vi "SBND_TST_p1_adc_1117.vi"() -> ()   [LabVIEW 2015]
uses:
  E:/P1_ADC_TEST_2017/LabVIEW_1130/LBNE_DLL/LBNE_DLL/bin/Debug/LBNE_DLL.dll
  <vilib>/Analysis/baseanly.llb/Mean (DBL).vi
  LBNE_Global .vi
  <vilib>/express/express analysis/Spectral/Block/exnSpectralBlock spectral measurements power poly.vi
  <vilib>/express/express analysis/Spectral/Block/exnSpectralBlock spectral measurements power DDT.vi
  <vilib>/express/express analysis/Spectral/XNode/ExpressSpectralMeasurementsBlockNode.xnode
  <vilib>/Analysis/NI_AAL_SigProc.lvlib
  <vilib>/Analysis/NI_AALBase.lvlib
panel:
  out "20":u16=100
  out "33":u16=3
  out "32":u16=10
  out "31":u16=90
  out "30":u16=32
  out "29":u16=10
  out "28":u16=10
  out "27":u16=90
  out "26":u16=60
  out "25":u16=40
  out "24":u16=6
  out "23":u16=92
  out "22":u16=12
  out "21":u16
  out "(hi.lo)":u16 format="%x"
  out "array":bool[](array[boolean])=[TRUE, FALSE, FALSE, TRUE, FALSE, FALSE, FALSE, FALSE]
  out "FE RB":u32[](array[numeric])=[4294901760, 4294901760, 4294901760, 4294901760, 4294901760, 4294901760, 4294901760, 4294901760, 4294901760, 4294901760, 4294901760, 4294901760, 4294901760, 4294901760, 4294901760, 4294901760, 4294901760, 4294901760, 4294901760, 4294901760, 4294901760, 4294901760, 4294901760, 4294901760, 4294901760, 4294901760, 4294901760, 4294901760, 4294901760, 4294901760, 4294901760, 4294901760, 4294901760, 4294901760, 4294901760, 4294901760] format="%x"
  out "FE Input":u32[](array[numeric])=[3503345872, 3503345872, 3503345872, 3503345872, 3503345872, 3503345872, 3503345872, 3503345872, 151062785, 3503345872, 3503345872, 3503345872, 3503345872, 3503345872, 3503345872, 3503345872, 3503345872, 151062785, 3503345872, 3503345872, 3503345872, 3503345872, 3503345872, 3503345872, 3503345872, 3503345872, 151062785, 3503345872, 3503345872, 3503345872, 3503345872, 3503345872, 3503345872, 3503345872, 3503345872, 151062785] format="%x"
  out "ADC RB":u32[](array[numeric])=[514, 514, 514, 514, 514, 514, 514, 514, 37120, 0, 0, 0, 0, 0, 0, 0, 0, 37120, 0, 0, 0, 0, 0, 0, 0, 0, 37120, 0, 0, 0, 0, 0, 0, 0, 0, 37120] format="%x"
  out "ADC  Input":u32[](array[numeric])=[0, 0, 0, 0, 0, 0, 0, 0, 1216366720, 0, 0, 0, 0, 0, 0, 0, 0, 1216366720, 0, 0, 0, 0, 0, 0, 0, 0, 1216366720, 257, 257, 257, 257, 257, 257, 257, 257, 1216366720] format="%x"
  in  "Array 4":T1(array[cluster])=[{"EN_GR"=1, "CLKG"=2, "FRQC"=1, "F2"=0, "F1"=0}, {"EN_GR"=1, "CLKG"=2, "FRQC"=1, "F2"=0, "F1"=0}, {"EN_GR"=1, "CLKG"=2, "FRQC"=1, "F2"=0, "F1"=0}, {"EN_GR"=1, "CLKG"=2, "FRQC"=1, "F2"=0, "F1"=0}, {"EN_GR"=0, "CLKG"=2, "FRQC"=1, "F2"=0, "F1"=0}, {"EN_GR"=0, "CLKG"=2, "FRQC"=1, "F2"=0, "F1"=0}, {"EN_GR"=0, "CLKG"=2, "FRQC"=1, "F2"=0, "F1"=0}, {"EN_GR"=1, "CLKG"=2, "FRQC"=1, "F2"=0, "F1"=0}] {"F1" items=["FIFO write clock is the ADC write clock", "FIFO write clock is on pin IdxMp/n.  "]; "F2" items=["FIFO clock generator off", "FIFO clock generator  on."]; "FRQC" items=["1 MHz", "2 MHz "]; "CLKG" items=["ADC clocks from monostable", "External clocks", "ADC clocks from digital generator of FIFO", "ADC clocks from monostable"]; "EN_GR" items=["Disables offset current absorption", "Enables the offset current absorption"]}
  out "size(s) 3":i32=127
  out "Array 5":dbl[](array[numeric])
  out "setting":u16=141
  out "Time has Elapsed":bool
  in  "y":i32=50
  out "ADC_hist":u32[][](array[numeric])
  out "FF_B_SHFT 2":u32=101058054 format="%x"
  out "TP_RES":u32=39341825
  out "Array 2":u32[](array[numeric])=[3503345872, 3503345872, 3503345872, 3503345872, 3503345872, 3503345872, 3503345872, 3503345872, 151062785, 3503345872, 3503345872, 3503345872, 3503345872, 3503345872, 3503345872, 3503345872, 3503345872, 151062785, 3503345872, 3503345872, 3503345872, 3503345872, 3503345872, 3503345872, 3503345872, 3503345872, 151062785, 3503345872, 3503345872, 3503345872, 3503345872, 3503345872, 3503345872, 3503345872, 3503345872, 151062785] format="%x"
  out "Array":u32[](array[numeric])=[0, 0, 0, 0, 0, 0, 0, 0, 1216366720, 0, 0, 0, 0, 0, 0, 0, 0, 1216366720, 0, 0, 0, 0, 0, 0, 0, 0, 1216366720, 257, 257, 257, 257, 257, 257, 257, 257, 1216366720] format="%x"
  out "FF_B_SHFT":u32=101058056 format="%x"
  in  "stop":bool
  in  "Tab Control":T2(tab)
  in  "Mult":dbl=1.0 format="%#_6p"
  in  "Pulse width(ns)":u32 max=1000000 step=20
  in  "Save":bool
  in  "DAC_MEAS":bool
  out "max value":u32=1719
  in  "RESET 6":bool
  in  "samples 3":i32
  in  "CHANNEL":u8(slide)
  in  "Tab Control 3":enum32{"CLOCK PHASE CONTROL"}(tab)
  in  "DATA SHIFT":u8[](array[numeric])=[8, 6, 6, 6, 6, 6, 6, 6] format="%x"
  in  "ADC_TM EN":bool=TRUE
  in  "TEST PAT":u32=279 format="%x"
  in  "TEST EN":u32 format="%x"
  out "result":u32=2165768192
  in  "ADC  CLK \nPHASE":bool[](array[boolean])=[TRUE, FALSE, FALSE, FALSE, TRUE, FALSE, TRUE, TRUE]
  in  "ASIC/CHN READOUT":bool=TRUE
  in  "number_of_samples":u32=10000
  in  "FREQ":u16=600
  in  "DLY":u8=79
  in  "AMPL":u8=1 format="%x"
  in  "CHIP":u8(slide) scale=0.0..7.0
  in  "STOP_DATA":bool
  in  "AUTO SCALE":bool=TRUE
  in  "x":u32=100
  out "ADC_MEAN":dbl=1719.0
  out "ADC_CNT":u32=37
  out "ADC_PEAK":u32=1719
  out "Waveform Graph 4":u32[](graph)
  out "ADC HIST":dynamicdata(graph)
  out "samples 4":u32=285743519
  out "Waveform Graph 5":u32[](graph)=[1719, 1718, 1719, 1717, 1719, 1717, 1718, 1717, 1718, 1719, 1718, 1717, 1718, 1716, 1717, 1718, 1717, 1717, 1717, 1717, 1718, 1719, 1718, 1717, 1719, 1719, 1719, 1717, 1718, 1717, 1716, 1719, 1718, 1717, 1717, 1719, 1717, 1718, 1717, 1719, 1716, 1718, 1717, 1718, 1717, 1718, 1717, 1718, 1717, 1718]
  in  "length":i32=50 min=10 max=65 step=1
  in  "SYNC":bool
  in  "FILE PATH":path=path "D:/debug_data"
  in  "FILE NAME 2":string="adaf2sd"
  in  "SAVE TO \nFILE":bool
  out "Store_Data":bool
  in  "SYNC 3":bool
  in  "recalu":bool
  out "samples":i32=10001
  in  "IntDAC_ON":bool
  out "x+y":u8=1 format="%b"
  in  "SYNC 2":bool
  in  "pulse_en":bool
  out "INV_REG":u16=3
  in  "invert 5":bool caption="INVERT"
  in  "invert 4":bool caption="invert"
  in  "invert 3":bool caption="invert"
  in  "invert 2":bool=TRUE caption="invert"
  in  "invert":bool=TRUE
  in  "LSB_S_OFF":dbl=4.4999999999999993e-07 caption="OFFSET" min=0.0 max=0.000655 step=1e-08 format="%#_6p"
  in  "LSB_S_WID":dbl=5e-08 caption="WIDTH" min=1e-08 max=0.000655 step=1e-08 format="%#_6p"
  in  "LSB_FC_OFF2":dbl=4.5e-07 caption="OFFSET" min=0.0 max=0.000655 step=1e-08 format="%#_6p"
  in  "LSB_FC_WID1":dbl=1.6e-07 caption="WIDTH" min=1e-08 max=0.000655 step=1e-08 format="%#_6p"
  in  "RD/EN_WID":dbl=3e-08 caption="WIDTH" min=1e-08 max=0.000655 step=1e-08 format="%#_6p"
  in  "LSB_FC_OFF1":dbl=5e-08 caption="OFFSET" min=0.0 max=0.000655 step=1e-08 format="%#_6p"
  in  "LSB_FC_WID2":dbl=5e-08 caption="WIDTH" min=1e-08 max=0.000655 step=1e-08 format="%#_6p"
  in  "PERIOD 2":dbl=5e-07 min=1e-08 max=0.000655 step=1e-08 format="%#_6p"
  in  "MSB_WID":dbl=3e-07 caption="WIDTH" min=1e-08 max=0.000655 step=1e-08 format="%#_6p"
  in  "MSB_OFF":dbl=2e-07 caption="OFFSET" min=0.0 max=0.000655 step=1e-08 format="%#_6p"
  in  "ADC_WID":dbl=6e-08 caption="WIDTH" min=1e-08 max=0.000655 step=1e-08 format="%#_6p"
  in  "ADC_OFF":dbl caption="OFFSET" min=0.0 max=0.000655 step=1e-08 format="%#_6p"
  in  "CLOCK":dbl=5e-09 format="%#_6p"
  in  "RD/EN_OFF":dbl=4.6e-07 caption="OFFSET" min=0.0 max=0.000655 step=1e-08 format="%#_6p"
  in  "Setting_ext_clk":bool
  in  "Reset":bool=TRUE
  out "Waveform Graph":dynamicdata(graph)=[{"t0"=timestamp(0 s since 1904-01-01), "dt"=199.98000199980004, "Y"=array[5001 elements], "attributes"=variant("NI_ChannelName"=variant(string "Power Spectrum"))}]
  in  "Boolean":bool=TRUE
  out "Peds Mean":dbl=18.0
  out "Peds_RMS":dbl
  in  "Restart Averaging":bool
  in  "fft save":bool=TRUE
  in  "Start channel":u8
  in  "Start chip":u8
  out "CUR_CHP":u8=8 caption="CHIP"
  out "CUR_CHN":u8 caption="CHANNEL"
  in  "Tab Control 2":enum32{"Page 1", "Page 2", "Page 3"}(tab)=enum."Page 2"
  out "Waveform Graph 6":u32[](graph)=[347, 344, 344, 344, 345, 347, 349, 350, 352, 351, 350, 350, 348, 349, 347, 350, 355, 674, 1968, 3349, 3455, 2112, 1599, 1721, 1728, 2759, 1820, 1126, 725, 547, 534, 612, 755, 755, 767, 750, 720, 699, 682, 677]
  out "ADC_CNT 2":u32=250000
  out "Waveform Graph 7":u32[](graph)
  out "CNT":i32
  in  "number_of_samples 2":u32=10000
  out "peds rms":dbl=13.663892227612275
  out "peds Mean":dbl=966.158
  out "ADC_MEAN 2":dbl=3547.568003950388
  out "ADC_RMS 2":dbl=28.577553542992373
  out "ENC":u32[][](array[numeric])=[[1066, 1158, 1012, 1088, 995, 1035, 1178, 1226, 0, 0, 0, 0, 0, 0, 0, 0], [1189, 1244, 1188, 920, 983, 1182, 1156, 1036, 0, 0, 0, 0, 0, 0, 0, 0], [998, 1190, 1140, 1203, 1082, 1076, 1156, 1019, 0, 0, 0, 0, 0, 0, 0, 0], [1218, 1198, 1231, 1210, 1128, 1046, 1135, 1285, 0, 0, 0, 0, 0, 0, 0, 0], [1111, 1144, 1123, 1107, 1274, 1033, 1249, 1045, 0, 0, 0, 0, 0, 0, 0, 0], [1232, 1074, 1188, 1225, 1224, 1163, 1150, 1045, 0, 0, 0, 0, 0, 0, 0, 0], [1135, 1231, 1161, 1158, 1204, 1187, 1007, 1210, 0, 0, 0, 0, 0, 0, 0, 0], [1167, 1176, 1273, 1200, 1029, 1106, 1193, 1134, 0, 0, 0, 0, 0, 0, 0, 0], [1193, 1078, 1088, 1147, 1057, 1218, 1117, 1152, 0, 0, 0, 0, 0, 0, 0, 0], [1139, 1255, 1171, 1006, 1142, 1231, 1182, 1110, 0, 0, 0, 0, 0, 0, 0, 0], [1022, 1243, 1182, 1152, 1182, 1227, 1034, 1008, 0, 0, 0, 0, 0, 0, 0, 0], [1097, 1118, 1072, 1073, 1076, 1190, 1129, 1021, 0, 0, 0, 0, 0, 0, 0, 0], [1180, 1434, 1174, 1222, 1134, 1076, 983, 961, 0, 0, 0, 0, 0, 0, 0, 0], [1246, 1138, 1204, 1072, 996, 1199, 1170, 1189, 0, 0, 0, 0, 0, 0, 0, 0], [1117, 1221, 1111, 1069, 1076, 1020, 1125, 1307, 0, 0, 0, 0, 0, 0, 0, 0], [1150, 1221, 1017, 1216, 1027, 1131, 1151, 1107, 0, 0, 0, 0, 0, 0, 0, 0]]
  out "RMS":dbl[][](array[numeric])=[[13.158810131795315, 14.299668256349447, 12.492235332772674, 13.434291139405659, 12.283790528144634, 12.773694837415796, 14.542669902822118, 15.129984571856891, 0.0, 0.0, 0.0, 0.0, 0.0, 0.0, 0.0, 0.0], [14.678913424572517, 15.352980350441642, 14.665580703900332, 11.355610563990915, 12.138665292767438, 14.589238842015973, 14.27260740231528, 12.784333020313527, 0.0, 0.0, 0.0, 0.0, 0.0, 0.0, 0.0, 0.0], [12.316104634769772, 14.686169938243747, 14.071507513514494, 14.850335266956211, 13.356531107153144, 13.286305287729014, 14.272524762853365, 12.585939548041432, 0.0, 0.0, 0.0, 0.0, 0.0, 0.0, 0.0, 0.0], [15.031876090654704, 14.78741307663375, 15.197331681388519, 14.942137963142448, 13.92969604991704, 12.916776312026833, 14.017775625421985, 15.861789423517077, 0.0, 0.0, 0.0, 0.0, 0.0, 0.0, 0.0, 0.0], [13.711007977448755, 14.124903893964802, 13.86214292900519, 13.669041429899488, 15.730185376637957, 12.757548988490175, 15.416399526623406, 12.90285640589203, 0.0, 0.0, 0.0, 0.0, 0.0, 0.0, 0.0, 0.0], [15.209968953932732, 13.253351507556122, 14.67011636123585, 15.11890588873142, 15.112163287188801, 14.361479615439631, 14.198048906716979, 12.907182040902331, 0.0, 0.0, 0.0, 0.0, 0.0, 0.0, 0.0, 0.0], [14.00645905304824, 15.192981506088497, 14.334865664637054, 14.29655500081451, 14.863929546227123, 14.648189450000741, 12.433031371901722, 14.93841649736285, 0.0, 0.0, 0.0, 0.0, 0.0, 0.0, 0.0, 0.0], [14.406934492960996, 14.521369254626054, 15.713725148777902, 14.816638937130847, 12.698558733540393, 13.65630718677371, 14.730008604397979, 14.000887735770736, 0.0, 0.0, 0.0, 0.0, 0.0, 0.0, 0.0, 0.0], [14.726953471809923, 13.307153473504258, 13.425939022614743, 14.159111250573732, 13.047276940761495, 15.032795841962947, 13.788303828391248, 14.216588987149647, 0.0, 0.0, 0.0, 0.0, 0.0, 0.0, 0.0, 0.0], [14.060310114619874, 15.497566502140451, 14.45258949361071, 12.414504608398772, 14.093800711961055, 15.193383167000526, 14.591254627573019, 13.700501782581963, 0.0, 0.0, 0.0, 0.0, 0.0, 0.0, 0.0, 0.0], [12.620986613202522, 15.34119284681887, 14.596673335246262, 14.228085214724398, 14.588330975790932, 15.14637178214725, 12.759404023095692, 12.44636167027054, 0.0, 0.0, 0.0, 0.0, 0.0, 0.0, 0.0, 0.0], [13.542240957742603, 13.796521505221467, 13.235895747990849, 13.24595461130884, 13.288907173806308, 14.693371316457617, 13.942789791470513, 12.605823223037053, 0.0, 0.0, 0.0, 0.0, 0.0, 0.0, 0.0, 0.0], [14.567227096150493, 17.700518696569162, 14.499408433524646, 15.089488052632309, 13.99466814342557, 13.28550840471075, 12.138577668930898, 11.868199777665112, 0.0, 0.0, 0.0, 0.0, 0.0, 0.0, 0.0, 0.0], [15.383401089361877, 14.0437627128782, 14.865354796421366, 13.236273748711483, 12.302313129985306, 14.80603646506271, 14.449664788619662, 14.684171701673126, 0.0, 0.0, 0.0, 0.0, 0.0, 0.0, 0.0, 0.0], [13.788793478982793, 15.074520898020795, 13.714749170015086, 13.194651442199076, 13.287129102811642, 12.589358859141534, 13.891878034502772, 16.13217079683144, 0.0, 0.0, 0.0, 0.0, 0.0, 0.0, 0.0, 0.0], [14.194393496869207, 14.58553882593015, 12.561266269833073, 15.01194166987972, 12.684919097973044, 13.95782081566281, 14.211606275556221, 13.663892227612275, 0.0, 0.0, 0.0, 0.0, 0.0, 0.0, 0.0, 0.0]] format="%#_6p"
  out "MEAN":dbl[][](array[numeric])=[[951.324636, 1011.55798, 971.46512, 1001.66468, 968.556052, 972.350264, 982.554388, 977.525348, 0.0, 0.0, 0.0, 0.0, 0.0, 0.0, 0.0, 0.0], [968.791648, 997.257824, 952.538196, 967.293388, 974.391288, 923.371776, 967.966284, 965.50768, 0.0, 0.0, 0.0, 0.0, 0.0, 0.0, 0.0, 0.0], [966.960944, 1017.868124, 981.59792, 999.453604, 946.836188, 936.086336, 945.20444, 959.828888, 0.0, 0.0, 0.0, 0.0, 0.0, 0.0, 0.0, 0.0], [978.26338, 1043.011188, 949.993868, 964.42902, 957.316784, 950.378752, 979.645384, 934.216884, 0.0, 0.0, 0.0, 0.0, 0.0, 0.0, 0.0, 0.0], [929.989036, 1032.178852, 966.136316, 986.937408, 946.225756, 967.610864, 953.010968, 978.696088, 0.0, 0.0, 0.0, 0.0, 0.0, 0.0, 0.0, 0.0], [929.028032, 1024.033592, 975.532416, 969.967212, 946.246792, 962.814236, 963.491192, 925.32462, 0.0, 0.0, 0.0, 0.0, 0.0, 0.0, 0.0, 0.0], [900.810692, 1016.34432, 957.256952, 971.032568, 951.10148, 974.453052, 971.472628, 976.797908, 0.0, 0.0, 0.0, 0.0, 0.0, 0.0, 0.0, 0.0], [904.885524, 1025.378384, 979.768964, 963.671816, 921.32862, 935.616876, 951.336824, 954.797924, 0.0, 0.0, 0.0, 0.0, 0.0, 0.0, 0.0, 0.0], [946.570576, 978.304044, 982.728128, 961.54466, 934.350396, 941.809608, 934.119708, 956.873992, 0.0, 0.0, 0.0, 0.0, 0.0, 0.0, 0.0, 0.0], [944.1745, 1004.2861, 977.463388, 964.074912, 934.10018, 936.20658, 957.856724, 945.618092, 0.0, 0.0, 0.0, 0.0, 0.0, 0.0, 0.0, 0.0], [973.670476, 982.029248, 954.42366, 975.224724, 923.454628, 929.649464, 976.710324, 968.553636, 0.0, 0.0, 0.0, 0.0, 0.0, 0.0, 0.0, 0.0], [965.06046, 898.844772, 965.280992, 974.93758, 917.347224, 921.535312, 966.193304, 960.837284, 0.0, 0.0, 0.0, 0.0, 0.0, 0.0, 0.0, 0.0], [950.01384, 992.454184, 956.749904, 943.244992, 952.055344, 933.469464, 965.61666, 962.037436, 0.0, 0.0, 0.0, 0.0, 0.0, 0.0, 0.0, 0.0], [930.076456, 1022.444884, 969.01946, 944.750212, 957.989368, 920.209564, 958.431424, 951.790124, 0.0, 0.0, 0.0, 0.0, 0.0, 0.0, 0.0, 0.0], [927.998292, 992.330316, 944.414212, 937.281776, 943.311696, 914.253672, 936.52954, 980.55764, 0.0, 0.0, 0.0, 0.0, 0.0, 0.0, 0.0, 0.0], [937.546208, 992.701584, 949.3722, 922.113264, 923.434524, 924.734336, 914.765328, 966.158, 0.0, 0.0, 0.0, 0.0, 0.0, 0.0, 0.0, 0.0]] format="%#_6p"
  out "samples received":i32=260051
  out "Average of all CHNS":dbl=1135.9057710689235
  out "gain electrons":u16=148
  out "FFT Analysis":dynamicdata(graph)=[{"t0"=timestamp(0 s since 1904-01-01), "dt"=400.0, "Y"=array[2500 elements], "attributes"=variant("NI_ChannelName"=variant(string "Power Spectrum"))}]
  in  "START":bool
  in  "FILE PATH 2":path=path "D:/ProtoDUNE_AM3/data0831/RMS"
  in  "FILE NAME 3":string="v6_" caption="FILE NAME 2"
  in  "SAVE TO \nFILE 2":bool
  in  "stop 2":bool
  out "samples 5":u32=261950 caption="SAMPLES"
  out "TP enable":bool
  out "AMPL 2":u8 format="%x"
  out "Store_Data 2":bool
  in  "com":u32=30
  in  "FREQ 2":u16=300
  in  "Caculation":u32=200
  in  "FILE NAME 4":string="FFT_" caption="FFTFILE NAME 2"
  out "loop cnt":i32=18865
  in  "AMPL2 END":i32 format="%x"
  in  "ADC write":bool=TRUE
  in  "DAC  0x00-0x3f":u16 format="%x"
  in  "DAC SW":u16(ring) items=["DISABLE TEST PULSE", "INTERNAL DAC", "EXTERNAL DAC", "DAC OUTPUT"]
  in  "DAC":u16[](array[numeric])=[16, 16, 16, 16, 16, 16, 16, 16] format="%x"
  in  "SW":u16[](array[ring])=[1, 1, 1, 1, 1, 1, 1, 1] items=["DISABLE TEST PULSE", "INTERNAL DAC", "EXTERNAL DAC", "DAC OUTPUT"]
  in  "FE ASIC(DAC)":bool=TRUE
  in  "ALL SET":bool
  in  "s 11":bool=TRUE
  in  "write_string":bool
  out "SDI 2":u16=16 format="%x"
  out "rst":u16=2
  out "cs":u16=4
  out "ck":u16=8
  out "SDI":u16=1
  in  "OK Button 2":bool
  in  "Slide":u8(slide)=3 scale=0.0..7.0
  in  "channel":T3={"sts"=TRUE, "snc"=TRUE, "SG"=2, "ST"=0, "SDC"=FALSE, "SDF"=FALSE} {"ST" items=["1us", "0.5us", "3us", "2us"]; "SG" items=["4.7 mV/fC", "7.8 mV/fC", "14 mV/fC", "25 mV/fC"]}
  in  "CHANNEL 4":T4={"D_offset"=0, "PDSR"=FALSE, "PCSR"=FALSE, "slp"=FALSE, "tst"=TRUE} {"D_offset" items=["0", "1", "2", "3", "4", "5", "6", "7", "8", "9", "10", "11", "12", "13", "14", "15"]}
  in  "QUICK SET":bool
  in  "s 10":bool=TRUE
  in  "s 9":bool=TRUE
  in  "s 8":bool=TRUE
  in  "s 7":bool=TRUE
  in  "s 6":bool=TRUE
  in  "s 5":bool=TRUE
  in  "s 4":bool=TRUE
  in  "s 3":bool=TRUE
  in  "s 2":bool=TRUE
  in  "s":bool=TRUE
  in  "CHANNEL 3":T5(array[cluster])=[[{"D_offset"=0, "PDSR"=FALSE, "PCSR"=FALSE, "slp"=FALSE, "tst"=FALSE}, {"D_offset"=0, "PDSR"=FALSE, "PCSR"=FALSE, "slp"=FALSE, "tst"=FALSE}, {"D_offset"=0, "PDSR"=FALSE, "PCSR"=FALSE, "slp"=FALSE, "tst"=FALSE}, {"D_offset"=0, "PDSR"=FALSE, "PCSR"=FALSE, "slp"=FALSE, "tst"=TRUE}, {"D_offset"=0, "PDSR"=FALSE, "PCSR"=FALSE, "slp"=FALSE, "tst"=FALSE}, {"D_offset"=0, "PDSR"=FALSE, "PCSR"=FALSE, "slp"=FALSE, "tst"=FALSE}, {"D_offset"=0, "PDSR"=FALSE, "PCSR"=FALSE, "slp"=FALSE, "tst"=FALSE}, {"D_offset"=0, "PDSR"=FALSE, "PCSR"=FALSE, "slp"=FALSE, "tst"=FALSE}], [{"D_offset"=0, "PDSR"=FALSE, "PCSR"=FALSE, "slp"=FALSE, "tst"=FALSE}, {"D_offset"=0, "PDSR"=FALSE, "PCSR"=FALSE, "slp"=FALSE, "tst"=FALSE}, {"D_offset"=0, "PDSR"=FALSE, "PCSR"=FALSE, "slp"=FALSE, "tst"=FALSE}, {"D_offset"=0, "PDSR"=FALSE, "PCSR"=FALSE, "slp"=FALSE, "tst"=TRUE}, {"D_offset"=0, "PDSR"=FALSE, "PCSR"=FALSE, "slp"=FALSE, "tst"=FALSE}, {"D_offset"=0, "PDSR"=FALSE, "PCSR"=FALSE, "slp"=FALSE, "tst"=FALSE}, {"D_offset"=0, "PDSR"=FALSE, "PCSR"=FALSE, "slp"=FALSE, "tst"=FALSE}, {"D_offset"=0, "PDSR"=FALSE, "PCSR"=FALSE, "slp"=FALSE, "tst"=FALSE}], [{"D_offset"=0, "PDSR"=FALSE, "PCSR"=FALSE, "slp"=FALSE, "tst"=FALSE}, {"D_offset"=0, "PDSR"=FALSE, "PCSR"=FALSE, "slp"=FALSE, "tst"=FALSE}, {"D_offset"=0, "PDSR"=FALSE, "PCSR"=FALSE, "slp"=FALSE, "tst"=FALSE}, {"D_offset"=0, "PDSR"=FALSE, "PCSR"=FALSE, "slp"=FALSE, "tst"=TRUE}, {"D_offset"=0, "PDSR"=FALSE, "PCSR"=FALSE, "slp"=FALSE, "tst"=FALSE}, {"D_offset"=0, "PDSR"=FALSE, "PCSR"=FALSE, "slp"=FALSE, "tst"=FALSE}, {"D_offset"=0, "PDSR"=FALSE, "PCSR"=FALSE, "slp"=FALSE, "tst"=FALSE}, {"D_offset"=0, "PDSR"=FALSE, "PCSR"=FALSE, "slp"=FALSE, "tst"=FALSE}], [{"D_offset"=0, "PDSR"=FALSE, "PCSR"=FALSE, "slp"=FALSE, "tst"=FALSE}, {"D_offset"=0, "PDSR"=FALSE, "PCSR"=FALSE, "slp"=FALSE, "tst"=FALSE}, {"D_offset"=0, "PDSR"=FALSE, "PCSR"=FALSE, "slp"=FALSE, "tst"=FALSE}, {"D_offset"=0, "PDSR"=FALSE, "PCSR"=FALSE, "slp"=FALSE, "tst"=TRUE}, {"D_offset"=0, "PDSR"=FALSE, "PCSR"=FALSE, "slp"=FALSE, "tst"=FALSE}, {"D_offset"=0, "PDSR"=FALSE, "PCSR"=FALSE, "slp"=FALSE, "tst"=FALSE}, {"D_offset"=0, "PDSR"=FALSE, "PCSR"=FALSE, "slp"=FALSE, "tst"=FALSE}, {"D_offset"=0, "PDSR"=FALSE, "PCSR"=FALSE, "slp"=FALSE, "tst"=FALSE}], [{"D_offset"=0, "PDSR"=FALSE, "PCSR"=FALSE, "slp"=FALSE, "tst"=FALSE}, {"D_offset"=0, "PDSR"=FALSE, "PCSR"=FALSE, "slp"=FALSE, "tst"=FALSE}, {"D_offset"=0, "PDSR"=FALSE, "PCSR"=FALSE, "slp"=FALSE, "tst"=FALSE}, {"D_offset"=0, "PDSR"=FALSE, "PCSR"=FALSE, "slp"=FALSE, "tst"=TRUE}, {"D_offset"=0, "PDSR"=FALSE, "PCSR"=FALSE, "slp"=FALSE, "tst"=FALSE}, {"D_offset"=0, "PDSR"=FALSE, "PCSR"=FALSE, "slp"=FALSE, "tst"=FALSE}, {"D_offset"=0, "PDSR"=FALSE, "PCSR"=FALSE, "slp"=FALSE, "tst"=FALSE}, {"D_offset"=0, "PDSR"=FALSE, "PCSR"=FALSE, "slp"=FALSE, "tst"=FALSE}], [{"D_offset"=0, "PDSR"=FALSE, "PCSR"=FALSE, "slp"=FALSE, "tst"=FALSE}, {"D_offset"=0, "PDSR"=FALSE, "PCSR"=FALSE, "slp"=FALSE, "tst"=FALSE}, {"D_offset"=0, "PDSR"=FALSE, "PCSR"=FALSE, "slp"=FALSE, "tst"=FALSE}, {"D_offset"=0, "PDSR"=FALSE, "PCSR"=FALSE, "slp"=FALSE, "tst"=TRUE}, {"D_offset"=0, "PDSR"=FALSE, "PCSR"=FALSE, "slp"=FALSE, "tst"=FALSE}, {"D_offset"=0, "PDSR"=FALSE, "PCSR"=FALSE, "slp"=FALSE, "tst"=FALSE}, {"D_offset"=0, "PDSR"=FALSE, "PCSR"=FALSE, "slp"=FALSE, "tst"=FALSE}, {"D_offset"=0, "PDSR"=FALSE, "PCSR"=FALSE, "slp"=FALSE, "tst"=FALSE}], [{"D_offset"=0, "PDSR"=FALSE, "PCSR"=FALSE, "slp"=FALSE, "tst"=FALSE}, {"D_offset"=0, "PDSR"=FALSE, "PCSR"=FALSE, "slp"=FALSE, "tst"=FALSE}, {"D_offset"=0, "PDSR"=FALSE, "PCSR"=FALSE, "slp"=FALSE, "tst"=FALSE}, {"D_offset"=0, "PDSR"=FALSE, "PCSR"=FALSE, "slp"=FALSE, "tst"=TRUE}, {"D_offset"=0, "PDSR"=FALSE, "PCSR"=FALSE, "slp"=FALSE, "tst"=FALSE}, {"D_offset"=0, "PDSR"=FALSE, "PCSR"=FALSE, "slp"=FALSE, "tst"=FALSE}, {"D_offset"=0, "PDSR"=FALSE, "PCSR"=FALSE, "slp"=FALSE, "tst"=FALSE}, {"D_offset"=0, "PDSR"=FALSE, "PCSR"=FALSE, "slp"=FALSE, "tst"=FALSE}], [{"D_offset"=0, "PDSR"=FALSE, "PCSR"=FALSE, "slp"=FALSE, "tst"=FALSE}, {"D_offset"=0, "PDSR"=FALSE, "PCSR"=FALSE, "slp"=FALSE, "tst"=FALSE}, {"D_offset"=0, "PDSR"=FALSE, "PCSR"=FALSE, "slp"=FALSE, "tst"=FALSE}, {"D_offset"=0, "PDSR"=FALSE, "PCSR"=FALSE, "slp"=FALSE, "tst"=TRUE}, {"D_offset"=0, "PDSR"=FALSE, "PCSR"=FALSE, "slp"=FALSE, "tst"=FALSE}, {"D_offset"=0, "PDSR"=FALSE, "PCSR"=FALSE, "slp"=FALSE, "tst"=FALSE}, {"D_offset"=0, "PDSR"=FALSE, "PCSR"=FALSE, "slp"=FALSE, "tst"=FALSE}, {"D_offset"=0, "PDSR"=FALSE, "PCSR"=FALSE, "slp"=FALSE, "tst"=FALSE}], [{"D_offset"=0, "PDSR"=FALSE, "PCSR"=FALSE, "slp"=FALSE, "tst"=FALSE}, {"D_offset"=0, "PDSR"=FALSE, "PCSR"=FALSE, "slp"=FALSE, "tst"=FALSE}, {"D_offset"=0, "PDSR"=FALSE, "PCSR"=FALSE, "slp"=FALSE, "tst"=FALSE}, {"D_offset"=0, "PDSR"=FALSE, "PCSR"=FALSE, "slp"=FALSE, "tst"=TRUE}, {"D_offset"=0, "PDSR"=FALSE, "PCSR"=FALSE, "slp"=FALSE, "tst"=FALSE}, {"D_offset"=0, "PDSR"=FALSE, "PCSR"=FALSE, "slp"=FALSE, "tst"=FALSE}, {"D_offset"=0, "PDSR"=FALSE, "PCSR"=FALSE, "slp"=FALSE, "tst"=FALSE}, {"D_offset"=0, "PDSR"=FALSE, "PCSR"=FALSE, "slp"=FALSE, "tst"=FALSE}], [{"D_offset"=0, "PDSR"=FALSE, "PCSR"=FALSE, "slp"=FALSE, "tst"=FALSE}, {"D_offset"=0, "PDSR"=FALSE, "PCSR"=FALSE, "slp"=FALSE, "tst"=FALSE}, {"D_offset"=0, "PDSR"=FALSE, "PCSR"=FALSE, "slp"=FALSE, "tst"=FALSE}, {"D_offset"=0, "PDSR"=FALSE, "PCSR"=FALSE, "slp"=FALSE, "tst"=TRUE}, {"D_offset"=0, "PDSR"=FALSE, "PCSR"=FALSE, "slp"=FALSE, "tst"=FALSE}, {"D_offset"=0, "PDSR"=FALSE, "PCSR"=FALSE, "slp"=FALSE, "tst"=FALSE}, {"D_offset"=0, "PDSR"=FALSE, "PCSR"=FALSE, "slp"=FALSE, "tst"=FALSE}, {"D_offset"=0, "PDSR"=FALSE, "PCSR"=FALSE, "slp"=FALSE, "tst"=FALSE}], [{"D_offset"=0, "PDSR"=FALSE, "PCSR"=FALSE, "slp"=FALSE, "tst"=FALSE}, {"D_offset"=0, "PDSR"=FALSE, "PCSR"=FALSE, "slp"=FALSE, "tst"=FALSE}, {"D_offset"=0, "PDSR"=FALSE, "PCSR"=FALSE, "slp"=FALSE, "tst"=FALSE}, {"D_offset"=0, "PDSR"=FALSE, "PCSR"=FALSE, "slp"=FALSE, "tst"=TRUE}, {"D_offset"=0, "PDSR"=FALSE, "PCSR"=FALSE, "slp"=FALSE, "tst"=FALSE}, {"D_offset"=0, "PDSR"=FALSE, "PCSR"=FALSE, "slp"=FALSE, "tst"=FALSE}, {"D_offset"=0, "PDSR"=FALSE, "PCSR"=FALSE, "slp"=FALSE, "tst"=FALSE}, {"D_offset"=0, "PDSR"=FALSE, "PCSR"=FALSE, "slp"=FALSE, "tst"=FALSE}], [{"D_offset"=0, "PDSR"=FALSE, "PCSR"=FALSE, "slp"=FALSE, "tst"=FALSE}, {"D_offset"=0, "PDSR"=FALSE, "PCSR"=FALSE, "slp"=FALSE, "tst"=FALSE}, {"D_offset"=0, "PDSR"=FALSE, "PCSR"=FALSE, "slp"=FALSE, "tst"=FALSE}, {"D_offset"=0, "PDSR"=FALSE, "PCSR"=FALSE, "slp"=FALSE, "tst"=TRUE}, {"D_offset"=0, "PDSR"=FALSE, "PCSR"=FALSE, "slp"=FALSE, "tst"=FALSE}, {"D_offset"=0, "PDSR"=FALSE, "PCSR"=FALSE, "slp"=FALSE, "tst"=FALSE}, {"D_offset"=0, "PDSR"=FALSE, "PCSR"=FALSE, "slp"=FALSE, "tst"=FALSE}, {"D_offset"=0, "PDSR"=FALSE, "PCSR"=FALSE, "slp"=FALSE, "tst"=FALSE}], [{"D_offset"=0, "PDSR"=FALSE, "PCSR"=FALSE, "slp"=FALSE, "tst"=FALSE}, {"D_offset"=0, "PDSR"=FALSE, "PCSR"=FALSE, "slp"=FALSE, "tst"=FALSE}, {"D_offset"=0, "PDSR"=FALSE, "PCSR"=FALSE, "slp"=FALSE, "tst"=FALSE}, {"D_offset"=0, "PDSR"=FALSE, "PCSR"=FALSE, "slp"=FALSE, "tst"=TRUE}, {"D_offset"=0, "PDSR"=FALSE, "PCSR"=FALSE, "slp"=FALSE, "tst"=FALSE}, {"D_offset"=0, "PDSR"=FALSE, "PCSR"=FALSE, "slp"=FALSE, "tst"=FALSE}, {"D_offset"=0, "PDSR"=FALSE, "PCSR"=FALSE, "slp"=FALSE, "tst"=FALSE}, {"D_offset"=0, "PDSR"=FALSE, "PCSR"=FALSE, "slp"=FALSE, "tst"=FALSE}], [{"D_offset"=0, "PDSR"=FALSE, "PCSR"=FALSE, "slp"=FALSE, "tst"=FALSE}, {"D_offset"=0, "PDSR"=FALSE, "PCSR"=FALSE, "slp"=FALSE, "tst"=FALSE}, {"D_offset"=0, "PDSR"=FALSE, "PCSR"=FALSE, "slp"=FALSE, "tst"=FALSE}, {"D_offset"=0, "PDSR"=FALSE, "PCSR"=FALSE, "slp"=FALSE, "tst"=TRUE}, {"D_offset"=0, "PDSR"=FALSE, "PCSR"=FALSE, "slp"=FALSE, "tst"=FALSE}, {"D_offset"=0, "PDSR"=FALSE, "PCSR"=FALSE, "slp"=FALSE, "tst"=FALSE}, {"D_offset"=0, "PDSR"=FALSE, "PCSR"=FALSE, "slp"=FALSE, "tst"=FALSE}, {"D_offset"=0, "PDSR"=FALSE, "PCSR"=FALSE, "slp"=FALSE, "tst"=FALSE}], [{"D_offset"=0, "PDSR"=FALSE, "PCSR"=FALSE, "slp"=FALSE, "tst"=FALSE}, {"D_offset"=0, "PDSR"=FALSE, "PCSR"=FALSE, "slp"=FALSE, "tst"=FALSE}, {"D_offset"=0, "PDSR"=FALSE, "PCSR"=FALSE, "slp"=FALSE, "tst"=FALSE}, {"D_offset"=0, "PDSR"=FALSE, "PCSR"=FALSE, "slp"=FALSE, "tst"=TRUE}, {"D_offset"=0, "PDSR"=FALSE, "PCSR"=FALSE, "slp"=FALSE, "tst"=FALSE}, {"D_offset"=0, "PDSR"=FALSE, "PCSR"=FALSE, "slp"=FALSE, "tst"=FALSE}, {"D_offset"=0, "PDSR"=FALSE, "PCSR"=FALSE, "slp"=FALSE, "tst"=FALSE}, {"D_offset"=0, "PDSR"=FALSE, "PCSR"=FALSE, "slp"=FALSE, "tst"=FALSE}], [{"D_offset"=0, "PDSR"=FALSE, "PCSR"=FALSE, "slp"=FALSE, "tst"=FALSE}, {"D_offset"=0, "PDSR"=FALSE, "PCSR"=FALSE, "slp"=FALSE, "tst"=FALSE}, {"D_offset"=0, "PDSR"=FALSE, "PCSR"=FALSE, "slp"=FALSE, "tst"=FALSE}, {"D_offset"=0, "PDSR"=FALSE, "PCSR"=FALSE, "slp"=FALSE, "tst"=TRUE}, {"D_offset"=0, "PDSR"=FALSE, "PCSR"=FALSE, "slp"=FALSE, "tst"=FALSE}, {"D_offset"=0, "PDSR"=FALSE, "PCSR"=FALSE, "slp"=FALSE, "tst"=FALSE}, {"D_offset"=0, "PDSR"=FALSE, "PCSR"=FALSE, "slp"=FALSE, "tst"=FALSE}, {"D_offset"=0, "PDSR"=FALSE, "PCSR"=FALSE, "slp"=FALSE, "tst"=FALSE}]] {"D_offset" items=["0", "1", "2", "3", "4", "5", "6", "7", "8", "9", "10", "11", "12", "13", "14", "15"]}
  out "ADC ARRAY":bool[](array[boolean])=[FALSE, FALSE, FALSE, FALSE, FALSE, FALSE, FALSE, FALSE, FALSE, FALSE, FALSE, FALSE, FALSE, FALSE, FALSE, FALSE, FALSE, FALSE, FALSE, FALSE, FALSE, FALSE, FALSE, FALSE, FALSE, FALSE, FALSE, FALSE, FALSE, FALSE, FALSE, FALSE, FALSE, FALSE, FALSE, FALSE, FALSE, FALSE, FALSE, FALSE, FALSE, FALSE, FALSE, FALSE, FALSE, FALSE, FALSE, FALSE, FALSE, FALSE, FALSE, FALSE, FALSE, FALSE, FALSE, FALSE, FALSE, FALSE, FALSE, FALSE, FALSE, FALSE, FALSE, FALSE, FALSE, FALSE, FALSE, FALSE, FALSE, FALSE, FALSE, FALSE, FALSE, FALSE, FALSE, FALSE, FALSE, FALSE, FALSE, FALSE, FALSE, FALSE, FALSE, FALSE, FALSE, FALSE, FALSE, FALSE, FALSE, FALSE, FALSE, FALSE, FALSE, FALSE, FALSE, FALSE, FALSE, FALSE, FALSE, FALSE, FALSE, FALSE, FALSE, FALSE, FALSE, FALSE, FALSE, FALSE, FALSE, FALSE, FALSE, FALSE, FALSE, FALSE, FALSE, FALSE, FALSE, FALSE, FALSE, FALSE, FALSE, FALSE, FALSE, FALSE, FALSE, FALSE, FALSE, FALSE, FALSE, FALSE, FALSE, FALSE, FALSE, FALSE, FALSE, TRUE, FALSE, FALSE, FALSE, TRUE, FALSE, FALSE, TRUE, FALSE, FALSE, FALSE, FALSE, FALSE, FALSE, FALSE, FALSE, FALSE, FALSE, FALSE, FALSE, FALSE, FALSE, FALSE, FALSE, FALSE, FALSE, FALSE, FALSE, FALSE, FALSE, FALSE, FALSE, FALSE, FALSE, FALSE, FALSE, FALSE, FALSE, FALSE, FALSE, FALSE, FALSE, FALSE, FALSE, FALSE, FALSE, FALSE, FALSE, FALSE, FALSE, FALSE, FALSE, FALSE, FALSE, FALSE, FALSE, FALSE, FALSE, FALSE, FALSE, FALSE, FALSE, FALSE, FALSE, FALSE, FALSE, FALSE, FALSE, FALSE, FALSE, FALSE, FALSE, FALSE, FALSE, FALSE, FALSE, FALSE, FALSE, FALSE, FALSE, FALSE, FALSE, FALSE, FALSE, FALSE, FALSE, FALSE, FALSE, FALSE, FALSE, FALSE, FALSE, FALSE, FALSE, FALSE, FALSE, FALSE, FALSE, FALSE, FALSE, FALSE, FALSE, FALSE, FALSE, FALSE, FALSE, FALSE, FALSE, FALSE, FALSE, FALSE, FALSE, FALSE, FALSE, FALSE, FALSE, FALSE, FALSE, FALSE, FALSE, FALSE, FALSE, FALSE, FALSE, FALSE, FALSE, FALSE, FALSE, FALSE, FALSE, FALSE, FALSE, FALSE, FALSE, FALSE, FALSE, FALSE, FALSE, FALSE, FALSE, FALSE, FALSE, FALSE, FALSE, TRUE, FALSE, FALSE, FALSE, TRUE, FALSE, FALSE, TRUE, FALSE, FALSE, FALSE, FALSE, FALSE, FALSE, FALSE, FALSE, FALSE, FALSE, FALSE, FALSE, FALSE, FALSE, FALSE, FALSE, FALSE, FALSE, FALSE, FALSE, FALSE, FALSE, FALSE, FALSE, FALSE, FALSE, FALSE, FALSE, FALSE, FALSE, FALSE, FALSE, FALSE, FALSE, FALSE, FALSE, FALSE, FALSE, FALSE, FALSE, FALSE, FALSE, FALSE, FALSE, FALSE, FALSE, FALSE, FALSE, FALSE, FALSE, FALSE, FALSE, FALSE, FALSE, FALSE, FALSE, FALSE, FALSE, FALSE, FALSE, FALSE, FALSE, FALSE, FALSE, FALSE, FALSE, FALSE, FALSE, FALSE, FALSE, FALSE, FALSE, FALSE, FALSE, FALSE, FALSE, FALSE, FALSE, FALSE, FALSE, FALSE, FALSE, FALSE, FALSE, FALSE, FALSE, FALSE, FALSE, FALSE, FALSE, FALSE, FALSE, FALSE, FALSE, FALSE, FALSE, FALSE, FALSE, FALSE, FALSE, FALSE, FALSE, FALSE, FALSE, FALSE, FALSE, FALSE, FALSE, FALSE, FALSE, FALSE, FALSE, FALSE, FALSE, FALSE, FALSE, FALSE, FALSE, FALSE, FALSE, FALSE, FALSE, FALSE, FALSE, FALSE, FALSE, FALSE, FALSE, FALSE, FALSE, FALSE, FALSE, FALSE, FALSE, FALSE, FALSE, TRUE, FALSE, FALSE, FALSE, TRUE, FALSE, FALSE, TRUE, FALSE, TRUE, FALSE, FALSE, FALSE, FALSE, FALSE, FALSE, FALSE, TRUE, FALSE, FALSE, FALSE, FALSE, FALSE, FALSE, FALSE, TRUE, FALSE, FALSE, FALSE, FALSE, FALSE, FALSE, FALSE, TRUE, FALSE, FALSE, FALSE, FALSE, FALSE, FALSE, FALSE, TRUE, FALSE, FALSE, FALSE, FALSE, FALSE, FALSE, FALSE, TRUE, FALSE, FALSE, FALSE, FALSE, FALSE, FALSE, FALSE, TRUE, FALSE, FALSE, FALSE, FALSE, FALSE, FALSE, FALSE, TRUE, FALSE, FALSE, FALSE, FALSE, FALSE, FALSE, FALSE, TRUE, FALSE, FALSE, FALSE, FALSE, FALSE, FALSE, FALSE, TRUE, FALSE, FALSE, FALSE, FALSE, FALSE, FALSE, FALSE, TRUE, FALSE, FALSE, FALSE, FALSE, FALSE, FALSE, FALSE, TRUE, FALSE, FALSE, FALSE, FALSE, FALSE, FALSE, FALSE, TRUE, FALSE, FALSE, FALSE, FALSE, FALSE, FALSE, FALSE, TRUE, FALSE, FALSE, FALSE, FALSE, FALSE, FALSE, FALSE, TRUE, FALSE, FALSE, FALSE, FALSE, FALSE, FALSE, FALSE, TRUE, FALSE, FALSE, FALSE, FALSE, FALSE, FALSE, FALSE, FALSE, FALSE, FALSE, FALSE, FALSE, FALSE, FALSE, TRUE, FALSE, FALSE, FALSE, TRUE, FALSE, FALSE, TRUE, FALSE, FALSE, FALSE, FALSE, FALSE, FALSE, FALSE, FALSE, FALSE, FALSE, FALSE, FALSE, FALSE, FALSE, FALSE, FALSE, FALSE, FALSE, FALSE, FALSE, FALSE, FALSE, FALSE, FALSE, FALSE, FALSE, FALSE, FALSE, FALSE, FALSE, FALSE, FALSE, FALSE, FALSE, FALSE, FALSE, FALSE, FALSE, FALSE, FALSE, FALSE, FALSE, FALSE, FALSE, FALSE, FALSE, FALSE, FALSE, FALSE, FALSE, FALSE, FALSE, FALSE, FALSE, FALSE, FALSE, FALSE, FALSE, FALSE, FALSE, FALSE, FALSE, FALSE, FALSE, FALSE, FALSE, FALSE, FALSE, FALSE, FALSE, FALSE, FALSE, FALSE, FALSE, FALSE, FALSE, FALSE, FALSE, FALSE, FALSE, FALSE, FALSE, FALSE, FALSE, FALSE, FALSE, FALSE, FALSE, FALSE, FALSE, FALSE, FALSE, FALSE, FALSE, FALSE, FALSE, FALSE, FALSE, FALSE, FALSE, FALSE, FALSE, FALSE, FALSE, FALSE, FALSE, FALSE, FALSE, FALSE, FALSE, FALSE, FALSE, FALSE, FALSE, FALSE, FALSE, FALSE, FALSE, FALSE, FALSE, FALSE, FALSE, FALSE, FALSE, FALSE, FALSE, FALSE, FALSE, FALSE, FALSE, FALSE, FALSE, FALSE, FALSE, FALSE, FALSE, TRUE, FALSE, FALSE, FALSE, TRUE, FALSE, FALSE, TRUE, FALSE, FALSE, FALSE, FALSE, FALSE, FALSE, FALSE, FALSE, FALSE, FALSE, FALSE, FALSE, FALSE, FALSE, FALSE, FALSE, FALSE, FALSE, FALSE, FALSE, FALSE, FALSE, FALSE, FALSE, FALSE, FALSE, FALSE, FALSE, FALSE, FALSE, FALSE, FALSE, FALSE, FALSE, FALSE, FALSE, FALSE, FALSE, FALSE, FALSE, FALSE, FALSE, FALSE, FALSE, FALSE, FALSE, FALSE, FALSE, FALSE, FALSE, FALSE, FALSE, FALSE, FALSE, FALSE, FALSE, FALSE, FALSE, FALSE, FALSE, FALSE, FALSE, FALSE, FALSE, FALSE, FALSE, FALSE, FALSE, FALSE, FALSE, FALSE, FALSE, FALSE, FALSE, FALSE, FALSE, FALSE, FALSE, FALSE, FALSE, FALSE, FALSE, FALSE, FALSE, FALSE, FALSE, FALSE, FALSE, FALSE, FALSE, FALSE, FALSE, FALSE, FALSE, FALSE, FALSE, FALSE, FALSE, FALSE, FALSE, FALSE, FALSE, FALSE, FALSE, FALSE, FALSE, FALSE, FALSE, FALSE, FALSE, FALSE, FALSE, FALSE, FALSE, FALSE, FALSE, FALSE, FALSE, FALSE, FALSE, FALSE, FALSE, FALSE, FALSE, FALSE, FALSE, FALSE, FALSE, FALSE, FALSE, FALSE, FALSE, FALSE, FALSE, FALSE, FALSE, TRUE, FALSE, FALSE, FALSE, TRUE, FALSE, FALSE, TRUE, FALSE, FALSE, FALSE, FALSE, FALSE, FALSE, FALSE, FALSE, FALSE, FALSE, FALSE, FALSE, FALSE, FALSE, FALSE, FALSE, FALSE, FALSE, FALSE, FALSE, FALSE, FALSE, FALSE, FALSE, FALSE, FALSE, FALSE, FALSE, FALSE, FALSE, FALSE, FALSE, FALSE, FALSE, FALSE, FALSE, FALSE, FALSE, FALSE, FALSE, FALSE, FALSE, FALSE, FALSE, FALSE, FALSE, FALSE, FALSE, FALSE, FALSE, FALSE, FALSE, FALSE, FALSE, FALSE, FALSE, FALSE, FALSE, FALSE, FALSE, FALSE, FALSE, FALSE, FALSE, FALSE, FALSE, FALSE, FALSE, FALSE, FALSE, FALSE, FALSE, FALSE, FALSE, FALSE, FALSE, FALSE, FALSE, FALSE, FALSE, FALSE, FALSE, FALSE, FALSE, FALSE, FALSE, FALSE, FALSE, FALSE, FALSE, FALSE, FALSE, FALSE, FALSE, FALSE, FALSE, FALSE, FALSE, FALSE, FALSE, FALSE, FALSE, FALSE, FALSE, FALSE, FALSE, FALSE, FALSE, FALSE, FALSE, FALSE, FALSE, FALSE, FALSE, FALSE, FALSE, FALSE, FALSE, FALSE, FALSE, FALSE, FALSE, FALSE, FALSE, FALSE, FALSE, FALSE, FALSE, FALSE, FALSE, FALSE, FALSE, FALSE, FALSE, FALSE, FALSE, TRUE, FALSE, FALSE, FALSE, TRUE, FALSE, FALSE, TRUE, FALSE, FALSE, FALSE, FALSE, FALSE, FALSE, FALSE, FALSE, FALSE, FALSE, FALSE, FALSE, FALSE, FALSE, FALSE, FALSE, FALSE, FALSE, FALSE, FALSE, FALSE, FALSE, FALSE, FALSE, FALSE, FALSE, FALSE, FALSE, FALSE, FALSE, FALSE, FALSE, FALSE, FALSE, FALSE, FALSE, FALSE, FALSE, FALSE, FALSE, FALSE, FALSE, FALSE, FALSE, FALSE, FALSE, FALSE, FALSE, FALSE, FALSE, FALSE, FALSE, FALSE, FALSE, FALSE, FALSE, FALSE, FALSE, FALSE, FALSE, FALSE, FALSE, FALSE, FALSE, FALSE, FALSE, FALSE, FALSE, FALSE, FALSE, FALSE, FALSE, FALSE, FALSE, FALSE, FALSE, FALSE, FALSE, FALSE, FALSE, FALSE, FALSE, FALSE, FALSE, FALSE, FALSE, FALSE, FALSE, FALSE, FALSE, FALSE, FALSE, FALSE, FALSE, FALSE, FALSE, FALSE, FALSE, FALSE, FALSE, FALSE, FALSE, FALSE, FALSE, FALSE, FALSE, FALSE, FALSE, FALSE, FALSE, FALSE, FALSE, FALSE, FALSE, FALSE, FALSE, FALSE, FALSE, FALSE, FALSE, FALSE, FALSE, FALSE, FALSE, FALSE, FALSE, FALSE, FALSE, FALSE, FALSE, FALSE, FALSE, FALSE, FALSE, FALSE, FALSE, TRUE, FALSE, FALSE, FALSE, TRUE, FALSE, FALSE, TRUE, FALSE]
  out "FE ARRAY":bool[](array[boolean])=[FALSE, FALSE, FALSE, FALSE, TRUE, FALSE, TRUE, TRUE, FALSE, FALSE, FALSE, FALSE, TRUE, FALSE, TRUE, TRUE, FALSE, FALSE, FALSE, FALSE, TRUE, FALSE, TRUE, TRUE, FALSE, FALSE, FALSE, FALSE, TRUE, FALSE, TRUE, TRUE, FALSE, FALSE, FALSE, FALSE, TRUE, FALSE, TRUE, TRUE, FALSE, FALSE, FALSE, FALSE, TRUE, FALSE, TRUE, TRUE, FALSE, FALSE, FALSE, FALSE, TRUE, FALSE, TRUE, TRUE, FALSE, FALSE, FALSE, FALSE, TRUE, FALSE, TRUE, TRUE, FALSE, FALSE, FALSE, FALSE, TRUE, FALSE, TRUE, TRUE, FALSE, FALSE, FALSE, FALSE, TRUE, FALSE, TRUE, TRUE, FALSE, FALSE, FALSE, FALSE, TRUE, FALSE, TRUE, TRUE, FALSE, FALSE, FALSE, FALSE, TRUE, FALSE, TRUE, TRUE, FALSE, FALSE, FALSE, FALSE, TRUE, FALSE, TRUE, TRUE, FALSE, FALSE, FALSE, FALSE, TRUE, FALSE, TRUE, TRUE, FALSE, FALSE, FALSE, FALSE, TRUE, FALSE, TRUE, TRUE, FALSE, FALSE, FALSE, FALSE, TRUE, FALSE, TRUE, TRUE, TRUE, FALSE, FALSE, FALSE, FALSE, FALSE, FALSE, FALSE, TRUE, FALSE, FALSE, TRUE, FALSE, FALSE, FALSE, FALSE, FALSE, FALSE, FALSE, FALSE, TRUE, FALSE, TRUE, TRUE, FALSE, FALSE, FALSE, FALSE, TRUE, FALSE, TRUE, TRUE, FALSE, FALSE, FALSE, FALSE, TRUE, FALSE, TRUE, TRUE, FALSE, FALSE, FALSE, FALSE, TRUE, FALSE, TRUE, TRUE, FALSE, FALSE, FALSE, FALSE, TRUE, FALSE, TRUE, TRUE, FALSE, FALSE, FALSE, FALSE, TRUE, FALSE, TRUE, TRUE, FALSE, FALSE, FALSE, FALSE, TRUE, FALSE, TRUE, TRUE, FALSE, FALSE, FALSE, FALSE, TRUE, FALSE, TRUE, TRUE, FALSE, FALSE, FALSE, FALSE, TRUE, FALSE, TRUE, TRUE, FALSE, FALSE, FALSE, FALSE, TRUE, FALSE, TRUE, TRUE, FALSE, FALSE, FALSE, FALSE, TRUE, FALSE, TRUE, TRUE, FALSE, FALSE, FALSE, FALSE, TRUE, FALSE, TRUE, TRUE, FALSE, FALSE, FALSE, FALSE, TRUE, FALSE, TRUE, TRUE, FALSE, FALSE, FALSE, FALSE, TRUE, FALSE, TRUE, TRUE, FALSE, FALSE, FALSE, FALSE, TRUE, FALSE, TRUE, TRUE, FALSE, FALSE, FALSE, FALSE, TRUE, FALSE, TRUE, TRUE, TRUE, FALSE, FALSE, FALSE, FALSE, FALSE, FALSE, FALSE, TRUE, FALSE, FALSE, TRUE, FALSE, FALSE, FALSE, FALSE, FALSE, FALSE, FALSE, FALSE, TRUE, FALSE, TRUE, TRUE, FALSE, FALSE, FALSE, FALSE, TRUE, FALSE, TRUE, TRUE, FALSE, FALSE, FALSE, FALSE, TRUE, FALSE, TRUE, TRUE, FALSE, FALSE, FALSE, FALSE, TRUE, FALSE, TRUE, TRUE, FALSE, FALSE, FALSE, FALSE, TRUE, FALSE, TRUE, TRUE, FALSE, FALSE, FALSE, FALSE, TRUE, FALSE, TRUE, TRUE, FALSE, FALSE, FALSE, FALSE, TRUE, FALSE, TRUE, TRUE, FALSE, FALSE, FALSE, FALSE, TRUE, FALSE, TRUE, TRUE, FALSE, FALSE, FALSE, FALSE, TRUE, FALSE, TRUE, TRUE, FALSE, FALSE, FALSE, FALSE, TRUE, FALSE, TRUE, TRUE, FALSE, FALSE, FALSE, FALSE, TRUE, FALSE, TRUE, TRUE, FALSE, FALSE, FALSE, FALSE, TRUE, FALSE, TRUE, TRUE, FALSE, FALSE, FALSE, FALSE, TRUE, FALSE, TRUE, TRUE, FALSE, FALSE, FALSE, FALSE, TRUE, FALSE, TRUE, TRUE, FALSE, FALSE, FALSE, FALSE, TRUE, FALSE, TRUE, TRUE, FALSE, FALSE, FALSE, FALSE, TRUE, FALSE, TRUE, TRUE, TRUE, FALSE, FALSE, FALSE, FALSE, FALSE, FALSE, FALSE, TRUE, FALSE, FALSE, TRUE, FALSE, FALSE, FALSE, FALSE, FALSE, FALSE, FALSE, FALSE, TRUE, FALSE, TRUE, TRUE, FALSE, FALSE, FALSE, FALSE, TRUE, FALSE, TRUE, TRUE, FALSE, FALSE, FALSE, FALSE, TRUE, FALSE, TRUE, TRUE, FALSE, FALSE, FALSE, FALSE, TRUE, FALSE, TRUE, TRUE, FALSE, FALSE, FALSE, FALSE, TRUE, FALSE, TRUE, TRUE, FALSE, FALSE, FALSE, FALSE, TRUE, FALSE, TRUE, TRUE, FALSE, FALSE, FALSE, FALSE, TRUE, FALSE, TRUE, TRUE, FALSE, FALSE, FALSE, FALSE, TRUE, FALSE, TRUE, TRUE, FALSE, FALSE, FALSE, FALSE, TRUE, FALSE, TRUE, TRUE, FALSE, FALSE, FALSE, FALSE, TRUE, FALSE, TRUE, TRUE, FALSE, FALSE, FALSE, FALSE, TRUE, FALSE, TRUE, TRUE, FALSE, FALSE, FALSE, FALSE, TRUE, FALSE, TRUE, TRUE, FALSE, FALSE, FALSE, FALSE, TRUE, FALSE, TRUE, TRUE, FALSE, FALSE, FALSE, FALSE, TRUE, FALSE, TRUE, TRUE, FALSE, FALSE, FALSE, FALSE, TRUE, FALSE, TRUE, TRUE, FALSE, FALSE, FALSE, FALSE, TRUE, FALSE, TRUE, TRUE, TRUE, FALSE, FALSE, FALSE, FALSE, FALSE, FALSE, FALSE, TRUE, FALSE, FALSE, TRUE, FALSE, FALSE, FALSE, FALSE, FALSE, FALSE, FALSE, FALSE, TRUE, FALSE, TRUE, TRUE, FALSE, FALSE, FALSE, FALSE, TRUE, FALSE, TRUE, TRUE, FALSE, FALSE, FALSE, FALSE, TRUE, FALSE, TRUE, TRUE, FALSE, FALSE, FALSE, FALSE, TRUE, FALSE, TRUE, TRUE, FALSE, FALSE, FALSE, FALSE, TRUE, FALSE, TRUE, TRUE, FALSE, FALSE, FALSE, FALSE, TRUE, FALSE, TRUE, TRUE, FALSE, FALSE, FALSE, FALSE, TRUE, FALSE, TRUE, TRUE, FALSE, FALSE, FALSE, FALSE, TRUE, FALSE, TRUE, TRUE, FALSE, FALSE, FALSE, FALSE, TRUE, FALSE, TRUE, TRUE, FALSE, FALSE, FALSE, FALSE, TRUE, FALSE, TRUE, TRUE, FALSE, FALSE, FALSE, FALSE, TRUE, FALSE, TRUE, TRUE, FALSE, FALSE, FALSE, FALSE, TRUE, FALSE, TRUE, TRUE, FALSE, FALSE, FALSE, FALSE, TRUE, FALSE, TRUE, TRUE, FALSE, FALSE, FALSE, FALSE, TRUE, FALSE, TRUE, TRUE, FALSE, FALSE, FALSE, FALSE, TRUE, FALSE, TRUE, TRUE, FALSE, FALSE, FALSE, FALSE, TRUE, FALSE, TRUE, TRUE, TRUE, FALSE, FALSE, FALSE, FALSE, FALSE, FALSE, FALSE, TRUE, FALSE, FALSE, TRUE, FALSE, FALSE, FALSE, FALSE, FALSE, FALSE, FALSE, FALSE, TRUE, FALSE, TRUE, TRUE, FALSE, FALSE, FALSE, FALSE, TRUE, FALSE, TRUE, TRUE, FALSE, FALSE, FALSE, FALSE, TRUE, FALSE, TRUE, TRUE, FALSE, FALSE, FALSE, FALSE, TRUE, FALSE, TRUE, TRUE, FALSE, FALSE, FALSE, FALSE, TRUE, FALSE, TRUE, TRUE, FALSE, FALSE, FALSE, FALSE, TRUE, FALSE, TRUE, TRUE, FALSE, FALSE, FALSE, FALSE, TRUE, FALSE, TRUE, TRUE, FALSE, FALSE, FALSE, FALSE, TRUE, FALSE, TRUE, TRUE, FALSE, FALSE, FALSE, FALSE, TRUE, FALSE, TRUE, TRUE, FALSE, FALSE, FALSE, FALSE, TRUE, FALSE, TRUE, TRUE, FALSE, FALSE, FALSE, FALSE, TRUE, FALSE, TRUE, TRUE, FALSE, FALSE, FALSE, FALSE, TRUE, FALSE, TRUE, TRUE, FALSE, FALSE, FALSE, FALSE, TRUE, FALSE, TRUE, TRUE, FALSE, FALSE, FALSE, FALSE, TRUE, FALSE, TRUE, TRUE, FALSE, FALSE, FALSE, FALSE, TRUE, FALSE, TRUE, TRUE, FALSE, FALSE, FALSE, FALSE, TRUE, FALSE, TRUE, TRUE, TRUE, FALSE, FALSE, FALSE, FALSE, FALSE, FALSE, FALSE, TRUE, FALSE, FALSE, TRUE, FALSE, FALSE, FALSE, FALSE, FALSE, FALSE, FALSE, FALSE, TRUE, FALSE, TRUE, TRUE, FALSE, FALSE, FALSE, FALSE, TRUE, FALSE, TRUE, TRUE, FALSE, FALSE, FALSE, FALSE, TRUE, FALSE, TRUE, TRUE, FALSE, FALSE, FALSE, FALSE, TRUE, FALSE, TRUE, TRUE, FALSE, FALSE, FALSE, FALSE, TRUE, FALSE, TRUE, TRUE, FALSE, FALSE, FALSE, FALSE, TRUE, FALSE, TRUE, TRUE, FALSE, FALSE, FALSE, FALSE, TRUE, FALSE, TRUE, TRUE, FALSE, FALSE, FALSE, FALSE, TRUE, FALSE, TRUE, TRUE, FALSE, FALSE, FALSE, FALSE, TRUE, FALSE, TRUE, TRUE, FALSE, FALSE, FALSE, FALSE, TRUE, FALSE, TRUE, TRUE, FALSE, FALSE, FALSE, FALSE, TRUE, FALSE, TRUE, TRUE, FALSE, FALSE, FALSE, FALSE, TRUE, FALSE, TRUE, TRUE, FALSE, FALSE, FALSE, FALSE, TRUE, FALSE, TRUE, TRUE, FALSE, FALSE, FALSE, FALSE, TRUE, FALSE, TRUE, TRUE, FALSE, FALSE, FALSE, FALSE, TRUE, FALSE, TRUE, TRUE, FALSE, FALSE, FALSE, FALSE, TRUE, FALSE, TRUE, TRUE, TRUE, FALSE, FALSE, FALSE, FALSE, FALSE, FALSE, FALSE, TRUE, FALSE, FALSE, TRUE, FALSE, FALSE, FALSE, FALSE, FALSE, FALSE, FALSE, FALSE, TRUE, FALSE, TRUE, TRUE, FALSE, FALSE, FALSE, FALSE, TRUE, FALSE, TRUE, TRUE, FALSE, FALSE, FALSE, FALSE, TRUE, FALSE, TRUE, TRUE, FALSE, FALSE, FALSE, FALSE, TRUE, FALSE, TRUE, TRUE, FALSE, FALSE, FALSE, FALSE, TRUE, FALSE, TRUE, TRUE, FALSE, FALSE, FALSE, FALSE, TRUE, FALSE, TRUE, TRUE, FALSE, FALSE, FALSE, FALSE, TRUE, FALSE, TRUE, TRUE, FALSE, FALSE, FALSE, FALSE, TRUE, FALSE, TRUE, TRUE, FALSE, FALSE, FALSE, FALSE, TRUE, FALSE, TRUE, TRUE, FALSE, FALSE, FALSE, FALSE, TRUE, FALSE, TRUE, TRUE, FALSE, FALSE, FALSE, FALSE, TRUE, FALSE, TRUE, TRUE, FALSE, FALSE, FALSE, FALSE, TRUE, FALSE, TRUE, TRUE, FALSE, FALSE, FALSE, FALSE, TRUE, FALSE, TRUE, TRUE, FALSE, FALSE, FALSE, FALSE, TRUE, FALSE, TRUE, TRUE, FALSE, FALSE, FALSE, FALSE, TRUE, FALSE, TRUE, TRUE, FALSE, FALSE, FALSE, FALSE, TRUE, FALSE, TRUE, TRUE, TRUE, FALSE, FALSE, FALSE, FALSE, FALSE, FALSE, FALSE, TRUE, FALSE, FALSE, TRUE, FALSE, FALSE, FALSE, FALSE]
  in  "SLK":bool=TRUE
  in  "STB":u16(ring) items=["Monitor Analog"=0, "Monitor Temp"=1, "Monitor Bandgap"=3]
  in  "Array 3":T6(array[cluster])=[[{"sts"=TRUE, "snc"=TRUE, "SG"=2, "ST"=0, "SDC"=FALSE, "SDF"=FALSE}, {"sts"=TRUE, "snc"=TRUE, "SG"=2, "ST"=0, "SDC"=FALSE, "SDF"=FALSE}, {"sts"=TRUE, "snc"=TRUE, "SG"=2, "ST"=0, "SDC"=FALSE, "SDF"=FALSE}, {"sts"=TRUE, "snc"=TRUE, "SG"=2, "ST"=0, "SDC"=FALSE, "SDF"=FALSE}, {"sts"=TRUE, "snc"=TRUE, "SG"=2, "ST"=0, "SDC"=FALSE, "SDF"=FALSE}, {"sts"=TRUE, "snc"=TRUE, "SG"=2, "ST"=0, "SDC"=FALSE, "SDF"=FALSE}, {"sts"=TRUE, "snc"=TRUE, "SG"=2, "ST"=0, "SDC"=FALSE, "SDF"=FALSE}, {"sts"=TRUE, "snc"=TRUE, "SG"=2, "ST"=0, "SDC"=FALSE, "SDF"=FALSE}], [{"sts"=TRUE, "snc"=TRUE, "SG"=2, "ST"=0, "SDC"=FALSE, "SDF"=FALSE}, {"sts"=TRUE, "snc"=TRUE, "SG"=2, "ST"=0, "SDC"=FALSE, "SDF"=FALSE}, {"sts"=TRUE, "snc"=TRUE, "SG"=2, "ST"=0, "SDC"=FALSE, "SDF"=FALSE}, {"sts"=TRUE, "snc"=TRUE, "SG"=2, "ST"=0, "SDC"=FALSE, "SDF"=FALSE}, {"sts"=TRUE, "snc"=TRUE, "SG"=2, "ST"=0, "SDC"=FALSE, "SDF"=FALSE}, {"sts"=TRUE, "snc"=TRUE, "SG"=2, "ST"=0, "SDC"=FALSE, "SDF"=FALSE}, {"sts"=TRUE, "snc"=TRUE, "SG"=2, "ST"=0, "SDC"=FALSE, "SDF"=FALSE}, {"sts"=TRUE, "snc"=TRUE, "SG"=2, "ST"=0, "SDC"=FALSE, "SDF"=FALSE}], [{"sts"=TRUE, "snc"=TRUE, "SG"=2, "ST"=0, "SDC"=FALSE, "SDF"=FALSE}, {"sts"=TRUE, "snc"=TRUE, "SG"=2, "ST"=0, "SDC"=FALSE, "SDF"=FALSE}, {"sts"=TRUE, "snc"=TRUE, "SG"=2, "ST"=0, "SDC"=FALSE, "SDF"=FALSE}, {"sts"=TRUE, "snc"=TRUE, "SG"=2, "ST"=0, "SDC"=FALSE, "SDF"=FALSE}, {"sts"=TRUE, "snc"=TRUE, "SG"=2, "ST"=0, "SDC"=FALSE, "SDF"=FALSE}, {"sts"=TRUE, "snc"=TRUE, "SG"=2, "ST"=0, "SDC"=FALSE, "SDF"=FALSE}, {"sts"=TRUE, "snc"=TRUE, "SG"=2, "ST"=0, "SDC"=FALSE, "SDF"=FALSE}, {"sts"=TRUE, "snc"=TRUE, "SG"=2, "ST"=0, "SDC"=FALSE, "SDF"=FALSE}], [{"sts"=TRUE, "snc"=TRUE, "SG"=2, "ST"=0, "SDC"=FALSE, "SDF"=FALSE}, {"sts"=TRUE, "snc"=TRUE, "SG"=2, "ST"=0, "SDC"=FALSE, "SDF"=FALSE}, {"sts"=TRUE, "snc"=TRUE, "SG"=2, "ST"=0, "SDC"=FALSE, "SDF"=FALSE}, {"sts"=TRUE, "snc"=TRUE, "SG"=2, "ST"=0, "SDC"=FALSE, "SDF"=FALSE}, {"sts"=TRUE, "snc"=TRUE, "SG"=2, "ST"=0, "SDC"=FALSE, "SDF"=FALSE}, {"sts"=TRUE, "snc"=TRUE, "SG"=2, "ST"=0, "SDC"=FALSE, "SDF"=FALSE}, {"sts"=TRUE, "snc"=TRUE, "SG"=2, "ST"=0, "SDC"=FALSE, "SDF"=FALSE}, {"sts"=TRUE, "snc"=TRUE, "SG"=2, "ST"=0, "SDC"=FALSE, "SDF"=FALSE}], [{"sts"=TRUE, "snc"=TRUE, "SG"=2, "ST"=0, "SDC"=FALSE, "SDF"=FALSE}, {"sts"=TRUE, "snc"=TRUE, "SG"=2, "ST"=0, "SDC"=FALSE, "SDF"=FALSE}, {"sts"=TRUE, "snc"=TRUE, "SG"=2, "ST"=0, "SDC"=FALSE, "SDF"=FALSE}, {"sts"=TRUE, "snc"=TRUE, "SG"=2, "ST"=0, "SDC"=FALSE, "SDF"=FALSE}, {"sts"=TRUE, "snc"=TRUE, "SG"=2, "ST"=0, "SDC"=FALSE, "SDF"=FALSE}, {"sts"=TRUE, "snc"=TRUE, "SG"=2, "ST"=0, "SDC"=FALSE, "SDF"=FALSE}, {"sts"=TRUE, "snc"=TRUE, "SG"=2, "ST"=0, "SDC"=FALSE, "SDF"=FALSE}, {"sts"=TRUE, "snc"=TRUE, "SG"=2, "ST"=0, "SDC"=FALSE, "SDF"=FALSE}], [{"sts"=TRUE, "snc"=TRUE, "SG"=2, "ST"=0, "SDC"=FALSE, "SDF"=FALSE}, {"sts"=TRUE, "snc"=TRUE, "SG"=2, "ST"=0, "SDC"=FALSE, "SDF"=FALSE}, {"sts"=TRUE, "snc"=TRUE, "SG"=2, "ST"=0, "SDC"=FALSE, "SDF"=FALSE}, {"sts"=TRUE, "snc"=TRUE, "SG"=2, "ST"=0, "SDC"=FALSE, "SDF"=FALSE}, {"sts"=TRUE, "snc"=TRUE, "SG"=2, "ST"=0, "SDC"=FALSE, "SDF"=FALSE}, {"sts"=TRUE, "snc"=TRUE, "SG"=2, "ST"=0, "SDC"=FALSE, "SDF"=FALSE}, {"sts"=TRUE, "snc"=TRUE, "SG"=2, "ST"=0, "SDC"=FALSE, "SDF"=FALSE}, {"sts"=TRUE, "snc"=TRUE, "SG"=2, "ST"=0, "SDC"=FALSE, "SDF"=FALSE}], [{"sts"=TRUE, "snc"=TRUE, "SG"=2, "ST"=0, "SDC"=FALSE, "SDF"=FALSE}, {"sts"=TRUE, "snc"=TRUE, "SG"=2, "ST"=0, "SDC"=FALSE, "SDF"=FALSE}, {"sts"=TRUE, "snc"=TRUE, "SG"=2, "ST"=0, "SDC"=FALSE, "SDF"=FALSE}, {"sts"=TRUE, "snc"=TRUE, "SG"=2, "ST"=0, "SDC"=FALSE, "SDF"=FALSE}, {"sts"=TRUE, "snc"=TRUE, "SG"=2, "ST"=0, "SDC"=FALSE, "SDF"=FALSE}, {"sts"=TRUE, "snc"=TRUE, "SG"=2, "ST"=0, "SDC"=FALSE, "SDF"=FALSE}, {"sts"=TRUE, "snc"=TRUE, "SG"=2, "ST"=0, "SDC"=FALSE, "SDF"=FALSE}, {"sts"=TRUE, "snc"=TRUE, "SG"=2, "ST"=0, "SDC"=FALSE, "SDF"=FALSE}], [{"sts"=TRUE, "snc"=TRUE, "SG"=2, "ST"=0, "SDC"=FALSE, "SDF"=FALSE}, {"sts"=TRUE, "snc"=TRUE, "SG"=2, "ST"=0, "SDC"=FALSE, "SDF"=FALSE}, {"sts"=TRUE, "snc"=TRUE, "SG"=2, "ST"=0, "SDC"=FALSE, "SDF"=FALSE}, {"sts"=TRUE, "snc"=TRUE, "SG"=2, "ST"=0, "SDC"=FALSE, "SDF"=FALSE}, {"sts"=TRUE, "snc"=TRUE, "SG"=2, "ST"=0, "SDC"=FALSE, "SDF"=FALSE}, {"sts"=TRUE, "snc"=TRUE, "SG"=2, "ST"=0, "SDC"=FALSE, "SDF"=FALSE}, {"sts"=TRUE, "snc"=TRUE, "SG"=2, "ST"=0, "SDC"=FALSE, "SDF"=FALSE}, {"sts"=TRUE, "snc"=TRUE, "SG"=2, "ST"=0, "SDC"=FALSE, "SDF"=FALSE}], [{"sts"=TRUE, "snc"=TRUE, "SG"=2, "ST"=0, "SDC"=FALSE, "SDF"=FALSE}, {"sts"=TRUE, "snc"=TRUE, "SG"=2, "ST"=0, "SDC"=FALSE, "SDF"=FALSE}, {"sts"=TRUE, "snc"=TRUE, "SG"=2, "ST"=0, "SDC"=FALSE, "SDF"=FALSE}, {"sts"=TRUE, "snc"=TRUE, "SG"=2, "ST"=0, "SDC"=FALSE, "SDF"=FALSE}, {"sts"=TRUE, "snc"=TRUE, "SG"=2, "ST"=0, "SDC"=FALSE, "SDF"=FALSE}, {"sts"=TRUE, "snc"=TRUE, "SG"=2, "ST"=0, "SDC"=FALSE, "SDF"=FALSE}, {"sts"=TRUE, "snc"=TRUE, "SG"=2, "ST"=0, "SDC"=FALSE, "SDF"=FALSE}, {"sts"=TRUE, "snc"=TRUE, "SG"=2, "ST"=0, "SDC"=FALSE, "SDF"=FALSE}], [{"sts"=TRUE, "snc"=TRUE, "SG"=2, "ST"=0, "SDC"=FALSE, "SDF"=FALSE}, {"sts"=TRUE, "snc"=TRUE, "SG"=2, "ST"=0, "SDC"=FALSE, "SDF"=FALSE}, {"sts"=TRUE, "snc"=TRUE, "SG"=2, "ST"=0, "SDC"=FALSE, "SDF"=FALSE}, {"sts"=TRUE, "snc"=TRUE, "SG"=2, "ST"=0, "SDC"=FALSE, "SDF"=FALSE}, {"sts"=TRUE, "snc"=TRUE, "SG"=2, "ST"=0, "SDC"=FALSE, "SDF"=FALSE}, {"sts"=TRUE, "snc"=TRUE, "SG"=2, "ST"=0, "SDC"=FALSE, "SDF"=FALSE}, {"sts"=TRUE, "snc"=TRUE, "SG"=2, "ST"=0, "SDC"=FALSE, "SDF"=FALSE}, {"sts"=TRUE, "snc"=TRUE, "SG"=2, "ST"=0, "SDC"=FALSE, "SDF"=FALSE}], [{"sts"=TRUE, "snc"=TRUE, "SG"=2, "ST"=0, "SDC"=FALSE, "SDF"=FALSE}, {"sts"=TRUE, "snc"=TRUE, "SG"=2, "ST"=0, "SDC"=FALSE, "SDF"=FALSE}, {"sts"=TRUE, "snc"=TRUE, "SG"=2, "ST"=0, "SDC"=FALSE, "SDF"=FALSE}, {"sts"=TRUE, "snc"=TRUE, "SG"=2, "ST"=0, "SDC"=FALSE, "SDF"=FALSE}, {"sts"=TRUE, "snc"=TRUE, "SG"=2, "ST"=0, "SDC"=FALSE, "SDF"=FALSE}, {"sts"=TRUE, "snc"=TRUE, "SG"=2, "ST"=0, "SDC"=FALSE, "SDF"=FALSE}, {"sts"=TRUE, "snc"=TRUE, "SG"=2, "ST"=0, "SDC"=FALSE, "SDF"=FALSE}, {"sts"=TRUE, "snc"=TRUE, "SG"=2, "ST"=0, "SDC"=FALSE, "SDF"=FALSE}], [{"sts"=TRUE, "snc"=TRUE, "SG"=2, "ST"=0, "SDC"=FALSE, "SDF"=FALSE}, {"sts"=TRUE, "snc"=TRUE, "SG"=2, "ST"=0, "SDC"=FALSE, "SDF"=FALSE}, {"sts"=TRUE, "snc"=TRUE, "SG"=2, "ST"=0, "SDC"=FALSE, "SDF"=FALSE}, {"sts"=TRUE, "snc"=TRUE, "SG"=2, "ST"=0, "SDC"=FALSE, "SDF"=FALSE}, {"sts"=TRUE, "snc"=TRUE, "SG"=2, "ST"=0, "SDC"=FALSE, "SDF"=FALSE}, {"sts"=TRUE, "snc"=TRUE, "SG"=2, "ST"=0, "SDC"=FALSE, "SDF"=FALSE}, {"sts"=TRUE, "snc"=TRUE, "SG"=2, "ST"=0, "SDC"=FALSE, "SDF"=FALSE}, {"sts"=TRUE, "snc"=TRUE, "SG"=2, "ST"=0, "SDC"=FALSE, "SDF"=FALSE}], [{"sts"=TRUE, "snc"=TRUE, "SG"=2, "ST"=0, "SDC"=FALSE, "SDF"=FALSE}, {"sts"=TRUE, "snc"=TRUE, "SG"=2, "ST"=0, "SDC"=FALSE, "SDF"=FALSE}, {"sts"=TRUE, "snc"=TRUE, "SG"=2, "ST"=0, "SDC"=FALSE, "SDF"=FALSE}, {"sts"=TRUE, "snc"=TRUE, "SG"=2, "ST"=0, "SDC"=FALSE, "SDF"=FALSE}, {"sts"=TRUE, "snc"=TRUE, "SG"=2, "ST"=0, "SDC"=FALSE, "SDF"=FALSE}, {"sts"=TRUE, "snc"=TRUE, "SG"=2, "ST"=0, "SDC"=FALSE, "SDF"=FALSE}, {"sts"=TRUE, "snc"=TRUE, "SG"=2, "ST"=0, "SDC"=FALSE, "SDF"=FALSE}, {"sts"=TRUE, "snc"=TRUE, "SG"=2, "ST"=0, "SDC"=FALSE, "SDF"=FALSE}], [{"sts"=TRUE, "snc"=TRUE, "SG"=2, "ST"=0, "SDC"=FALSE, "SDF"=FALSE}, {"sts"=TRUE, "snc"=TRUE, "SG"=2, "ST"=0, "SDC"=FALSE, "SDF"=FALSE}, {"sts"=TRUE, "snc"=TRUE, "SG"=2, "ST"=0, "SDC"=FALSE, "SDF"=FALSE}, {"sts"=TRUE, "snc"=TRUE, "SG"=2, "ST"=0, "SDC"=FALSE, "SDF"=FALSE}, {"sts"=TRUE, "snc"=TRUE, "SG"=2, "ST"=0, "SDC"=FALSE, "SDF"=FALSE}, {"sts"=TRUE, "snc"=TRUE, "SG"=2, "ST"=0, "SDC"=FALSE, "SDF"=FALSE}, {"sts"=TRUE, "snc"=TRUE, "SG"=2, "ST"=0, "SDC"=FALSE, "SDF"=FALSE}, {"sts"=TRUE, "snc"=TRUE, "SG"=2, "ST"=0, "SDC"=FALSE, "SDF"=FALSE}], [{"sts"=TRUE, "snc"=TRUE, "SG"=2, "ST"=0, "SDC"=FALSE, "SDF"=FALSE}, {"sts"=TRUE, "snc"=TRUE, "SG"=2, "ST"=0, "SDC"=FALSE, "SDF"=FALSE}, {"sts"=TRUE, "snc"=TRUE, "SG"=2, "ST"=0, "SDC"=FALSE, "SDF"=FALSE}, {"sts"=TRUE, "snc"=TRUE, "SG"=2, "ST"=0, "SDC"=FALSE, "SDF"=FALSE}, {"sts"=TRUE, "snc"=TRUE, "SG"=2, "ST"=0, "SDC"=FALSE, "SDF"=FALSE}, {"sts"=TRUE, "snc"=TRUE, "SG"=2, "ST"=0, "SDC"=FALSE, "SDF"=FALSE}, {"sts"=TRUE, "snc"=TRUE, "SG"=2, "ST"=0, "SDC"=FALSE, "SDF"=FALSE}, {"sts"=TRUE, "snc"=TRUE, "SG"=2, "ST"=0, "SDC"=FALSE, "SDF"=FALSE}], [{"sts"=TRUE, "snc"=TRUE, "SG"=2, "ST"=0, "SDC"=FALSE, "SDF"=FALSE}, {"sts"=TRUE, "snc"=TRUE, "SG"=2, "ST"=0, "SDC"=FALSE, "SDF"=FALSE}, {"sts"=TRUE, "snc"=TRUE, "SG"=2, "ST"=0, "SDC"=FALSE, "SDF"=FALSE}, {"sts"=TRUE, "snc"=TRUE, "SG"=2, "ST"=0, "SDC"=FALSE, "SDF"=FALSE}, {"sts"=TRUE, "snc"=TRUE, "SG"=2, "ST"=0, "SDC"=FALSE, "SDF"=FALSE}, {"sts"=TRUE, "snc"=TRUE, "SG"=2, "ST"=0, "SDC"=FALSE, "SDF"=FALSE}, {"sts"=TRUE, "snc"=TRUE, "SG"=2, "ST"=0, "SDC"=FALSE, "SDF"=FALSE}, {"sts"=TRUE, "snc"=TRUE, "SG"=2, "ST"=0, "SDC"=FALSE, "SDF"=FALSE}]] {"ST" items=["1us", "0.5us", "3us", "2us"]; "SG" items=["4.7 mV/fC", "7.8 mV/fC", "14 mV/fC", "25 mV/fC"]}
  out "size(s)":i32=1152
  out "size(s) 2":i32=1152
  out "ADC SPI OK":bool
  out "FE SPI OK":bool
  out "ADC FIFO SYNC":u16=65535 format="%016b"
  out "DAC  0x00-0x3f":u16=16 format="%x"
  in  "SLK 2":bool
  in  "DAC QUICK SET":bool
  in  "Global0":T7={"CLKG"=2, "FRQC"=0, "EN_GR"=0, "F0"=1, "F1"=0, "F2"=0, "F3"=0} {"F3" items=["0: IDL falling edge is delayed of 5-10ns after IDXM rising edge", "1: delay of 1 clock cycle on LVDS pin CLK"]; "F2" items=["0: the signal  generator on", "1: the signal  generator off"]; "F1" items=["0: a rising edge on LVDS pin ADC_CONV starts the sampling and readout", "1:the readout is compatible to V* version"]; "F0" items=["0: the ADC write clock is generated internally", "1: the ADC write clock is on LVDS pin IDXM"]; "FRQC" items=["0: 1 MHz", "1: 2 MHz "]; "CLKG" items=["0: ADC clocks from internal FIFO controller", "1: External clocks", "2: ADC clocks from internal monostable", "3: ADC clocks from internal FIFO controller"]; "EN_GR" items=["0: Disables offset current absorption", "1: Enables the offset current absorption"]}
  in  "Global1":T8={"F4"=1, "F5"=0, "sLSB"=0, "RES4-0(binary)"=0} {"RES4-0(binary)" items=["0", "1", "2", "3", "4", "5", "6", "7", "8", "9", "10", "11", "12", "13", "14", "15"]; "sLSB" items=["0: Full", "1: partial"]; "F5" items=["0: ADC data is selected and pipelined", "1: test data is selected and pipelined"]; "F4" items=["0: eanble F5", "1: CMOS pins CS and CLK controls the pipeline"]}
  in  "Sync_cnt":bool=TRUE
  in  "Cluster":T9={"EXT_RST"=TRUE, "EXT_READ"=TRUE, "EXT_MSB"=TRUE, "EXT_LSB"=TRUE, "EXT_LSBc"=TRUE, "ADC_CLK_200M"=TRUE, "ADC_CONV"=TRUE, "ADC_SPI_CS"=TRUE, "ADC_PD"=TRUE, "ADC_SPI_SCK"=TRUE, "ADC_SPI_SDO"=TRUE}
  in  "UDP READ":bool
  in  "UDP WRITE":bool
  out "DATA 3":u32=571627079 format="%x"
  in  "ADDRESS 3":u16=7 format="%x"
  in  "DATA":u32=571627079 format="%x"
  in  "ADDRESS":u16=7 format="%x"
  in  "Remote Host":string="192.168.121.1"
  out "start_udp_IO":string="OK"
  out "UDP_CLEANUP":string="ok"
  in  "ADDRESS 4":u16=16 format="%x"
  out "DATA 4":u32=267 format="%x"
  in  "DATA 2":u32=288 format="%x"
  in  "ADDRESS 2":u16=16 format="%x"
  in  "SBND I2C WRITE":bool
  in  "SBND I2C READ":bool
  in  "UDP/I2C":bool=TRUE
  in  "LBNE READ BLK":bool
  in  "BLK ADDRESS":u16=8
  out "BLK RD DATA":u32[](array[numeric]) format="%x"
  out "LBNE_DLL_VERSION":u32=102
  in  "enable":bool
  in  "Tab Control 4":T10(tab)
  in  "program \nFLASH":bool
  in  "Numeric":i32
  out "Meter":dbl(knob) scale=0.0..100.0
  out "PAGE 3":i32=15217
  out "READ ARRAY 2":u32[](array[numeric])=[0, 0, 0, 0, 0, 0, 0, 0, 0, 0, 17, 0, 268501009, 268500992, 4352, 268500992, 0, 0, 0, 1114112, 0, 0, 0, 0, 0, 0, 0, 4097, 0, 0, 0, 0, 0, 0, 0, 0, 0, 0, 0, 0, 0, 0, 0, 0, 0, 0, 0, 0, 49346, 3752002095, 1846345728, 0, 2961253394, 1410483634, 2170847556, 2219156004, 304223960, 313009179, 1210598437, 1361318696, 1363678808, 608862849, 1652632961, 1108584484] format="%x"
  out "WRITE ARRAY":u32[](array[numeric])=[2236879429, 310464840, 374875202, 715203606, 3625093268, 2169131592, 626074644, 709969942, 411345938, 1247969573, 2705857704, 612701202, 1410476625, 1209419940, 1210753316, 304159560, 763447890, 1210336293, 2702344466, 2243199396, 306872897, 2994852882, 672421924, 2236879402, 1099452744, 457712194, 709960731, 1210941768, 2219135560, 622944897, 709969947, 1210599466, 1361318744, 311059585, 1163020321, 672573458, 2234810698, 2722638417, 605102474, 1686193490, 1210337890, 2167017881, 2166039579, 1209733701, 1376855178, 1686192513, 1168253974, 2819757512, 2166039579, 1209209428, 323334785, 1686193284, 1168253970, 571922450, 2820938568, 675554641, 605235281, 1209423908, 1250066786, 2167243074, 330842450, 1211453732, 428364104, 374875202] format="%x"
  out "x = y?":bool
  out "pages 2":dbl=15292.25390625
  in  "LOAD RPD":bool
  out "DATA 5":u32 format="%x"
  in  "READ STATUS":bool
  in  "erase flash":bool
  in  "START FROM":i32=15217
  in  "STOP WRITE":bool
  out "DATA 6":u32 format="%x"
  out "NUM ATTEMP":i32=15217
  out "ONE_MORE":i32=15217
  out "x = y? 3":bool
  in  "verify\nFLASH":bool
  out "Meter 2":dbl(knob) scale=0.0..100.0
  out "PAGE 2":i32=15217
  out "READ ARRAY 3":u32[](array[numeric])=[0, 0, 0, 0, 0, 0, 0, 0, 0, 0, 17, 0, 268501009, 268500992, 4352, 268500992, 0, 0, 0, 1114112, 0, 0, 0, 0, 0, 0, 0, 4097, 0, 0, 0, 0, 0, 0, 0, 0, 0, 0, 0, 0, 0, 0, 0, 0, 0, 0, 0, 0, 49346, 3752002095, 1846345728, 0, 2961253394, 1410483634, 2170847556, 2219156004, 304223960, 313009179, 1210598437, 1361318696, 1363678808, 608862849, 1652632961, 1108584484] format="%x"
  out "WRITE ARRAY 2":u32[](array[numeric])=[2236879429, 310464840, 374875202, 715203606, 3625093268, 2169131592, 626074644, 709969942, 411345938, 1247969573, 2705857704, 612701202, 1410476625, 1209419940, 1210753316, 304159560, 763447890, 1210336293, 2702344466, 2243199396, 306872897, 2994852882, 672421924, 2236879402, 1099452744, 457712194, 709960731, 1210941768, 2219135560, 622944897, 709969947, 1210599466, 1361318744, 311059585, 1163020321, 672573458, 2234810698, 2722638417, 605102474, 1686193490, 1210337890, 2167017881, 2166039579, 1209733701, 1376855178, 1686192513, 1168253974, 2819757512, 2166039579, 1209209428, 323334785, 1686193284, 1168253970, 571922450, 2820938568, 675554641, 605235281, 1209423908, 1250066786, 2167243074, 330842450, 1211453732, 428364104, 374875202] format="%x"
  out "x = y? 2":bool
  in  "STOP VERIFY":bool
  in  "blank check":bool
  in  "start from":i32=15217
  in  "read flash":bool
  in  "P OFFSET":i32=15210
  in  "PAGES":i32=10
  out "PAGE":i32=104
  out "READ FROM FLASH":u32[][](array[numeric]) format="%x"
  out "FROM FILE":u32[][](array[numeric]) format="%x"
  in  "SAVE FLASH DATA":bool
  out "error out 2":errorcluster
  # "SW1   SW0   DAC5  DAC4  DAC3 DAC2 DAC1 DAC0"
  # "RAW BIN FILE"
  # "1"
  # "1"
  # "2"
  # "2"
  # "3"
  # "3"
  # "4"
  # "4"
  # "5"
  # "5"
  # "6"
  # "6"
  # "7"
  # "7"
  # "8"
  # "8"
  # "STATUS"
  # "0"
  # "1"
  # "2"
  # "3"
  # "4"
  # "5"
  # "6"
  # "7"
  # "8"
  # "9"
  # "10"
  # "11"
  # "12"
  # "13"
  # "14"
  # "15"
  # "STEP 1"
  # "STEP 2"
  # "STEP 3"
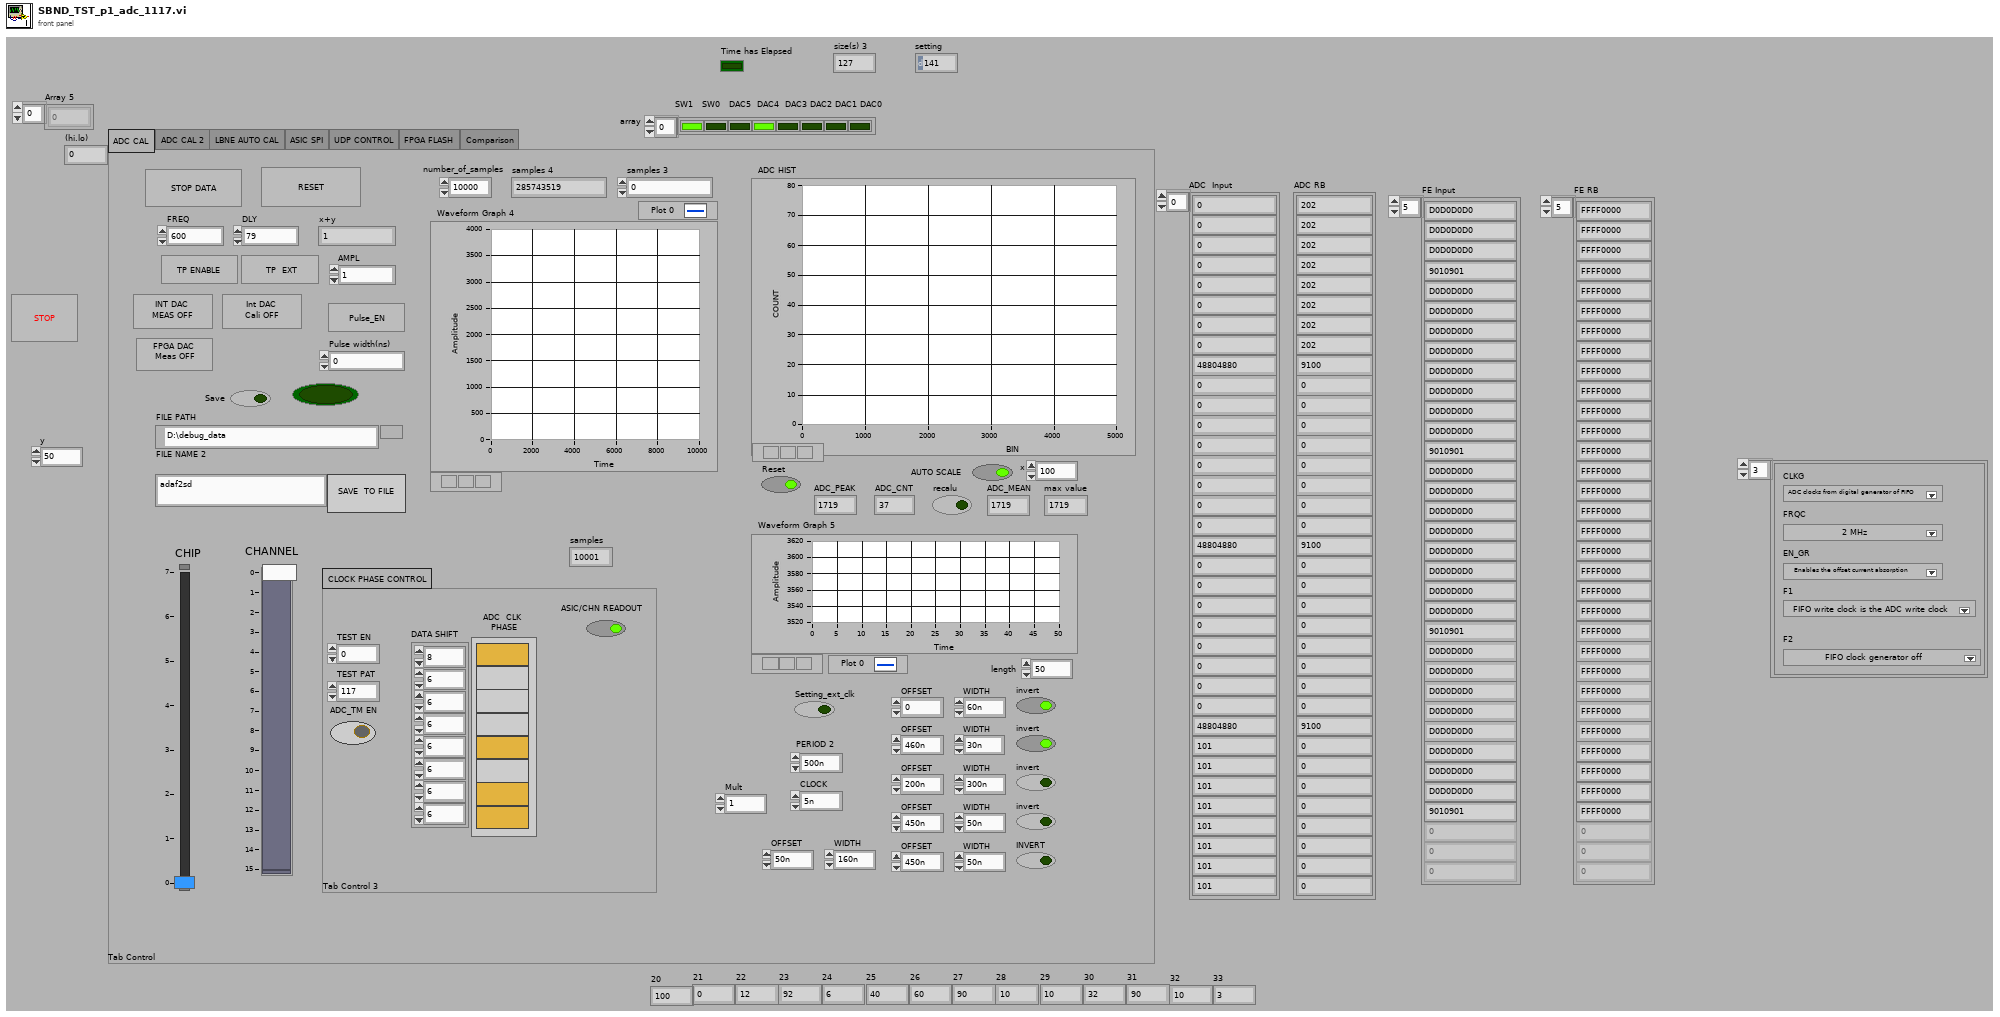
[diagram p1: front panel]
types:
  T1 = cluster{"EN_GR":u16, "CLKG":u16, "FRQC":u16, "F2":u16, "F1":u16}[]
  T2 = enum32{"ADC CAL", "ADC CAL 2", "LBNE AUTO CAL", "ASIC SPI", "UDP CONTROL", "FPGA FLASH", "Comparison"}
  T3 = cluster{"sts":bool, "snc":bool, "SG":u16, "ST":u16, "SDC":bool, "SDF":bool}
  T4 = cluster{"D_offset":u16, "PDSR":bool, "PCSR":bool, "slp":bool, "tst":bool}
  T5 = cluster{"D_offset":u16, "PDSR":bool, "PCSR":bool, "slp":bool, "tst":bool}[][]
  T6 = cluster{"sts":bool, "snc":bool, "SG":u16, "ST":u16, "SDC":bool, "SDF":bool}[][]
  T7 = cluster{"CLKG":u16, "FRQC":u16, "EN_GR":u16, "F0":u16, "F1":u16, "F2":u16, "F3":u16}
  T8 = cluster{"F4":u16, "F5":u16, "sLSB":u16, "RES4-0(binary)":u16}
  T9 = cluster{"EXT_RST":bool, "EXT_READ":bool, "EXT_MSB":bool, "EXT_LSB":bool, "EXT_LSBc":bool, "ADC_CLK_200M":bool, "ADC_CONV":bool, "ADC_SPI_CS":bool, "ADC_PD":bool, "ADC_SPI_SCK":bool, "ADC_SPI_SDO":bool}
  T10 = enum32{"PROGRAM FPGA", "VERIFY FPGA", "READ BACK AND SAVE"}
  T11 = cluster{"averaging mode":u16, "weighting mode":u16, "number of averages":u32}
  T12 = cluster{"dB On (F)":bool, "unwrap phase (F)":bool, "convert to degree (F)":bool}
  T13 = enum16{"open", "replace", "create", "open or create", "replace or create", "replace or create with confirmation"}
  T14 = enum16{"deny read/write", "deny write-only", "deny none"}
  T15 = cluster{"D_offset":u16, "PDSR":bool, "PCSR":bool, "slp":bool, "tst":bool}[]
  T16 = cluster{"sts":bool, "snc":bool, "SG":u16, "ST":u16, "SDC":bool, "SDF":bool}[]
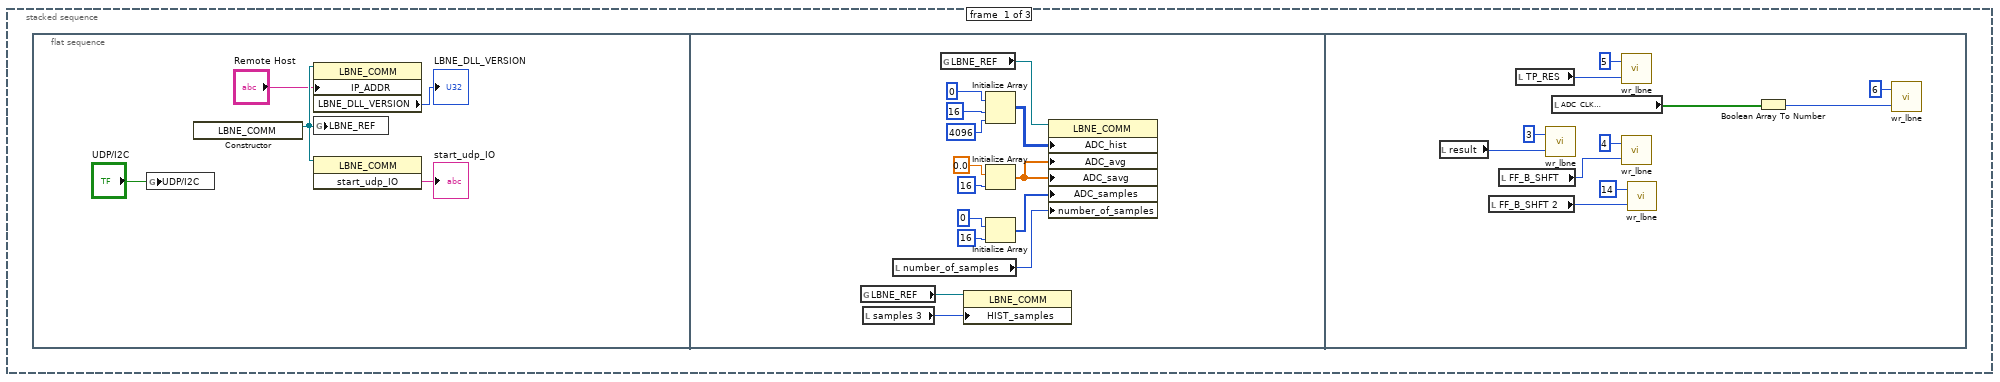
[diagram p2: hidden frame]
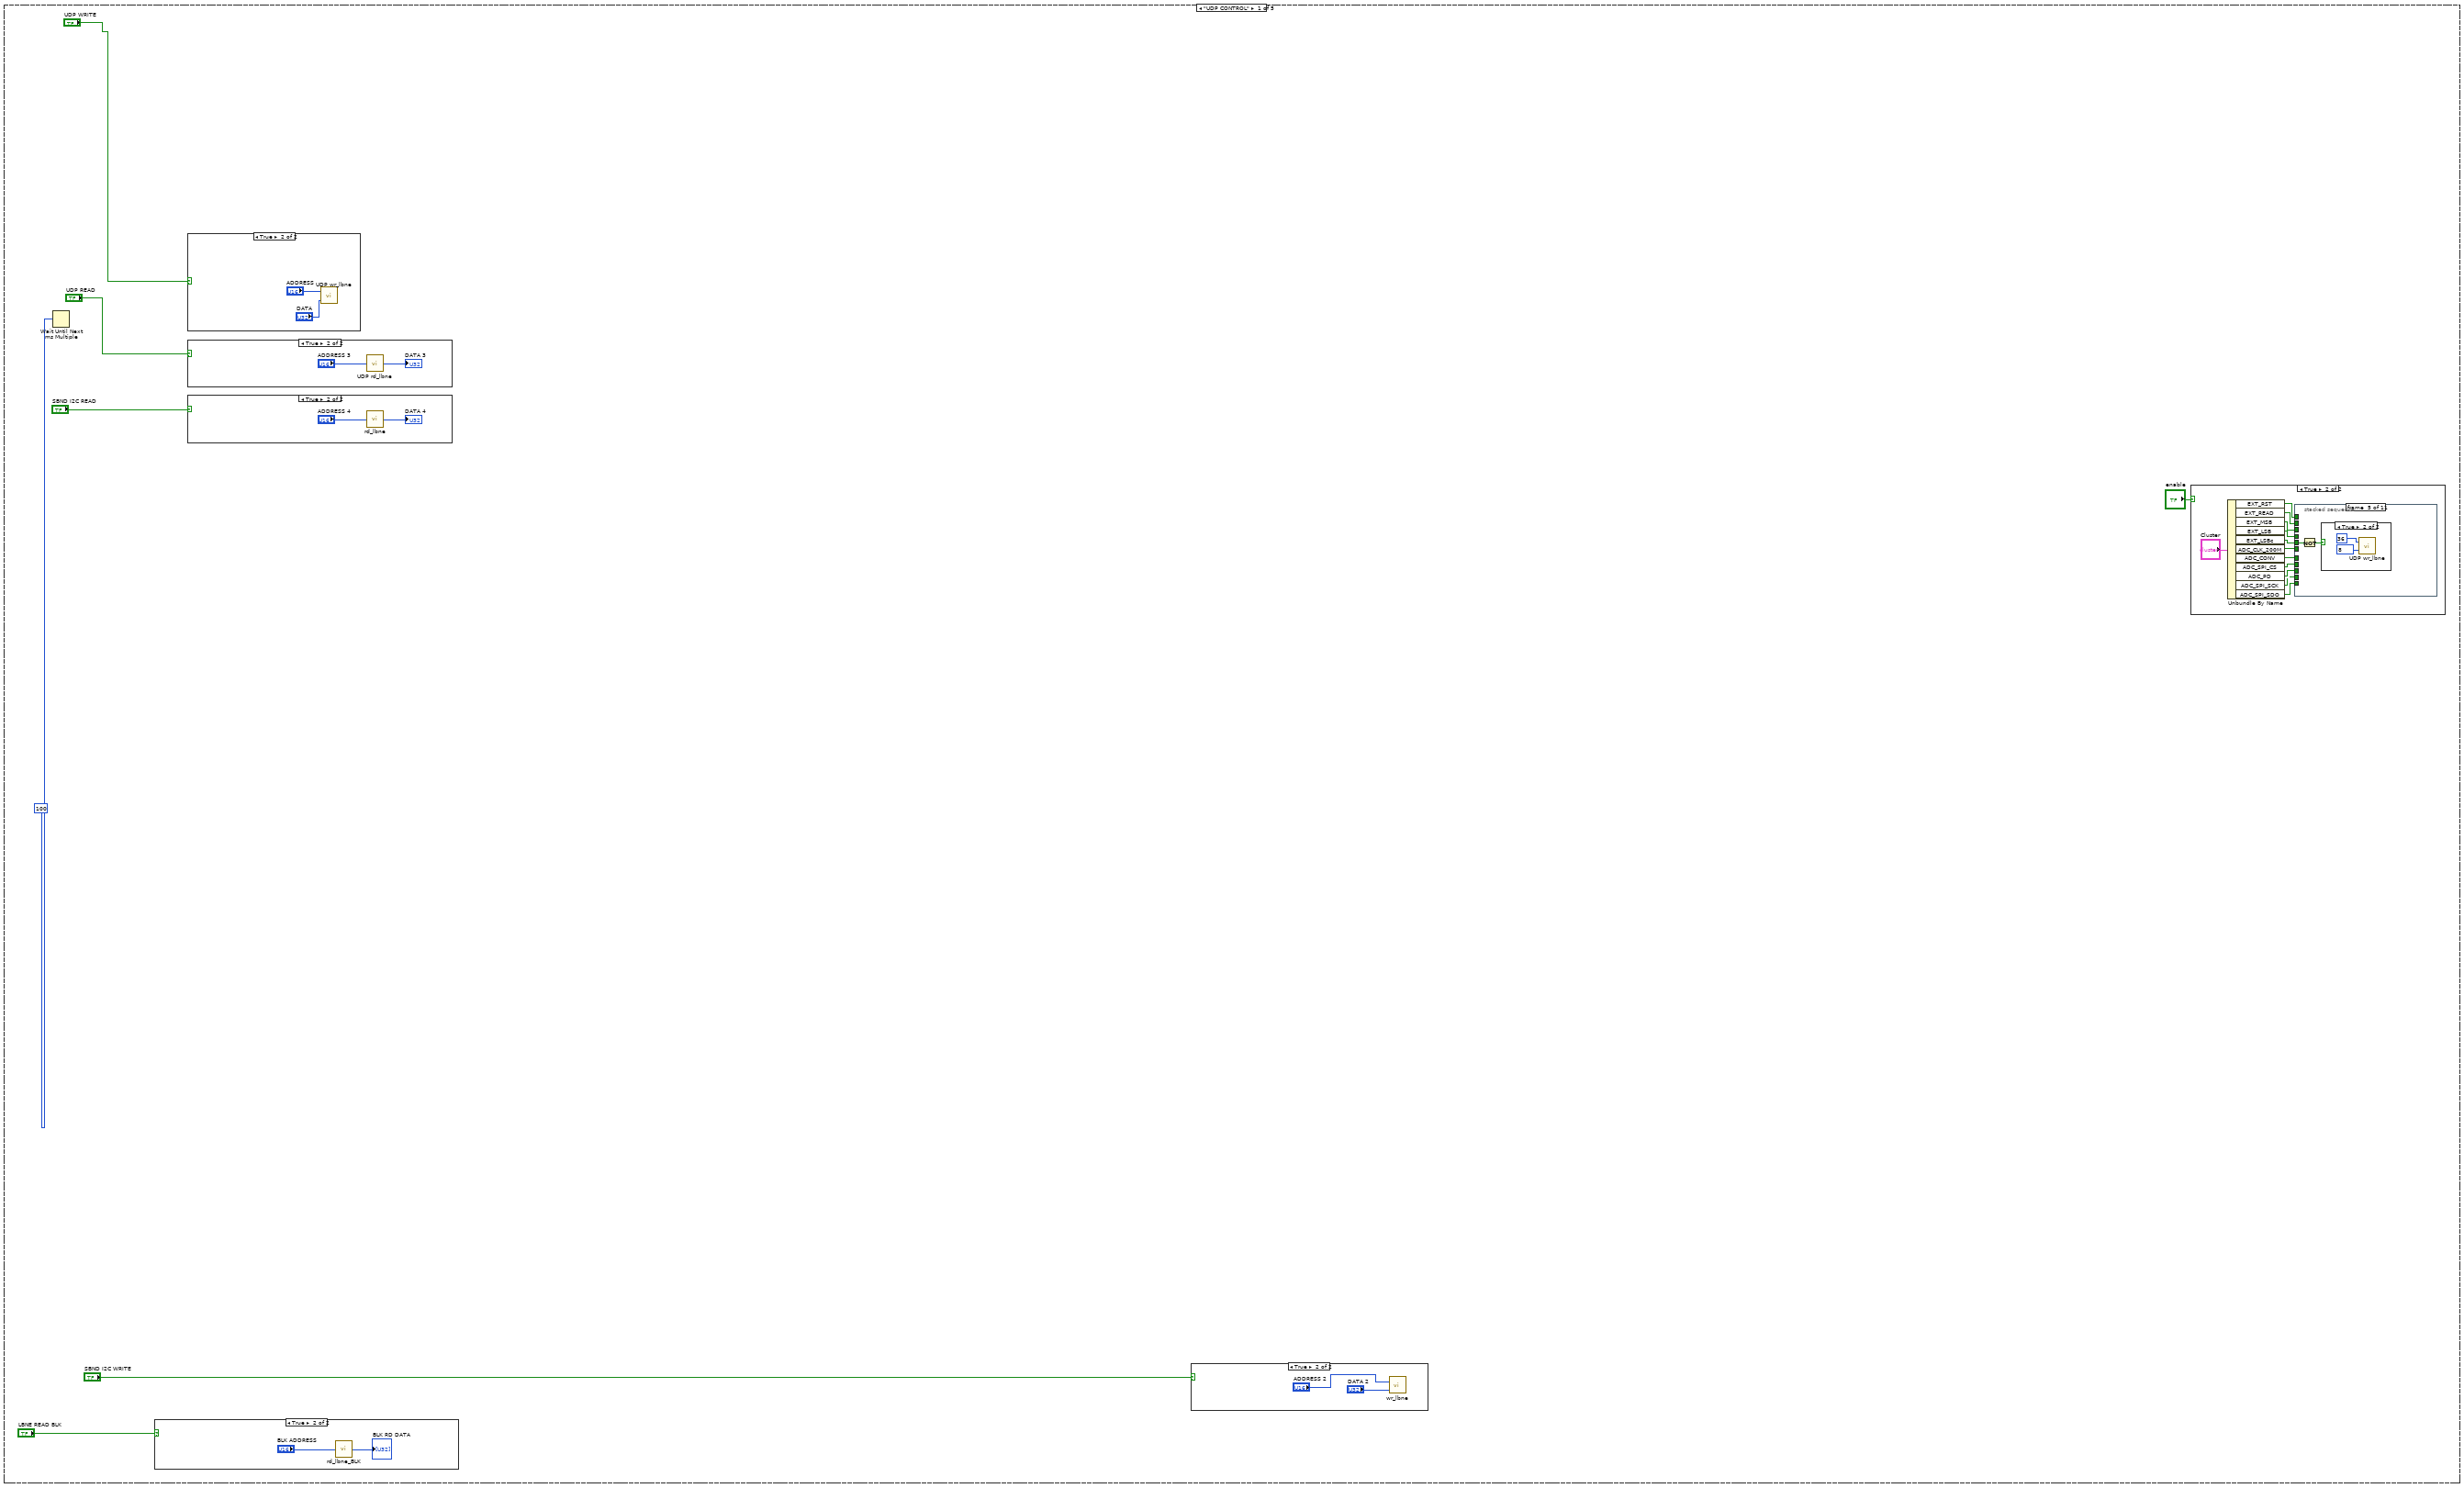
[diagram p3: hidden frame]
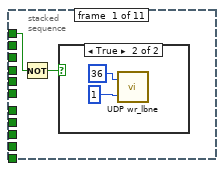
[diagram p5: hidden frame]
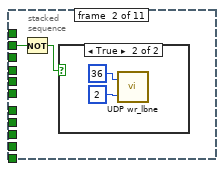
[diagram p7: hidden frame]
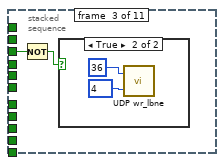
[diagram p9: hidden frame]
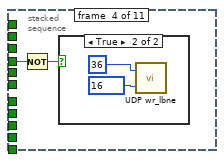
[diagram p11: hidden frame]
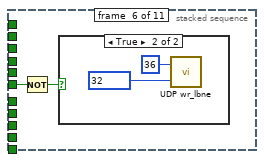
[diagram p14: hidden frame]
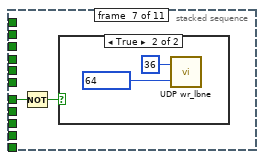
[diagram p16: hidden frame]
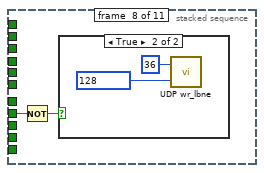
[diagram p18: hidden frame]
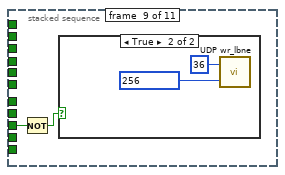
[diagram p20: hidden frame]
diagram:
  n1 = stacked-sequence {
    frame #0 {
      n2 = flat-sequence {
        frame #0 {
          n3 = global write "LBNE_Global .vi" "UDP/I2C"("UDP/I2C") -> ()
          n4 = constructor class="LBNE_COMM"() -> (reference out=w5:refnum<k24>)  [unwired: 3 in, 2 out]
          n5 = property class="LBNE_COMM"(reference=w5, "IP_ADDR"="Remote Host") -> ("LBNE_DLL_VERSION"=→"LBNE_DLL_VERSION":u32)  [unwired: 1 in, 2 out]
          n6 = global write "LBNE_Global .vi" "LBNE_REF"(w5) -> ()
          n7 = invoke class="LBNE_COMM" method="start_udp_IO"(reference=w5) -> ("start_udp_IO"=→"start_udp_IO":string)  [unwired: 2 in, 2 out]
        }
        frame #1 {
          n8 = global read "LBNE_Global .vi" "LBNE_REF"() -> (w18:refnum<k24>)
          n9 = local read "samples 3"() -> (w19:i32)
          n10 = local read "number_of_samples"() -> (w17:u32)
          n11 = global read "LBNE_Global .vi" "LBNE_REF"() -> (w6:refnum<k24>)
          n12 = property class="LBNE_COMM"(reference=w18, "HIST_samples"=w19) -> ()  [unwired: 1 in, 2 out]
          n13 = Initialize Array(u32 0 ("element"), 16 ("dimension size"), 4096 ("dimension size")) -> (w10:u32[][])
          n14 = Initialize Array(0.0 ("element"), 16 ("dimension size")) -> (w13:dbl[])
          n15 = Initialize Array(u32 0 ("element"), 16 ("dimension size")) -> (w15:u32[])
          n16 = property class="LBNE_COMM"(reference=w6, "ADC_hist"=w10, "ADC_avg"=w13, "ADC_savg"=w13, "ADC_samples"=w15, "number_of_samples"=w17) -> ()  [unwired: 1 in, 2 out]
        }
        frame #2 {
          n17 = local read "result"() -> (w27:u32)
          n18 = local read "FF_B_SHFT 2"() -> (w21:u32)
          n19 = local read "FF_B_SHFT"() -> (w30:u32)
          n20 = local read "TP_RES"() -> (w22:u32)
          n21 = call "wr_lbne.vi"("DATA"=w27, "ADDRESS"=u16 3) -> ()  [unwired: 1 out]
          n22 = local read "ADC  CLK \nPHASE"() -> (w24:bool[])
          n23 = call "wr_lbne.vi"("DATA"=w22, "ADDRESS"=u16 5) -> ()  [unwired: 1 out]
          n24 = call "wr_lbne.vi"("DATA"=w30, "ADDRESS"=u16 4) -> ()  [unwired: 1 out]
          n25 = call "wr_lbne.vi"("DATA"=w21, "ADDRESS"=u16 14) -> ()  [unwired: 1 out]
          n26 = Boolean Array To Number(Boolean array=w24) -> (number=w26:u32)
          n27 = call "wr_lbne.vi"("DATA"=w26, "ADDRESS"=u16 6 ("address")) -> ()  [unwired: 1 out]
        }
      }
    }
    frame #1 {
      n28 = while {
        shift-right: [w32] -> _
        shift-left: u32[] [] ("appended array") -> [w33]
        stop <- "stop" stop-if-true
        n29 = case shown="\"ASIC SPI\"" "Tab Control" {
          tunnel: w33 -> [_ w110 _ _ _]
          tunnel: [_ w109 _ _ _] -> w32
          frame "UDP CONTROL" {
            n30 = Wait Until Next ms Multiple(millisecond multiple=u32 100) -> ()  [unwired: 1 out]
            n31 = case shown="True" "LBNE READ BLK" {
              frame False {
              }
              frame True {
                n32 = call "rd_lbne_BLK.vi"("ADDRESS 2"="BLK ADDRESS") -> ("Array"=→"BLK RD DATA":u32[])
              }
            }
            n33 = case shown="True" "UDP WRITE" {
              frame False {
              }
              frame True {
                n34 = call "UDP wr_lbne.vi"("DATA"="DATA", "ADDRESS"="ADDRESS") -> ()  [unwired: 1 out]
              }
            }
            n35 = case shown="True" "UDP READ" {
              frame False {
              }
              frame True {
                n36 = call "UDP rd_lbne.vi"("ADDRESS 2"="ADDRESS 3") -> ("DATA 2"=→"DATA 3":u32)
              }
            }
            n37 = case shown="True" "SBND I2C READ" {
              frame False {
              }
              frame True {
                n38 = call "rd_lbne.vi"("ADDRESS 2"="ADDRESS 4") -> ("DATA 2"=→"DATA 4":u32)
              }
            }
            n39 = case shown="True" "SBND I2C WRITE" {
              frame False {
              }
              frame True {
                n40 = call "wr_lbne.vi"("DATA"="DATA 2", "ADDRESS"="ADDRESS 2") -> ()  [unwired: 1 out]
              }
            }
            n41 = case shown="True" "enable" {
              frame False {
              }
              frame True {
                n42 = Unbundle By Name("Cluster") -> ("EXT_RST"=w53:bool, "EXT_READ"=w52:bool, "EXT_MSB"=w51:bool, "EXT_LSB"=w50:bool, "EXT_LSBc"=w49:bool, "ADC_CLK_200M"=w48:bool, "ADC_CONV"=w47:bool, "ADC_SPI_CS"=w46:bool, "ADC_PD"=w45:bool, "ADC_SPI_SCK"=w44:bool, "ADC_SPI_SDO"=w43:bool)
                n43 = stacked-sequence {
                  tunnel: w53 -> [w56 _ _ _ _ _ _ _ _ _ _]
                  tunnel: w52 -> [_ w60 _ _ _ _ _ _ _ _ _]
                  tunnel: w51 -> [_ _ w63 _ _ _ _ _ _ _ _]
                  tunnel: w50 -> [_ _ _ w67 _ _ _ _ _ _ _]
                  tunnel: w49 -> [_ _ _ _ w71 _ _ _ _ _ _]
                  tunnel: w48 -> [_ _ _ _ _ w75 _ _ _ _ _]
                  tunnel: w47 -> [_ _ _ _ _ _ w79 _ _ _ _]
                  tunnel: w46 -> [_ _ _ _ _ _ _ w83 _ _ _]
                  tunnel: w45 -> [_ _ _ _ _ _ _ _ w87 _ _]
                  tunnel: w44 -> [_ _ _ _ _ _ _ _ _ w91 _]
                  tunnel: w43 -> [_ _ _ _ _ _ _ _ _ _ w95]
                  frame #0 {
                    n44 = Not(x=w56) -> (.not. x?=w55:bool)
                    n45 = case shown="True" w55 {
                      frame False {
                      }
                      frame True {
                        n46 = call "UDP wr_lbne.vi"("DATA"=u16 1 ("ADDRESS"), "ADDRESS"=u16 36) -> ()  [unwired: 1 out]
                      }
                    }
                  }
                  frame #1 {
                    n47 = Not(x=w60) -> (.not. x?=w59:bool)
                    n48 = case shown="True" w59 {
                      frame False {
                      }
                      frame True {
                        n49 = call "UDP wr_lbne.vi"("DATA"=u16 2 ("ADDRESS"), "ADDRESS"=u16 36) -> ()  [unwired: 1 out]
                      }
                    }
                  }
                  frame #2 {
                    n50 = Not(x=w63) -> (.not. x?=w64:bool)
                    n51 = case shown="True" w64 {
                      frame False {
                      }
                      frame True {
                        n52 = call "UDP wr_lbne.vi"("DATA"=u16 4 ("ADDRESS"), "ADDRESS"=u16 36) -> ()  [unwired: 1 out]
                      }
                    }
                  }
                  frame #3 {
                    n53 = Not(x=w67) -> (.not. x?=w68:bool)
                    n54 = case shown="True" w68 {
                      frame False {
                      }
                      frame True {
                        n55 = call "UDP wr_lbne.vi"("DATA"=u16 16 ("ADDRESS"), "ADDRESS"=u16 36) -> ()  [unwired: 1 out]
                      }
                    }
                  }
                  frame #4 {
                    n56 = Not(x=w71) -> (.not. x?=w72:bool)
                    n57 = case shown="True" w72 {
                      frame False {
                      }
                      frame True {
                        n58 = call "UDP wr_lbne.vi"("DATA"=u16 8 ("ADDRESS"), "ADDRESS"=u16 36) -> ()  [unwired: 1 out]
                      }
                    }
                  }
                  frame #5 {
                    n59 = Not(x=w75) -> (.not. x?=w76:bool)
                    n60 = case shown="True" w76 {
                      frame False {
                      }
                      frame True {
                        n61 = call "UDP wr_lbne.vi"("DATA"=u16 32 ("ADDRESS"), "ADDRESS"=u16 36) -> ()  [unwired: 1 out]
                      }
                    }
                  }
                  frame #6 {
                    n62 = Not(x=w79) -> (.not. x?=w80:bool)
                    n63 = case shown="True" w80 {
                      frame False {
                      }
                      frame True {
                        n64 = call "UDP wr_lbne.vi"("DATA"=u16 64 ("ADDRESS"), "ADDRESS"=u16 36) -> ()  [unwired: 1 out]
                      }
                    }
                  }
                  frame #7 {
                    n65 = Not(x=w83) -> (.not. x?=w84:bool)
                    n66 = case shown="True" w84 {
                      frame False {
                      }
                      frame True {
                        n67 = call "UDP wr_lbne.vi"("DATA"=u16 128 ("ADDRESS"), "ADDRESS"=u16 36) -> ()  [unwired: 1 out]
                      }
                    }
                  }
                  frame #8 {
                    n68 = Not(x=w87) -> (.not. x?=w88:bool)
                    n69 = case shown="True" w88 {
                      frame False {
                      }
                      frame True {
                        n70 = call "UDP wr_lbne.vi"("DATA"=u16 256 ("ADDRESS"), "ADDRESS"=u16 36) -> ()  [unwired: 1 out]
                      }
                    }
                  }
                  frame #9 {
                    n71 = Not(x=w91) -> (.not. x?=w92:bool)
                    n72 = case shown="True" w92 {
                      frame False {
                      }
                      frame True {
                        n73 = call "UDP wr_lbne.vi"("DATA"=u16 512 ("ADDRESS"), "ADDRESS"=u16 36) -> ()  [unwired: 1 out]
                      }
                    }
                  }
                  frame #10 {
                    n74 = Not(x=w95) -> (.not. x?=w96:bool)
                    n75 = case shown="True" w96 {
                      frame False {
                      }
                      frame True {
                        n76 = call "UDP wr_lbne.vi"("DATA"=u16 1024 ("ADDRESS"), "ADDRESS"=u16 36) -> ()  [unwired: 1 out]
                      }
                    }
                  }
                }
              }
            }
          }
          frame "ADC CAL", Default {
            n77 = Wait Until Next ms Multiple(millisecond multiple=u32 10) -> ()  [unwired: 1 out]
            n78 = global read "LBNE_Global .vi" "LBNE_REF"() -> (w113:refnum<k24>)
            n79 = property class="LBNE_COMM"(reference=w113) -> ("Store_Data"=→"Store_Data":bool)  [unwired: 1 in, 2 out]
            n80 = case shown="True" "RESET 6" {
              frame False {
              }
              frame True {
                n81 = flat-sequence {
                  tunnel: "number_of_samples" -> [w384]
                  frame #0 {
                    n82 = global read "LBNE_Global .vi" "LBNE_REF"() -> (w385:refnum<k24>)
                    n83 = global read "LBNE_Global .vi" "LBNE_REF"() -> (w387:refnum<k24>)
                    n84 = Initialize Array(u32 0 ("element"), 16 ("dimension size"), 4096 ("dimension size")) -> (w391:u32[][])
                    n85 = Initialize Array(0.0 ("element"), 16 ("dimension size")) -> (w394:dbl[])
                    n86 = Initialize Array(u32 0 ("element"), 16 ("dimension size")) -> (w396:u32[])
                    n87 = property class="LBNE_COMM"(reference=w387, "ADC_hist"=w391, "ADC_avg"=w394, "ADC_savg"=w394, "ADC_samples"=w396, "number_of_samples"=w384) -> ()  [unwired: 1 in, 2 out]
                    n88 = property class="LBNE_COMM"(reference=w385, "LV_READY"=FALSE) -> ()  [unwired: 1 in, 2 out]
                  }
                }
              }
            }
            n89 = event shown="[4] \"SYNC\", \"IntDAC_ON\", \"DAC_MEAS\", \"SYNC 3\", \"SYNC 2\", \"Pulse width(ns)\", \"pulse_en\": Value Change" {
              selector: _ -> [_ _ _ _ _ _ _ _]
              dyn-events: _ -> [_ _ _ _ _ _ _ _]
              timeout: 100 -> [_ _ _ _ _ _ _ _]
              event Timeout {
                n90 = event-data() -> ()  [unwired: 1 in, 2 out]
              }
              event "ADC_TM EN", "TEST PAT", "TEST EN", "ADC  CLK \nPHASE", "DATA SHIFT": Value Change {
                n91 = event-data() -> ()  [unwired: 1 in, 6 out]
                n92 = Boolean Array To Number(Boolean array="ADC  CLK \nPHASE") -> (number=w237:u32)
                n93 = Boolean To (0,1)(Boolean="ADC_TM EN") -> (0, 1=w242:i16)
                n94 = call "wr_lbne.vi"("DATA"=w237, "ADDRESS"=u16 6 ("address")) -> ()  [unwired: 1 out]
                n95 = for {
                  tunnel: "DATA SHIFT" -> [w259] mode=indexing
                  shift-right: [w254] -> _
                  shift-left: bool[] [] -> [w256]
                  tunnel: [w255] -> w233
                  tunnel: [w252] -> w231
                  w253 = 32 ("length")
                  n96 = Number To Boolean Array(number=w259) -> (Boolean array=w258:bool[])
                  n97 = Array Subset(array=w258, length=8) -> (w257:bool[])  [unwired: 1 in]
                  n98 = Build Array (concatenate)(w256, w257) -> (w254:bool[])
                  n99 = Array Subset(array=w254, index=w253, length=w253) -> (w252:bool[])
                  n100 = Array Subset(array=w254, length=w253) -> (w255:bool[])  [unwired: 1 in]
                }
                n101 = To Unsigned Long Integer(number=w242) -> (unsigned 32bit integer=w243:u32)
                n102 = Logical Shift(y=i16 16, x="TEST PAT") -> (x << y=w246:u32)
                n103 = Logical Shift(y=i16 31, x=w243) -> (x << y=w245:u32)
                n104 = Compound Arithmetic op=OR("TEST EN", w246, w245) -> (w240:u32)
                "result" <- w240
                n105 = call "wr_lbne.vi"("DATA"=w240, "ADDRESS"=u16 3 ("address")) -> ()  [unwired: 1 out]
                n106 = Boolean Array To Number(Boolean array=w231) -> (number=w230:u32)
                "FF_B_SHFT 2" <- w230
                n107 = Boolean Array To Number(Boolean array=w233) -> (number=w234:u32)
                "FF_B_SHFT" <- w234
                n108 = call "wr_lbne.vi"("DATA"=w234, "ADDRESS"=u16 4 ("address")) -> ()  [unwired: 1 out]
                n109 = call "wr_lbne.vi"("DATA"=w230, "ADDRESS"=u16 14 ("address")) -> ()  [unwired: 1 out]
              }
              event "STOP_DATA": Value Change {
                n110 = event-data() -> ()  [unwired: 1 in, 6 out]
                n111 = Select(t=2.0, s="STOP_DATA", f=0.0) -> (s? t:f=w264:dbl)
                n112 = call "wr_lbne.vi"("DATA"=w264, "ADDRESS"=u16 30 ("address")) -> ()  [unwired: 1 out]
              }
              event "FREQ", "DLY", "AMPL": Value Change {
                n113 = event-data() -> ()  [unwired: 1 in, 6 out]
                n114 = Quotient & Remainder(x="AMPL", y=u8 64) -> (x-y*floor(x/y)=w266:u8)  [unwired: 1 out]
                "x+y" <- w266
                n115 = Join Numbers(hi="DLY", lo=w266) -> ((hi.lo)=w271:u16)
                n116 = Join Numbers(hi="FREQ", lo=w271) -> ((hi.lo)=w269:u32)
                "TP_RES" <- w269
                n117 = call "wr_lbne.vi"("DATA"=w269, "ADDRESS"=u16 5) -> ()  [unwired: 1 out]
              }
              event "SYNC", "IntDAC_ON", "DAC_MEAS", "SYNC 3", "SYNC 2", "Pulse width(ns)", "pulse_en": Value Change {
                n118 = event-data() -> ()  [unwired: 1 in, 6 out]
                n119 = flat-sequence {
                  frame #0 {
                    n120 = Boolean To (0,1)(Boolean="SYNC") -> (0, 1=w289:i16)
                    n121 = Select(t=u8 10, s="IntDAC_ON", f=u8 0) -> (s? t:f=w282:u8)
                    n122 = Boolean To (0,1)(Boolean="SYNC 3") -> (0, 1=w288:i16)
                    n123 = To Unsigned Byte Integer(number=w289) -> (unsigned 8bit integer=w280:u8)
                    n124 = Select(t=u8 6, s="DAC_MEAS", f=w282) -> (s? t:f=w279:u8)
                    n125 = Or(x=w280, y=w279) -> (x .or. y?=w277:u8)
                    n126 = To Unsigned Byte Integer(number=w288) -> (unsigned 8bit integer=w287:u8)
                    n127 = Join Numbers(hi=w287, lo=w277) -> ((hi.lo)=w275:u16)
                    n128 = Select(t=u16 384, s="SYNC 2", f=w275) -> (s? t:f=w274:u16)
                    "(hi.lo)" <- w274
                    n129 = call "wr_lbne.vi"("DATA"=w274, "ADDRESS"=u16 16) -> ()  [unwired: 1 out]
                  }
                  frame #1 {
                    n130 = local read "TP_RES"() -> (w295:u32)
                    n131 = Or(x=w295, y=u32 1) -> (x .or. y?=w293:u32)
                    n132 = call "wr_lbne.vi"("DATA"=w293, "ADDRESS"=u16 5) -> ()  [unwired: 1 out]
                  }
                  frame #2 {
                    n133 = Divide(x="Pulse width(ns)", y=u16 20) -> (x/y=w304:dbl)
                    n134 = To Unsigned Word Integer(number=w304) -> (unsigned 16bit integer=w303:u16)
                    n135 = Decrement(x=w303) -> (x-1=w298:u16)
                    n136 = Select(t=u16 32768, s="pulse_en", f=u16 0 ("t")) -> (s? t:f=w299:u16)
                    n137 = Join Numbers(hi=w299, lo=w298) -> ((hi.lo)=w297:u32)
                    n138 = call "wr_lbne.vi"("DATA"=w297, "ADDRESS"=u16 20) -> ()  [unwired: 1 out]
                  }
                }
              }
              event "Setting_ext_clk": Value Change {
                n139 = event-data() -> ()  [unwired: 1 in, 6 out]
                n140 = case shown="True" "Setting_ext_clk" {
                  frame False {
                  }
                  frame True {
                    n141 = Divide(x="CLOCK", y="Mult") -> (x/y=w323:dbl)
                    n142 = Build Array("invert", "invert 2", "invert 3", "invert 4", "invert 5") -> (w340:bool[])
                    n143 = Boolean Array To Number(Boolean array=w340) -> (number=w341:u32)
                    n144 = Divide(x="LSB_S_WID", y=w323) -> (x/y=w370:dbl)
                    n145 = Divide(x="LSB_FC_OFF2", y=w323) -> (x/y=w361:dbl)
                    n146 = Divide(x="LSB_FC_WID1", y=w323) -> (x/y=w363:dbl)
                    n147 = Divide(x="RD/EN_WID", y=w323) -> (x/y=w367:dbl)
                    n148 = Divide(x="LSB_FC_OFF1", y=w323) -> (x/y=w362:dbl)
                    n149 = Divide(x="LSB_FC_WID2", y=w323) -> (x/y=w360:dbl)
                    n150 = Divide(x="PERIOD 2", y=w323) -> (x/y=w371:dbl)
                    n151 = Divide(x="MSB_WID", y=w323) -> (x/y=w368:dbl)
                    n152 = Divide(x="MSB_OFF", y=w323) -> (x/y=w372:dbl)
                    n153 = Divide(x="ADC_WID", y=w323) -> (x/y=w365:dbl)
                    n154 = Divide(x="ADC_OFF", y=w323) -> (x/y=w364:dbl)
                    n155 = Divide(x="LSB_S_OFF", y=w323) -> (x/y=w369:dbl)
                    n156 = Divide(x="RD/EN_OFF", y=w323) -> (x/y=w366:dbl)
                    n157 = To Unsigned Word Integer(number=w341) -> (unsigned 16bit integer=w309:u16)
                    "INV_REG" <- w309
                    "33" <- w309
                    n158 = To Unsigned Word Integer(number=w370) -> (unsigned 16bit integer=w315:u16)
                    "28" <- w315
                    n159 = To Unsigned Word Integer(number=w361) -> (unsigned 16bit integer=w312:u16)
                    "31" <- w312
                    n160 = To Unsigned Word Integer(number=w363) -> (unsigned 16bit integer=w313:u16)
                    "30" <- w313
                    n161 = To Unsigned Word Integer(number=w367) -> (unsigned 16bit integer=w319:u16)
                    "24" <- w319
                    n162 = To Unsigned Word Integer(number=w362) -> (unsigned 16bit integer=w314:u16)
                    "29" <- w314
                    n163 = To Unsigned Word Integer(number=w360) -> (unsigned 16bit integer=w311:u16)
                    "32" <- w311
                    n164 = To Unsigned Word Integer(number=w371) -> (unsigned 16bit integer=w334:u16)
                    "20" <- w334
                    n165 = To Unsigned Word Integer(number=w368) -> (unsigned 16bit integer=w317:u16)
                    "26" <- w317
                    n166 = To Unsigned Word Integer(number=w372) -> (unsigned 16bit integer=w318:u16)
                    "25" <- w318
                    n167 = To Unsigned Word Integer(number=w365) -> (unsigned 16bit integer=w321:u16)
                    "22" <- w321
                    n168 = To Unsigned Word Integer(number=w364) -> (unsigned 16bit integer=w322:u16)
                    "21" <- w322
                    n169 = To Unsigned Word Integer(number=w369) -> (unsigned 16bit integer=w316:u16)
                    "27" <- w316
                    n170 = To Unsigned Word Integer(number=w366) -> (unsigned 16bit integer=w320:u16)
                    "23" <- w320
                    n171 = call "wr_lbne.vi"("DATA"=w309, "ADDRESS"=u16 33 ("ADDRESS 2")) -> ()  [unwired: 1 out]
                    n172 = call "wr_lbne.vi"("DATA"=w315, "ADDRESS"=u16 28 ("ADDRESS 2")) -> ()  [unwired: 1 out]
                    n173 = call "wr_lbne.vi"("DATA"=w312, "ADDRESS"=u16 31 ("ADDRESS 2")) -> ()  [unwired: 1 out]
                    n174 = call "wr_lbne.vi"("DATA"=w313, "ADDRESS"=u16 30 ("ADDRESS 2")) -> ()  [unwired: 1 out]
                    n175 = call "wr_lbne.vi"("DATA"=w319, "ADDRESS"=u16 24 ("ADDRESS 2")) -> ()  [unwired: 1 out]
                    n176 = call "wr_lbne.vi"("DATA"=w314, "ADDRESS"=u16 29 ("ADDRESS 2")) -> ()  [unwired: 1 out]
                    n177 = call "wr_lbne.vi"("DATA"=w311, "ADDRESS"=u16 32 ("ADDRESS 2")) -> ()  [unwired: 1 out]
                    n178 = call "wr_lbne.vi"("DATA"=w334, "ADDRESS"=u16 20 ("ADDRESS 2")) -> ()  [unwired: 1 out]
                    n179 = call "wr_lbne.vi"("DATA"=w317, "ADDRESS"=u16 26 ("ADDRESS 2")) -> ()  [unwired: 1 out]
                    n180 = call "wr_lbne.vi"("DATA"=w318, "ADDRESS"=u16 25 ("ADDRESS 2")) -> ()  [unwired: 1 out]
                    n181 = call "wr_lbne.vi"("DATA"=w321, "ADDRESS"=u16 22 ("ADDRESS 2")) -> ()  [unwired: 1 out]
                    n182 = call "wr_lbne.vi"("DATA"=w322, "ADDRESS"=u16 21 ("ADDRESS 2")) -> ()  [unwired: 1 out]
                    n183 = call "wr_lbne.vi"("DATA"=w316, "ADDRESS"=u16 27 ("ADDRESS 2")) -> ()  [unwired: 1 out]
                    n184 = call "wr_lbne.vi"("DATA"=w320, "ADDRESS"=u16 23 ("ADDRESS 2")) -> ()  [unwired: 1 out]
                  }
                }
              }
              event "samples 3": Value Change {
                n185 = event-data() -> ()  [unwired: 1 in, 6 out]
                n186 = global read "LBNE_Global .vi" "LBNE_REF"() -> (w374:refnum<k24>)
                n187 = property class="LBNE_COMM"(reference=w374, "HIST_samples"="samples 3") -> ()  [unwired: 1 in, 2 out]
              }
              event "CHANNEL", "CHIP", "ASIC/CHN READOUT": Value Change {
                n188 = event-data() -> ()  [unwired: 1 in, 6 out]
                n189 = global read "LBNE_Global .vi" "LBNE_REF"() -> (w379:refnum<k24>)
                n190 = property class="LBNE_COMM"(reference=w379, "CHN_SEL"="CHANNEL") -> ()  [unwired: 1 in, 2 out]
                n191 = Join Numbers(hi="CHANNEL", lo="CHIP") -> ((hi.lo)=w381:u16)
                n192 = Boolean To (0,1)(Boolean="ASIC/CHN READOUT") -> (0, 1=w376:i16)
                n193 = call "wr_lbne.vi"("DATA"=w381, "ADDRESS"=u16 7 ("address")) -> ()  [unwired: 1 out]
                n194 = call "wr_lbne.vi"("DATA"=w376, "ADDRESS"=u16 17 ("address")) -> ()  [unwired: 1 out]
              }
            }
            n195 = stacked-sequence {
              tunnel: w110 -> [w118 _]
              tunnel: [w117 _] -> w109
              frame #0 {
                n196 = local read "STOP_DATA"() -> (w127:bool)
                n197 = global read "LBNE_Global .vi" "LBNE_REF"() -> (w122:refnum<k24>)
                n198 = property class="LBNE_COMM"(reference=w122) -> ("LV_READY"=w120:bool)  [unwired: 1 in, 2 out]
                n199 = Not(x=w127) -> (.not. x?=w121:bool)
                n200 = And(x=w121, y=w120) -> (x .and. y?=w119:bool)
                n201 = case shown="True" w119 {
                  tunnel: [w129 w132] -> w123
                  tunnel: w118 -> [w128 w131]
                  tunnel: [w128 w130] -> w117
                  frame False {
                    n202 = local read "ADC_hist"() -> (w129:u32[][])
                  }
                  frame True {
                    n203 = stacked-sequence {
                      tunnel: [w147 _] -> w132
                      tunnel: w131 -> [w144 _]
                      tunnel: [w145 _] -> w130
                      frame #0 {
                        n204 = global read "LBNE_Global .vi" "LBNE_REF"() -> (w159:refnum<k24>)
                        n205 = case shown="False" "recalu" {
                          tunnel: [w174 u32[] [] ("appended array")] -> w142
                          tunnel: w144 -> [w174 _]
                          frame False {
                          }
                          frame True {
                          }
                        }
                        n206 = case shown="False" "AUTO SCALE" {
                          frame False {
                          }
                          frame True {
                            n207 = local read "ADC_PEAK"() -> (w207:u32)
                            n208 = Add(x="x", y=w207) -> (x+y=w206:u32)
                            n209 = Subtract(x=w207, y="x") -> (x-y=w205:u32)
                            n210 = property on="ADC HIST" class="WFGraph (strict)"("XScale.Maximum"=w206, "XScale.Minimum"=w205) -> ()  [unwired: 2 in, 2 out]
                          }
                        }
                        n211 = property class="LBNE_COMM" props=["receive_word_array", "ADC_hist", "ADC_samples", "receive_byte_array"](reference=w159) -> ("receive_word_array"=w136:u32[], "ADC_hist"=w147:u32[][], "ADC_samples"=w155:u32[])  [unwired: 1 in, 3 out]
                        "Waveform Graph 4" <- w136
                        "ADC_hist" <- w147
                        n212 = local read "CHANNEL"() -> (w154:u8)
                        n213 = case shown="True" "Boolean" {
                          tunnel: w136 -> [_ w179]
                          frame False {
                          }
                          frame True {
                            n214 = Bundle By Name("Y"=w179, "dt"=5e-07) -> (w178:waveform(u32))  [unwired: 1 in]
                            n215 = xnode "Spectral Measurements"("Signals"=w178, "Restart Averaging"="Restart Averaging") -> ("Power Spectrum"=→"Waveform Graph":dynamicdata)  [unwired: 1 in, 2 out]
                          }
                        }
                        n216 = case shown="True" "Save" {
                          tunnel: w136 -> [_ w173]
                          frame False {
                          }
                          frame True {
                            n217 = call "Convert to Dynamic Data8"("Array"=w173) -> ("Dynamic Data Type"=w170:dynamicdata)  [unwired: 3 in]
                            n218 = local read "setting"() -> (w166:u16)
                            n219 = local read "FILE PATH 2"() -> (w167:path)
                            n220 = Number To Decimal String(number=w166, width (-)=i16 3) -> (decimal integer string=w168:string)
                            n221 = Build Path(base path=w167, name or relative path=w168) -> (appended path=w165:path)
                            n222 = Build Path(base path=w165, name or relative path="raw_data") -> (appended path=w171:path)
                            n223 = call "Write To Measurement File4"("Signals"=w170, "Filename"=w171) -> ()  [unwired: 15 in, 3 out]
                          }
                        }
                        n224 = Index Array(array=w155, index=w154) -> (element=→"samples 4":u32)
                        n225 = Array Size(array=w136) -> (size(s)=→"samples":i32)
                        n226 = Array Max & Min(array=w136) -> (max value=w160:u32)  [unwired: 3 out]
                        n227 = call "Convert to Dynamic Data"("Array"=w142) -> ("Dynamic Data Type"=w157:dynamicdata)  [unwired: 3 in]
                        n228 = call "Convert to Dynamic Data7"("Array"=w136) -> ("Dynamic Data Type"=w141:dynamicdata)  [unwired: 3 in]
                        n229 = call "Statistics4"("Signals"=w141) -> ("Standard Dev"=→"Peds_RMS":dynamicdata, "Arithmetic Mean"=→"Peds Mean":dynamicdata)  [unwired: 23 in, 2 out]
                        n230 = call "Statistics"("Signals"=w157) -> ("Total Samples"=→"ADC_CNT":dynamicdata, "Arithmetic Mean"=→"ADC_MEAN":dynamicdata)  [unwired: 23 in, 2 out]
                        n231 = Subtract(x=w160, y="y") -> (x-y=w161:u32)
                        n232 = call "Convert to Dynamic Data9"("Array"=w136) -> ("Dynamic Data Type"=w135:dynamicdata)  [unwired: 3 in]
                        n233 = call "Create Histogram"("Reset"="Reset", "Signal"=w135) -> ("Histogram"=→"ADC HIST":dynamicdata)  [unwired: 8 in, 1 out]
                        n234 = call <vilib>:"Peak Detector.vi"("peaks/valleys"=enum32{"Peaks", "Valleys"}."Peaks", "width"=3, "threshold"=w161, "X"=w136) -> ("Locations"=w152:dbl[], "# found"=w150:i32)  [unwired: 3 in, 3 out]
                        n235 = Greater Or Equal?(x=w150, y=3 ("x")) -> (x >= y?=w153:bool)
                        n236 = case shown="True" w153 {
                          tunnel: w152 -> [_ w203]
                          tunnel: w136 -> [_ w200]
                          tunnel: w142 -> [w191 w194]
                          tunnel: [w191 w193] -> w145
                          frame False {
                          }
                          frame True {
                            n237 = Index Array(array=w203, index=1) -> (element=w201:dbl)
                            n238 = Divide(x="length", y=2) -> (x/y=w198:dbl)
                            n239 = Subtract(x=w201, y=w198) -> (x-y=w199:dbl)
                            n240 = Array Subset(array=w200, index=w199, length="length") -> (w195:u32[])
                            "Waveform Graph 5" <- w195
                            n241 = Array Max & Min(array=w195) -> (max value=w192:u32)  [unwired: 3 out]
                            "max value" <- w192
                            "ADC_PEAK" <- w192
                            n242 = Build Array (concatenate)(w194, w192) -> (w193:u32[])
                          }
                        }
                      }
                      frame #1 {
                        n243 = global read "LBNE_Global .vi" "LBNE_REF"() -> (w208:refnum<k24>)
                        n244 = property class="LBNE_COMM"(reference=w208, "LV_READY"=FALSE) -> ()  [unwired: 1 in, 2 out]
                      }
                    }
                  }
                }
                n245 = local read "CHANNEL"() -> (w125:u8)
                n246 = Index Array(array=w123, index (row)=w125) -> (element=w126:u32[])  [unwired: 1 in]
                n247 = Array Max & Min(array=w126) -> ()  [unwired: 4 out]
                n248 = Array Subset(array=w126, length=4096) -> ()  [unwired: 1 in, 1 out]
              }
              frame #1 {
              }
            }
            n249 = case shown="True" "SAVE TO \nFILE" {
              frame False {
              }
              frame True {
                n250 = local read "Store_Data"() -> (w210:bool)
                n251 = case shown="False" w210 {
                  frame False {
                    n252 = stacked-sequence {
                      seq-local: [w212 _] -> [_ w224]
                      seq-local: [w211 _] -> [_ w223]
                      frame #0 {
                        n253 = Concatenate Strings("FILE NAME 2", ".txt" ("string")) -> (w214:string)
                        n254 = Build Path(base path="FILE PATH", name or relative path=w214) -> (appended path=w212:path)
                        n255 = call <vilib>:"Check if File or Folder Exists.vi"("path"=w212) -> ("file or folder exists?"=w215:bool)  [unwired: 8 in, 2 out]
                        n256 = case shown="False" w215 {
                          tunnel: [TRUE ("T button?") w221] -> w211
                          frame False {
                          }
                          frame True {
                            n257 = Two Button Dialog(message="FILE EXISTS DO YOU \nWANT TO OVERWRITE", 1:"NO" ("F button name (\"Cancel\")"), 2:"YES" ("T button name (\"OK\")")) -> (T button?=w221:bool)
                          }
                        }
                      }
                      frame #1 {
                        n258 = Path To String(path=w224) -> (string=w225:string)
                        n259 = case shown="True" w223 {
                          tunnel: w225 -> [_ w227]
                          frame False {
                          }
                          frame True {
                            n260 = global read "LBNE_Global .vi" "LBNE_REF"() -> (w226:refnum<k24>)
                            n261 = invoke class="LBNE_COMM" method="open_file"(reference=w226, "File_name"=w227) -> ()  [unwired: 2 in, 4 out]
                          }
                        }
                      }
                    }
                  }
                  frame True {
                    n262 = global read "LBNE_Global .vi" "LBNE_REF"() -> (w228:refnum<k24>)
                    n263 = invoke class="LBNE_COMM" method="open_file"(reference=w228, "File_name"="") -> ()  [unwired: 2 in, 4 out]
                  }
                }
              }
            }
          }
          frame "LBNE AUTO CAL" {
            n264 = flat-sequence {
              tunnel: "START" -> [w405]
              tunnel: [w404] -> w400
              tunnel: [w402] -> w399
              tunnel: [w407] -> w398
              frame #0 {
                n265 = case shown="True" w405 {
                  tunnel: [FALSE ("YES") w415] -> w404
                  frame False {
                  }
                  frame True {
                    n266 = call "Display Message to User2"() -> ("YES"=w415:bool)  [unwired: 10 in, 1 out]
                  }
                }
                n267 = local write "Array 5"(dbl[] [] ("output array")) -> ()
                n268 = local read "setting"() -> (w411:u16)
                n269 = Number To Decimal String(number=w411, width (-)=i16 3) -> (decimal integer string=w409:string)
                n270 = Build Path(base path="FILE PATH 2", name or relative path=w409) -> (appended path=w408:path)
                n271 = call <vilib>:"Check if File or Folder Exists.vi"("path"=w408) -> ("file or folder exists?"=w413:bool)  [unwired: 8 in, 2 out]
                n272 = case shown="False" w413 {
                  tunnel: w408 -> [w417 w418]
                  tunnel: [w416 w418] -> w407
                  frame False {
                    n273 = Create Folder(path (use dialog)=w417) -> (created path=w416:path)  [unwired: 2 in, 2 out]
                  }
                  frame True {
                  }
                }
                n274 = local read "DLY"() -> (w403:u8)
                n275 = Number To Decimal String(number=w403) -> (decimal integer string=w402:string)  [unwired: 1 in]
              }
            }
            n276 = case shown="True" w400 {
              tunnel: w399 -> [_ w424]
              tunnel: w398 -> [_ w423]
              frame False {
                n277 = global read "LBNE_Global .vi" "LBNE_REF"() -> (w420:refnum<k24>)
                n278 = property class="LBNE_COMM"(reference=w420) -> ("Store_Data"=w419:bool)  [unwired: 1 in, 2 out]
                n279 = case shown="True" w419 {
                  frame False {
                  }
                  frame True {
                    n280 = global read "LBNE_Global .vi" "LBNE_REF"() -> (w422:refnum<k24>)
                    n281 = invoke class="LBNE_COMM" method="open_file"(reference=w422, "File_name"="") -> ()  [unwired: 2 in, 4 out]
                  }
                }
                n282 = local write "Store_Data 2"(w419) -> ()
              }
              frame True {
                n283 = while {
                  tunnel: w424 -> [w429]
                  tunnel: w423 -> [w428]
                  i -> [w431]
                  stop <- w426 stop-if-true
                  n284 = Not Equal?(x=0, y=w431) -> (x != y?=w432:bool)
                  n285 = stacked-sequence {
                    tunnel: w432 -> [w452 _ _ _]
                    tunnel: w431 -> [w450 _ _ _]
                    tunnel: [_ _ w516 _] -> w430
                    tunnel: w429 -> [_ _ _ w777]
                    tunnel: w428 -> [_ _ w515 w774]
                    frame #0 {
                      n286 = case shown="False" w452 {
                        tunnel: [FALSE ("Boolean") TRUE ("Boolean")] -> w451
                        tunnel: w450 -> [_ w470]
                        tunnel: [u8 0 ("AMPL 2") w469] -> w449
                        frame False {
                        }
                        frame True {
                          n287 = case shown="0, Default" w470 {
                            tunnel: [u8 0 ("AMPL 2") u8 1 ("AMPL 2") u8 2 ("AMPL 2") u8 3 ("AMPL 2") u8 4 ("AMPL 2") u8 5 ("AMPL 2") u8 6 ("AMPL 2") u8 7 ("AMPL 2") u8 8 ("AMPL 2") u8 9 ("AMPL 2") u8 10 ("AMPL 2") u8 11 ("AMPL 2") u8 12 ("AMPL 2") u8 13 ("AMPL 2") u8 14 ("AMPL 2") u8 15 ("AMPL 2") u8 16 ("AMPL 2") u8 17 ("AMPL 2") u8 18 ("AMPL 2") u8 19 ("AMPL 2") u8 20 ("AMPL 2") u8 21 ("AMPL 2") u8 22 ("AMPL 2") u8 23 ("AMPL 2") u8 24 ("AMPL 2") u8 25 ("AMPL 2") u8 26 ("AMPL 2") u8 27 ("AMPL 2") u8 28 ("AMPL 2") u8 29 ("AMPL 2") u8 30 ("AMPL 2") u8 31 ("AMPL 2")] -> w469
                            frame 0, Default {
                              n288 = call "Display Message to User"() -> ()  [unwired: 10 in, 2 out]
                            }
                            frame 1 {
                            }
                            frame 2 {
                            }
                            frame 3 {
                            }
                            frame 4 {
                            }
                            frame 5 {
                            }
                            frame 6 {
                            }
                            frame 7 {
                            }
                            frame 8 {
                            }
                            frame 9 {
                            }
                            frame 10 {
                            }
                            frame 11 {
                            }
                            frame 12 {
                            }
                            frame 13 {
                            }
                            frame 14 {
                            }
                            frame 15 {
                            }
                            frame 16 {
                            }
                            frame 17 {
                            }
                            frame 18 {
                            }
                            frame 19 {
                            }
                            frame 20 {
                            }
                            frame 21 {
                            }
                            frame 22 {
                            }
                            frame 23 {
                            }
                            frame 24 {
                            }
                            frame 25 {
                            }
                            frame 26 {
                            }
                            frame 27 {
                            }
                            frame 28 {
                            }
                            frame 29 {
                            }
                            frame 30 {
                            }
                            frame 31 {
                            }
                          }
                        }
                      }
                      n289 = flat-sequence {
                        tunnel: w449 -> [w453]
                        tunnel: w451 -> [w459]
                        frame #0 {
                          n290 = local read "DLY"() -> (w455:u8)
                          n291 = Join Numbers(hi=w455, lo=w453) -> ((hi.lo)=w457:u16)
                          n292 = local read "FREQ 2"() -> (w454:u16)
                          n293 = Join Numbers(hi=w454, lo=w457) -> ((hi.lo)=w456:u32)
                          n294 = call "wr_lbne.vi"("DATA"=w456, "ADDRESS"=u16 5) -> ()  [unwired: 1 out]
                          "AMPL 2" <- w453
                        }
                        frame #1 {
                          n295 = Boolean To (0,1)(Boolean=w459) -> (0, 1=w463:i16)
                          n296 = Boolean To (0,1)(Boolean=TRUE) -> (0, 1=w465:i16)
                          n297 = To Unsigned Byte Integer(number=w465) -> (unsigned 8bit integer=w466:u8)
                          n298 = To Unsigned Byte Integer(number=w463) -> (unsigned 8bit integer=w464:u8)
                          n299 = Join Numbers(hi=w466, lo=w464) -> ((hi.lo)=w462:u16)
                          n300 = call "wr_lbne.vi"("DATA"=w462, "ADDRESS"=u16 16) -> ()  [unwired: 1 out]
                          "TP enable" <- w459
                        }
                      }
                    }
                    frame #1 {
                      w505 = 16 ("dimension size")
                      n301 = global read "LBNE_Global .vi" "LBNE_REF"() -> (w510:refnum<k24>)
                      n302 = global read "LBNE_Global .vi" "LBNE_REF"() -> (w509:refnum<k24>)
                      n303 = Initialize Array(0.0 ("element"), w505, w505) -> (w506:dbl[][])
                      n304 = local write "MEAN"(w506) -> ()
                      n305 = local write "RMS"(w506) -> ()
                      n306 = property class="LBNE_COMM"(reference=w509) -> ("Store_Data"=w508:bool)  [unwired: 1 in, 2 out]
                      "Store_Data 2" <- w508
                      n307 = property class="LBNE_COMM"(reference=w510, "HIST_samples"=u32 0) -> ()  [unwired: 1 in, 2 out]
                      n308 = case shown="True" w508 {
                        frame False {
                        }
                        frame True {
                          n309 = global read "LBNE_Global .vi" "LBNE_REF"() -> (w514:refnum<k24>)
                          n310 = invoke class="LBNE_COMM" method="open_file"(reference=w514, "File_name"="") -> ()  [unwired: 2 in, 4 out]
                        }
                      }
                      "CUR_CHN" <- "Start channel"
                      "CUR_CHP" <- "Start chip"
                    }
                    frame #2 {
                      n311 = while {
                        tunnel: [w519] -> w516
                        tunnel: w515 -> [w517]
                        stop <- w518 stop-if-true
                        n312 = stacked-sequence {
                          tunnel: [_ _ w580 _ _] -> w519
                          tunnel: [_ _ _ _ w758] -> w520
                          tunnel: w517 -> [w521 _ w576 _ _]
                          frame #0 {
                            n313 = global read "LBNE_Global .vi" "LBNE_REF"() -> (w525:refnum<k24>)
                            n314 = local read "CUR_CHN"() -> (w524:u8)
                            n315 = local read "CUR_CHP"() -> (w523:u8)
                            n316 = case shown="True" "SAVE TO \nFILE 2" {
                              tunnel: w521 -> [_ w528]
                              frame False {
                              }
                              frame True {
                                n317 = local read "CUR_CHN"() -> (w533:u8)
                                n318 = local read "TP enable"() -> (w530:bool)
                                n319 = Equal To 0?(x=w533) -> (x = 0?=w532:bool)
                                n320 = Not(x=w530) -> (.not. x?=w529:bool)
                                n321 = And(x=w532, y=w529) -> (x .and. y?=w531:bool)
                                n322 = case shown="True" w531 {
                                tunnel: w528 -> [_ w534]
                                frame False {
                                }
                                frame True {
                                n323 = stacked-sequence {
                                tunnel: w534 -> [_ _ w540 _]
                                frame #0 {
                                n324 = global read "LBNE_Global .vi" "LBNE_REF"() -> (w536:refnum<k24>)
                                n325 = property class="LBNE_COMM"(reference=w536) -> ("Store_Data"=w535:bool)  [unwired: 1 in, 2 out]
                                n326 = case shown="True" w535 {
                                frame False {
                                }
                                frame True {
                                n327 = global read "LBNE_Global .vi" "LBNE_REF"() -> (w537:refnum<k24>)
                                n328 = invoke class="LBNE_COMM" method="open_file"(reference=w537, "File_name"="") -> ()  [unwired: 2 in, 4 out]
                                }
                                }
                                }
                                frame #1 {
                                n329 = Wait Until Next ms Multiple(millisecond multiple=u32 100) -> ()  [unwired: 1 out]
                                }
                                frame #2 {
                                n330 = Build Path(base path=w540, name or relative path="raw") -> (appended path=w542:path)
                                n331 = call <vilib>:"Check if File or Folder Exists.vi"("path"=w542) -> ("file or folder exists?"=w543:bool)  [unwired: 8 in, 2 out]
                                n332 = case shown="False" w543 {
                                tunnel: w542 -> [w554 w555]
                                tunnel: [w553 w555] -> w541
                                frame False {
                                n333 = Create Folder(path (use dialog)=w554) -> (created path=w553:path)  [unwired: 2 in, 2 out]
                                }
                                frame True {
                                }
                                }
                                n334 = local read "CUR_CHN"() -> (w545:u8)
                                n335 = local read "CUR_CHP"() -> (w547:u8)
                                n336 = Format Into String(format string="_CHIP%d_CHN%d.bin", initial string="FILE NAME 3", w547, w545) -> (resulting string=w549:string)  [unwired: 1 in, 1 out]
                                n337 = Build Path(base path=w541, name or relative path=w549) -> (appended path=w550:path)
                                n338 = global read "LBNE_Global .vi" "LBNE_REF"() -> (w552:refnum<k24>)
                                n339 = Path To String(path=w550) -> (string=w551:string)
                                n340 = invoke class="LBNE_COMM" method="open_file"(reference=w552, "File_name"=w551) -> ()  [unwired: 2 in, 4 out]
                                }
                                frame #3 {
                                n341 = Wait Until Next ms Multiple(millisecond multiple=u32 50) -> ()  [unwired: 1 out]
                                }
                                }
                                }
                                }
                              }
                            }
                            n342 = property class="LBNE_COMM"(reference=w525, "CHN_SEL"=w524) -> ()  [unwired: 1 in, 2 out]
                            n343 = Join Numbers(hi=w524, lo=w523) -> ((hi.lo)=w526:u16)
                            n344 = call "wr_lbne.vi"("DATA"=w526, "ADDRESS"=u16 7 ("address")) -> ()  [unwired: 1 out]
                          }
                          frame #1 {
                            n345 = global read "LBNE_Global .vi" "LBNE_REF"() -> (w561:refnum<k24>)
                            n346 = global read "LBNE_Global .vi" "LBNE_REF"() -> (w560:refnum<k24>)
                            n347 = local read "TP enable"() -> (w557:bool)
                            n348 = case shown="False" w557 {
                              tunnel: [u32 260050 ("number_of_samples 2") "number_of_samples 2"] -> w558
                              frame False {
                              }
                              frame True {
                              }
                            }
                            n349 = property class="LBNE_COMM"(reference=w560) -> ("Store_Data"=w559:bool)  [unwired: 1 in, 2 out]
                            n350 = property class="LBNE_COMM"(reference=w561, "LV_READY"=FALSE) -> ()  [unwired: 1 in, 2 out]
                            n351 = local write "Store_Data 2"(w559) -> ()
                            n352 = global read "LBNE_Global .vi" "LBNE_REF"() -> (w563:refnum<k24>)
                            n353 = Initialize Array(u32 0 ("element"), 16 ("dimension size"), 4096 ("dimension size")) -> (w567:u32[][])
                            n354 = Initialize Array(0.0 ("element"), 16 ("dimension size")) -> (w570:dbl[])
                            n355 = Initialize Array(u32 0 ("element"), 16 ("dimension size")) -> (w572:u32[])
                            n356 = property class="LBNE_COMM"(reference=w563, "ADC_hist"=w567, "ADC_avg"=w570, "ADC_savg"=w570, "ADC_samples"=w572, "number_of_samples"=w558) -> ()  [unwired: 1 in, 2 out]
                          }
                          frame #2 {
                            n357 = call "Elapsed Time"("Reset"=TRUE) -> ("Time has Elapsed"=→"Time has Elapsed":bool)  [unwired: 11 in, 7 out]
                            n358 = while {
                              tunnel: ["stop 2"] -> w580
                              shift-right: [w589] -> _
                              shift-left: u32[] [] ("subarray") -> [w590]
                              tunnel: w576 -> [w583]
                              i -> [w586]
                              stop <- w587 stop-if-true
                              n359 = global read "LBNE_Global .vi" "LBNE_REF"() -> (w582:refnum<k24>)
                              n360 = property class="LBNE_COMM"(reference=w582) -> ("LV_READY"=w581:bool)  [unwired: 1 in, 2 out]
                              n361 = case shown="True" w581 {
                                tunnel: [FALSE w596] -> w591
                                tunnel: w590 -> [w593 w602]
                                tunnel: [w593 w601] -> w589
                                tunnel: w583 -> [_ w595]
                                frame False {
                                }
                                frame True {
                                n362 = stacked-sequence {
                                tunnel: w602 -> [w610 _]
                                tunnel: [w611 _] -> w601
                                tunnel: [w605 _] -> w600
                                tunnel: w595 -> [w603 _]
                                frame #0 {
                                n363 = Array Size(array=w610) -> (size(s)=w607:i32)
                                "CNT" <- w607
                                n364 = Wait Until Next ms Multiple(millisecond multiple=u32 10) -> ()  [unwired: 1 out]
                                n365 = global read "LBNE_Global .vi" "LBNE_REF"() -> (w617:refnum<k24>)
                                n366 = property class="LBNE_COMM"(reference=w617) -> ("receive_word_array"=w608:u32[], "ADC_hist"=w616:u32[][], "ADC_samples"=w615:u32[])  [unwired: 1 in, 2 out]
                                "Waveform Graph 7" <- w608
                                n367 = local read "CUR_CHN"() -> (w614:u8)
                                n368 = local read "TP enable"() -> (w609:bool)
                                n369 = case shown="False" w609 {
                                tunnel: w608 -> [w684 _]
                                tunnel: w603 -> [w670 _]
                                frame False {
                                n370 = Build Path(base path=w670, name or relative path="FFT") -> (appended path=w672:path)
                                n371 = Array Subset(array=w684, index=5000, length=250000) -> (w678:u32[])
                                n372 = call <vilib>:"Check if File or Folder Exists.vi"("path"=w672) -> ("file or folder exists?"=w673:bool)  [unwired: 8 in, 2 out]
                                n373 = call "Convert to Dynamic Data6"("Array"=w678) -> ("Dynamic Data Type"=w677:dynamicdata)  [unwired: 3 in]
                                n374 = case shown="True" w673 {
                                tunnel: w672 -> [w687 w688]
                                tunnel: [w686 w688] -> w671
                                frame False {
                                n375 = Create Folder(path (use dialog)=w687) -> (created path=w686:path)  [unwired: 2 in, 2 out]
                                }
                                frame True {
                                }
                                }
                                n376 = for {
                                N: 50 -> [_]
                                tunnel: w678 -> [w709]
                                tunnel: [w703] -> w681
                                i -> [w701]
                                n377 = Multiply(x=w701, y=5000) -> (x*y=w707:i32)
                                n378 = Array Subset(array=w709, index=w707, length=5000) -> (w704:u32[])
                                n379 = Bundle By Name("Y"=w704, "dt"=5e-07) -> (w702:waveform(u32))  [unwired: 1 in]
                                n380 = Equal To 0?(x=w701) -> (x = 0?=w700:bool)
                                n381 = xnode "Spectral Measurements 2"("Signals"=w702, "Restart Averaging"=w700) -> ("Power Spectrum"=w703:dynamicdata)  [unwired: 1 in, 2 out]
                                }
                                n382 = local read "CUR_CHN"() -> (w667:u8)
                                n383 = local read "CUR_CHP"() -> (w669:u8)
                                n384 = Increment(x=w669) -> (x+1=w668:u8)
                                n385 = Increment(x=w667) -> (x+1=w666:u8)
                                n386 = Format Into String(format string="_CHIP%d_CHN%d.xlsx", initial string="FILE NAME 4", w668, w666) -> (resulting string=w676:string)  [unwired: 1 in, 1 out]
                                n387 = Build Path(base path=w671, name or relative path=w676) -> (appended path=w675:path)
                                n388 = flat-sequence {
                                tunnel: w681 -> [w693]
                                tunnel: w676 -> [w692]
                                tunnel: w675 -> [w695]
                                frame #0 {
                                n389 = property on="FFT Analysis" class="WFGraph (strict)"("Plot.Plot Name"=w692) -> ()  [unwired: 2 in, 2 out]
                                "FFT Analysis" <- w693
                                }
                                frame #1 {
                                n390 = case shown="True" TRUE {
                                tunnel: w695 -> [_ w699]
                                frame False {
                                }
                                frame True {
                                n391 = invoke on="FFT Analysis" class="WFGraph (strict)" method="Export Image"("FileType"=enum32{"BMP", "EPS", "EMF", "PICT"}."BMP" ("File Type"), "Target"=enum32{"File", "Clipboard"}."File", "Path"=w699, "Overwrite"=TRUE ("Always Overwrite")) -> ()  [unwired: 4 in, 8 out]
                                }
                                }
                                }
                                }
                                n392 = case shown="True" "fft save" {
                                tunnel: w677 -> [_ w691]
                                tunnel: w675 -> [_ w690]
                                frame False {
                                }
                                frame True {
                                n393 = call "Write To Measurement File3"("Signals"=w691, "Enable"=TRUE, "Filename"=w690) -> ()  [unwired: 14 in, 3 out]
                                }
                                }
                                }
                                frame True {
                                }
                                }
                                n394 = Index Array(array=w616, index (row)=w614) -> ()  [unwired: 1 in, 1 out]
                                n395 = Index Array(array=w615, index=w614) -> (element=→"samples 5":u32)
                                n396 = Array Size(array=w608) -> (size(s)=w606:i32)
                                "samples received" <- w606
                                n397 = local read "TP enable"() -> (w604:bool)
                                n398 = case shown="False" w604 {
                                tunnel: [w627 w633] -> w611
                                tunnel: w610 -> [w627 w631]
                                tunnel: w608 -> [w621 w629]
                                tunnel: [w626 w628] -> w605
                                tunnel: w607 -> [_ w628]
                                tunnel: w606 -> [w626 _]
                                frame False {
                                n399 = Array Subset(array=w621, index=5000, length=250000) -> (w618:u32[])
                                n400 = call "Convert to Dynamic Data5"("Array"=w618) -> ("Dynamic Data Type"=w623:dynamicdata)  [unwired: 3 in]
                                n401 = call "Statistics3"("Signals"=w623) -> ("Total Samples"=w622:dynamicdata, "Standard Dev"=→"peds rms":dynamicdata, "Arithmetic Mean"=→"peds Mean":dynamicdata)  [unwired: 23 in, 1 out]
                                n402 = local write "ADC_CNT 2"(w622) -> ()
                                }
                                frame True {
                                n403 = Array Max & Min(array=w629) -> (max value=w635:u32)  [unwired: 3 out]
                                n404 = Subtract(x=w635, y="com") -> (x-y=w639:u32)
                                n405 = call <vilib>:"Peak Detector.vi"("peaks/valleys"=enum32{"Peaks", "Valleys"}."Peaks", "width"=3, "threshold"=w639, "X"=w629) -> ("Amplitudes"=w634:dbl[], "Locations"=w637:dbl[], "# found"=w630:i32)  [unwired: 3 in, 2 out]
                                n406 = Greater Or Equal?(x=w630, y=3 ("x")) -> (x >= y?=w638:bool)
                                n407 = case shown="False" w638 {
                                tunnel: w637 -> [_ w645]
                                tunnel: w629 -> [_ w655]
                                tunnel: w634 -> [_ w643]
                                tunnel: w631 -> [w642 w650]
                                tunnel: [w642 w649] -> w633
                                tunnel: w630 -> [_ _]
                                frame False {
                                }
                                frame True {
                                w651 = 40 ("length 2")
                                n408 = Build Array (concatenate)(w650, w643) -> (w649:dbl[])
                                n409 = Array Size(array=w649) -> (size(s)=w648:i32)
                                n410 = Divide(x=w651, y=2) -> (x/y=w653:dbl)
                                n411 = Index Array(array=w645, index=1) -> (element=w656:dbl)
                                n412 = Subtract(x=w656, y=w653) -> (x-y=w654:dbl)
                                n413 = Greater?(x=w648, y=5) -> (0:w646:bool)
                                n414 = Array Subset(array=w655, index=w654, length=w651) -> (→"Waveform Graph 6":u32[])
                                n415 = case shown="True" w646 {
                                tunnel: w649 -> [_ w663]
                                frame False {
                                }
                                frame True {
                                n416 = Array Subset(array=w663, index=4) -> (w661:dbl[])  [unwired: 1 in]
                                n417 = call "Convert to Dynamic Data2"("Array"=w661) -> ("Dynamic Data Type"=w664:dynamicdata)  [unwired: 3 in]
                                n418 = call "Statistics2"("Signals"=w664) -> ("Total Samples"=→"ADC_CNT 2":dynamicdata, "Standard Dev"=→"ADC_RMS 2":dynamicdata, "Arithmetic Mean"=→"ADC_MEAN 2":dynamicdata)  [unwired: 23 in, 1 out]
                                }
                                }
                                }
                                }
                                }
                                }
                                }
                                frame #1 {
                                n419 = global read "LBNE_Global .vi" "LBNE_REF"() -> (w720:refnum<k24>)
                                n420 = property class="LBNE_COMM"(reference=w720, "LV_READY"=FALSE) -> ()  [unwired: 1 in, 2 out]
                                }
                                }
                                n421 = Add(x="Caculation", y=u32 5) -> (x+y=w598:u32)
                                n422 = Greater Or Equal?(x=w600, y=w598) -> (x >= y?=w596:bool)
                                }
                              }
                              n423 = Greater?(x=w586, y=30000) -> (0:w584:bool)
                              n424 = Or(x=w591, y="stop 2") -> (x .or. y?=w588:bool)
                              n425 = Or(x=w588, y=w584) -> (x .or. y?=w587:bool)
                              "loop cnt" <- w586
                            }
                          }
                          frame #3 {
                            n426 = local read "TP enable"() -> (w745:bool)
                            n427 = case shown="False" w745 {
                              tunnel: [w754 w757] -> w727
                              tunnel: [w755 w756] -> w744
                              frame False {
                                n428 = local read "peds Mean"() -> (w755:dbl)
                                n429 = local read "peds rms"() -> (w754:dbl)
                              }
                              frame True {
                                n430 = local read "ADC_MEAN 2"() -> (w756:dbl)
                                n431 = local read "ADC_RMS 2"() -> (w757:dbl)
                              }
                            }
                            n432 = local read "CUR_CHN"() -> (w733:u8)
                            n433 = local read "CUR_CHP"() -> (w731:u8)
                            n434 = local read "MEAN"() -> (w747:dbl[][])
                            n435 = local read "RMS"() -> (w746:dbl[][])
                            n436 = Equal?(x=w731, y=1 ("index (row)")) -> (x = y?=w730:bool)
                            n437 = Equal?(x=w733, y=15 ("disabled index (col)")) -> (x = y?=w729:bool)
                            n438 = local read "Array 5"() -> (w726:dbl[])
                            n439 = And(x=w730, y=w729) -> (x .and. y?=w728:bool)
                            n440 = Replace Array Subset(array=w747, new element=w744, index (row)=w733, index (col)=w731) -> (→"MEAN":dbl[][])
                            n441 = Replace Array Subset(array=w746, new element=w727, index (row)=w733, index (col)=w731) -> (w743:dbl[][])
                            "RMS" <- w743
                            n442 = case shown="False" w728 {
                              tunnel: w727 -> [w751 _]
                              tunnel: [w749 w753] -> w723
                              tunnel: w726 -> [w752 w753]
                              frame False {
                                n443 = Insert Into Array(array=w752, index=0, new element=w751) -> (w749:dbl[])
                              }
                              frame True {
                              }
                            }
                            "Array 5" <- w723
                            n444 = Index Array(array=w743, index (row)=14 ("disabled index (col)"), index (col)=1 ("index (row)")) -> (element=w742:dbl)
                            n445 = local read "gain electrons"() -> (w725:u16)
                            n446 = Replace Array Subset(array=w743, new element=w742, index (row)=15 ("disabled index (col)"), index (col)=1 ("index (row)")) -> (w741:dbl[][])
                            n447 = Multiply(x=w725, y=w723) -> (x*y=w724:dbl[])
                            n448 = Multiply(x=w741, y=w725) -> (x*y=→"ENC":dbl[][])
                            n449 = Array Size(array=w723) -> (size(s)=→"size(s) 3":i32)
                            n450 = call-poly <vilib>:"Mean.vi"("X"=w724) -> ("mean"=→"Average of all CHNS":dbl)  [unwired: 1 out]
                          }
                          frame #4 {
                            n451 = flat-sequence {
                              tunnel: [w768] -> w758
                              frame #0 {
                                n452 = local read "CUR_CHN"() -> (w762:u8)
                                n453 = Increment(x=w762) -> (x+1=w761:u8)
                                n454 = Greater Or Equal?(x=w761, y=u8 16) -> (x >= y?=w760:bool)
                                n455 = case shown="True" w760 {
                                frame False {
                                n456 = local read "CUR_CHN"() -> (w764:u8)
                                n457 = Increment(x=w764) -> (x+1=w763:u8)
                                n458 = local write "CUR_CHN"(w763) -> ()
                                }
                                frame True {
                                n459 = local read "CUR_CHP"() -> (w766:u8)
                                n460 = local write "CUR_CHN"(u8 0 ("CUR_CHN")) -> ()
                                n461 = Increment(x=w766) -> (x+1=w765:u8)
                                n462 = local write "CUR_CHP"(w765) -> ()
                                }
                                }
                              }
                              frame #1 {
                                n463 = local read "CUR_CHP"() -> (w770:u8)
                                n464 = Greater Or Equal?(x=w770, y=u8 8) -> (x >= y?=w768:bool)
                              }
                            }
                          }
                        }
                        n465 = Or(x=w519, y=w520) -> (x .or. y?=w518:bool)
                      }
                    }
                    frame #3 {
                      n466 = Concatenate Strings(w777, ".xlsx" ("string")) -> (w778:string)
                      n467 = Concatenate Strings("test_mean_" ("File_name"), w778) -> (w773:string)
                      n468 = local read "MEAN"() -> (w783:dbl[][])
                      n469 = Build Path(base path=w774, name or relative path=w773) -> (appended path=w772:path)
                      n470 = Concatenate Strings("test_rms_" ("File_name"), w778) -> (w776:string)
                      n471 = local read "RMS"() -> (w771:dbl[][])
                      n472 = call "Convert to Dynamic Data4"("2D Array"=w783) -> ("Dynamic Data Type"=w782:dynamicdata)  [unwired: 3 in]
                      n473 = call "Write To Measurement File"("Signals"=w782, "Filename"=w772) -> ()  [unwired: 15 in, 3 out]
                      n474 = Build Path(base path=w774, name or relative path=w776) -> (appended path=w775:path)
                      n475 = call "Convert to Dynamic Data3"("2D Array"=w771) -> ("Dynamic Data Type"=w784:dynamicdata)  [unwired: 3 in]
                      n476 = call "Write To Measurement File2"("Signals"=w784, "Filename"=w775) -> ()  [unwired: 15 in, 3 out]
                    }
                  }
                  n477 = Equal?(x="AMPL2 END", y=w431) -> (x = y?=w427:bool)
                  n478 = Or(x=w430, y=w427) -> (x .or. y?=w426:bool)
                  n479 = case shown="True" w426 {
                    frame False {
                    }
                    frame True {
                      n480 = flat-sequence {
                        tunnel: u32 10000 ("number_of_samples") -> [w435]
                        frame #0 {
                          n481 = global read "LBNE_Global .vi" "LBNE_REF"() -> (w436:refnum<k24>)
                          n482 = global read "LBNE_Global .vi" "LBNE_REF"() -> (w438:refnum<k24>)
                          n483 = Initialize Array(u32 0 ("element"), 16 ("dimension size"), 4096 ("dimension size")) -> (w442:u32[][])
                          n484 = Initialize Array(0.0 ("element"), 16 ("dimension size")) -> (w445:dbl[])
                          n485 = Initialize Array(u32 0 ("element"), 16 ("dimension size")) -> (w447:u32[])
                          n486 = property class="LBNE_COMM"(reference=w438, "ADC_hist"=w442, "ADC_avg"=w445, "ADC_savg"=w445, "ADC_samples"=w447, "number_of_samples"=w435) -> ()  [unwired: 1 in, 2 out]
                          n487 = property class="LBNE_COMM"(reference=w436, "LV_READY"=FALSE) -> ()  [unwired: 1 in, 2 out]
                        }
                      }
                    }
                  }
                }
              }
            }
          }
          frame "FPGA FLASH" {
            n488 = case shown="False" "erase flash" {
              frame False {
              }
              frame True {
                n489 = flat-sequence {
                  frame #0 {
                    n490 = call "wr_lbne.vi"("DATA"=u32 1, "ADDRESS"=u16 13) -> ()  [unwired: 1 out]
                    n491 = call "wr_lbne.vi"("DATA"=u32 1, "ADDRESS"=u16 9) -> ()  [unwired: 1 out]
                  }
                  frame #1 {
                    # "erase flash"
                    n492 = stacked-sequence {
                      frame #0 {
                        n493 = call "wr_lbne.vi"("DATA"=u32 6, "ADDRESS"=u16 10) -> ()  [unwired: 1 out]
                      }
                      frame #1 {
                        n494 = call "wr_lbne.vi"("DATA"=u32 262, "ADDRESS"=u16 10) -> ()  [unwired: 1 out]
                      }
                      frame #2 {
                        n495 = call "wr_lbne.vi"("DATA"=u32 0, "ADDRESS"=u16 10) -> ()  [unwired: 1 out]
                      }
                    }
                  }
                  frame #2 {
                    w1033 = u32 199  # opcode
                    # "wait for clear flash"
                    n496 = call "wr_lbne.vi"("DATA"=w1033, "ADDRESS"=u16 10) -> ()  [unwired: 1 out]
                    n497 = Wait Until Next ms Multiple(millisecond multiple=u32 5) -> ()  [unwired: 1 out]
                  }
                  frame #3 {
                    n498 = stacked-sequence {
                      frame #0 {
                        w1036 = u32 455  # opcode
                        n499 = call "wr_lbne.vi"("DATA"=w1036, "ADDRESS"=u16 10) -> ()  [unwired: 1 out]
                      }
                      frame #1 {
                        n500 = Wait Until Next ms Multiple(millisecond multiple=u32 1) -> ()  [unwired: 1 out]
                      }
                      frame #2 {
                        w1039 = u32 199  # opcode
                        n501 = call "wr_lbne.vi"("DATA"=w1039, "ADDRESS"=u16 10) -> ()  [unwired: 1 out]
                      }
                    }
                  }
                  frame #4 {
                    n502 = call "wr_lbne.vi"("DATA"=u32 0, "ADDRESS"=u16 10) -> ()  [unwired: 1 out]
                    n503 = Wait Until Next ms Multiple(millisecond multiple=u32 1000) -> ()  [unwired: 1 out]
                  }
                }
              }
            }
            n504 = case shown="False" "LOAD RPD" {
              frame False {
              }
              frame True {
                w879 = "Choose Binary File"  # Prompt
                n505 = File Dialog(6:"*.rpd" ("pattern (all files)"), 7:w879) -> (0:w883:errorcluster, 3:w878:path)  [unwired: 5 in, 2 out]
                n506 = Open/Create/Replace File(file path (use dialog)=w878, error in=w883, operation (0:open)=T13."open", access (0:read/write)=enum16{"read/write", "read-only", "write-only"}."read-only") -> (refnum out=w886:refnum<file>, error out=w885:errorcluster)  [unwired: 2 in, 1 out]
                n507 = Deny Access(4:w885, 6:T14."deny write-only" ("deny mode (0:deny read/write)"), 7:w886) -> (0:w887:errorcluster, 3:w888:refnum<file>)
                n508 = Get File Size(file=w888, error in=w887) -> (refnum out=w876:refnum<file>, size (in bytes)=w871:i64, 0:w881:errorcluster)
                n509 = Divide(x=w871, y=i64 4) -> (x/y=w869:dbl)
                n510 = Read from Binary File(5:u32 0 ("y"), 8:w881, 10:w869, 11:w876) -> (0:w880:errorcluster, 2:w867:u32[], 3:w877:refnum<file>)  [unwired: 2 in, 1 out]
                n511 = Divide(x=w869, y=u32 64) -> (x/y=w873:dbl)
                n512 = Close File(refnum=w877, error in=w880) -> (error out=→"error out 2":errorcluster)  [unwired: 1 out]
                n513 = Increment(x=w873) -> (x+1=w868:dbl)
                "pages 2" <- w868
                n514 = for {
                  N: w868 -> [_]
                  tunnel: w867 -> [w896]
                  tunnel: [w895] -> w874 mode=indexing
                  i -> [w894]
                  w893 = 64 ("length")
                  n515 = Multiply(x=w893, y=w894) -> (x*y=w892:i32)
                  n516 = Array Subset(array=w896, index=w892, length=w893) -> (w895:u32[])
                }
                "FROM FILE" <- w874
              }
            }
            n517 = case shown="False" "READ STATUS" {
              frame False {
              }
              frame True {
                n518 = flat-sequence {
                  frame #0 {
                    n519 = call "wr_lbne.vi"("DATA"=u32 1, "ADDRESS"=u16 13) -> ()  [unwired: 1 out]
                    n520 = call "wr_lbne.vi"("DATA"=u32 1, "ADDRESS"=u16 9) -> ()  [unwired: 1 out]
                  }
                  frame #1 {
                    n521 = call "wr_lbne.vi"("DATA"=u32 5, "ADDRESS"=u16 10) -> ()  [unwired: 1 out]
                  }
                  frame #2 {
                    n522 = stacked-sequence {
                      frame #0 {
                        n523 = call "wr_lbne.vi"("DATA"=u32 261, "ADDRESS"=u16 10) -> ()  [unwired: 1 out]
                      }
                      frame #1 {
                        n524 = Wait Until Next ms Multiple(millisecond multiple=u32 1) -> ()  [unwired: 1 out]
                      }
                      frame #2 {
                        n525 = call "wr_lbne.vi"("DATA"=u32 5, "ADDRESS"=u16 10) -> ()  [unwired: 1 out]
                      }
                    }
                  }
                  frame #3 {
                    n526 = call "rd_lbne.vi"("ADDRESS 2"=i16 12) -> ("DATA 2"=→"DATA 5":u32)
                  }
                }
              }
            }
            n527 = case shown="False" "read flash" {
              frame False {
              }
              frame True {
                n528 = for {
                  N: "PAGES" -> [_]
                  tunnel: "P OFFSET" -> [w796]
                  shift-right: [w795] -> _
                  shift-left: u32[][] [] -> [w794]
                  i -> [w797]
                  n529 = Add(x=w796, y=w797) -> (x+y=w798:i32)
                  "PAGE" <- w798
                  n530 = Multiply(x=256 ("length"), y=w798) -> (x*y=w800:i32)
                  n531 = stacked-sequence {
                    tunnel: w800 -> [w801 _ _]
                    tunnel: [_ _ w810] -> w795
                    tunnel: w794 -> [_ _ w811]
                    frame #0 {
                      n532 = call "wr_lbne.vi"("DATA"=w801, "ADDRESS"=u16 11) -> ()  [unwired: 1 out]
                    }
                    frame #1 {
                      n533 = flat-sequence {
                        frame #0 {
                          w803 = u32 3  # opcode
                          n534 = call "wr_lbne.vi"("DATA"=w803, "ADDRESS"=u16 10) -> ()  [unwired: 1 out]
                        }
                        frame #1 {
                          w805 = u32 259  # opcode
                          n535 = call "wr_lbne.vi"("DATA"=w805, "ADDRESS"=u16 10) -> ()  [unwired: 1 out]
                        }
                        frame #2 {
                          w807 = u32 0  # opcode
                          n536 = call "wr_lbne.vi"("DATA"=w807, "ADDRESS"=u16 10) -> ()  [unwired: 1 out]
                        }
                        frame #3 {
                          n537 = Wait Until Next ms Multiple(millisecond multiple=u32 1) -> ()  [unwired: 1 out]
                        }
                      }
                    }
                    frame #2 {
                      n538 = for {
                        N: 4 -> [_]
                        shift-right: [w817] -> w812
                        shift-left: u32[] [] ("DATA") -> [w818]
                        i -> [w820]
                        n539 = Multiply(x=16, y=w820) -> (x*y=w821:i32)
                        n540 = Add(x=u32 128, y=w821) -> (x+y=w815:u32)
                        n541 = call "rd_lbne_BLK.vi"("ADDRESS 2"=w815) -> ("Array"=w816:u32[])
                        n542 = Build Array (concatenate)(w818, w816) -> (w817:u32[])
                      }
                      n543 = Build Array (concatenate)(w811, w812) -> (w810:u32[][])
                      "READ FROM FLASH" <- w810
                    }
                  }
                }
              }
            }
            n544 = case shown="False" "verify\nFLASH" {
              frame False {
              }
              frame True {
                n545 = local read "FROM FILE"() -> (w823:u32[][])
                n546 = for {
                  tunnel: w823 -> [w829]
                  tunnel: "start from" -> [w825]
                  tunnel: w823 -> [_] mode=indexing
                  i -> [w827]
                  stop <- w831 continue-if-true
                  n547 = Index Array(array=w829) -> (element=w828:u32[])  [unwired: 2 in]
                  n548 = Add(x=w825, y=w827) -> (x+y=w826:i32)
                  "PAGE 2" <- w826
                  n549 = local read "pages 2"() -> (w837:dbl)
                  n550 = Divide(x=w826, y=w837) -> (x/y=w835:dbl)
                  n551 = Multiply(x=256 ("length"), y=w826) -> (x*y=w839:i32)
                  n552 = stacked-sequence {
                    seq-local: [_ w842 _] -> [_ _ w865]
                    tunnel: w828 -> [_ _ w862]
                    tunnel: w839 -> [w840 _ _]
                    tunnel: [_ _ w866] -> w830
                    frame #0 {
                      n553 = call "wr_lbne.vi"("DATA"=w840, "ADDRESS"=u16 11) -> ()  [unwired: 1 out]
                    }
                    frame #1 {
                      n554 = stacked-sequence {
                        tunnel: [_ _ _ _ w850] -> w842
                        frame #0 {
                          w843 = u32 3  # opcode
                          n555 = call "wr_lbne.vi"("DATA"=w843, "ADDRESS"=u16 10) -> ()  [unwired: 1 out]
                        }
                        frame #1 {
                          w845 = u32 259  # opcode
                          n556 = call "wr_lbne.vi"("DATA"=w845, "ADDRESS"=u16 10) -> ()  [unwired: 1 out]
                        }
                        frame #2 {
                          w847 = u32 0  # opcode
                          n557 = call "wr_lbne.vi"("DATA"=w847, "ADDRESS"=u16 10) -> ()  [unwired: 1 out]
                        }
                        frame #3 {
                          n558 = Wait Until Next ms Multiple(millisecond multiple=u32 10) -> ()  [unwired: 1 out]
                        }
                        frame #4 {
                          n559 = for {
                            N: 4 -> [_]
                            shift-right: [w855] -> w850
                            shift-left: u32[] [] ("DATA") -> [w856]
                            i -> [w858]
                            n560 = Multiply(x=16, y=w858) -> (x*y=w859:i32)
                            n561 = Add(x=u32 128, y=w859) -> (x+y=w854:u32)
                            n562 = call "rd_lbne_BLK.vi"("ADDRESS 2"=w854) -> ("Array"=w853:u32[])
                            n563 = Build Array (concatenate)(w856, w853) -> (w855:u32[])
                          }
                        }
                      }
                    }
                    frame #2 {
                      n564 = Select(t=u32[] [4294967295, 4294967295, 4294967295, 4294967295, 4294967295, 4294967295, 4294967295, 4294967295, 4294967295, 4294967295, 4294967295, 4294967295, 4294967295, 4294967295, 4294967295, 4294967295, 4294967295, 4294967295, 4294967295, 4294967295, 4294967295, 4294967295, 4294967295, 4294967295, 4294967295, 4294967295, 4294967295, 4294967295, 4294967295, 4294967295, 4294967295, 4294967295, 4294967295, 4294967295, 4294967295, 4294967295, 4294967295, 4294967295, 4294967295, 4294967295, 4294967295, 4294967295, 4294967295, 4294967295, 4294967295, 4294967295, 4294967295, 4294967295, 4294967295, 4294967295, 4294967295, 4294967295, 4294967295, 4294967295, 4294967295, 4294967295, 4294967295, 4294967295, 4294967295, 4294967295, 4294967295, 4294967295, 4294967295, 4294967295] ("READ ARRAY 4"), s="blank check", f=w862) -> (s? t:f=w864:u32[])
                      "WRITE ARRAY 2" <- w864
                      n565 = Equal?(x=w865, y=w864) -> (x = y?=w866:bool)
                      "x = y? 2" <- w866
                      "READ ARRAY 3" <- w865
                    }
                  }
                  n566 = Multiply(x=100.0, y=w835) -> (x*y=→"Meter 2":dbl)
                  n567 = Not(x="STOP VERIFY") -> (.not. x?=w832:bool)
                  n568 = And(x=w830, y=w832) -> (x .and. y?=w831:bool)
                }
              }
            }
            n569 = case shown="True" "program \nFLASH" {
              frame False {
              }
              frame True {
                n570 = stacked-sequence {
                  frame #0 {
                    n571 = local write "NUM ATTEMP"(0 ("NUM ATTEMP")) -> ()
                    n572 = call "wr_lbne.vi"("DATA"=u32 1, "ADDRESS"=u16 13) -> ()  [unwired: 1 out]
                    n573 = local write "PAGE 3"("START FROM") -> ()
                    n574 = call "wr_lbne.vi"("DATA"=u32 1, "ADDRESS"=u16 9) -> ()  [unwired: 1 out]
                    "ONE_MORE" <- -1 ("ONE_MORE")
                  }
                  frame #1 {
                    n575 = local read "FROM FILE"() -> (w905:u32[][])
                    n576 = while {
                      tunnel: w905 -> [w913]
                      tunnel: "Numeric" -> [w914]
                      stop <- w906 continue-if-true
                      n577 = local read "PAGE 3"() -> (w907:i32)
                      n578 = Divide(x=w907, y=w914) -> (x/y=w916:dbl)
                      n579 = Index Array(array=w913, index (row)=w907) -> (element=w912:u32[])  [unwired: 1 in]
                      n580 = Multiply(x=256 ("length"), y=w907) -> (x*y=w918:i32)
                      n581 = stacked-sequence {
                        seq-local: [w919 _ _ _ _ _] -> [_ _ _ _ _ w991]
                        seq-local: [_ _ _ _ w969 _] -> [_ _ _ _ _ w990]
                        tunnel: w912 -> [w920 _ _ _ _ _]
                        tunnel: w918 -> [_ _ w947 _ _ _]
                        tunnel: [_ _ _ _ _ w989] -> w911
                        frame #0 {
                          n582 = while {
                            tunnel: w920 -> [w926]
                            tunnel: [w923] -> w919
                            stop <- w921 stop-if-true
                            (unwired) FALSE
                            # "load fifo"
                            n583 = for {
                              tunnel: w926 -> [w936] mode=indexing
                              tunnel: [w936] -> w923 mode=indexing
                              tunnel: [4] -> w922
                              i -> [w938]
                              n584 = Add(x=u32 64, y=w938) -> (x+y=w937:u32)
                              n585 = call "wr_lbne.vi"("DATA"=w936, "ADDRESS"=w937) -> ()  [unwired: 1 out]
                            }
                            n586 = for {
                              N: w922 -> [_]
                              shift-right: [w929] -> w924
                              shift-left: u32[] [] ("DATA") -> [w930]
                              i -> [w932]
                              n587 = Multiply(x=16, y=w932) -> (x*y=w933:i32)
                              n588 = Add(x=u32 64, y=w933) -> (x+y=w927:u32)
                              n589 = call "rd_lbne_BLK.vi"("ADDRESS 2"=w927) -> ("Array"=w928:u32[])
                              n590 = Build Array (concatenate)(w930, w928) -> (w929:u32[])
                            }
                            n591 = Equal?(x=w923, y=w924) -> (x = y?=w921:bool)
                            "x = y? 3" <- w921
                          }
                        }
                        frame #1 {
                          # "set write enable"
                          n592 = flat-sequence {
                            frame #0 {
                              n593 = call "wr_lbne.vi"("DATA"=u32 6, "ADDRESS"=u16 10) -> ()  [unwired: 1 out]
                            }
                            frame #1 {
                              n594 = stacked-sequence {
                                frame #0 {
                                n595 = call "wr_lbne.vi"("DATA"=u32 262, "ADDRESS"=u16 10) -> ()  [unwired: 1 out]
                                }
                                frame #1 {
                                n596 = Wait Until Next ms Multiple(millisecond multiple=u32 1) -> ()  [unwired: 1 out]
                                }
                                frame #2 {
                                n597 = call "wr_lbne.vi"("DATA"=u32 0, "ADDRESS"=u16 10) -> ()  [unwired: 1 out]
                                }
                              }
                            }
                          }
                        }
                        frame #2 {
                          n598 = call "wr_lbne.vi"("DATA"=w947, "ADDRESS"=u16 11) -> ()  [unwired: 1 out]
                        }
                        frame #3 {
                          # "write flash"
                          n599 = flat-sequence {
                            frame #0 {
                              n600 = call "wr_lbne.vi"("DATA"=u32 2, "ADDRESS"=u16 10) -> ()  [unwired: 1 out]
                            }
                            frame #1 {
                              n601 = while {
                                stop <- w953 continue-if-true
                                n602 = stacked-sequence {
                                tunnel: [_ _ w957 _] -> w952
                                frame #0 {
                                n603 = call "wr_lbne.vi"("DATA"=u32 258, "ADDRESS"=u16 10) -> ()  [unwired: 1 out]
                                }
                                frame #1 {
                                n604 = Wait Until Next ms Multiple(millisecond multiple=u32 1) -> ()  [unwired: 1 out]
                                }
                                frame #2 {
                                n605 = stacked-sequence {
                                tunnel: [_ _ w965] -> w957
                                frame #0 {
                                n606 = call "wr_lbne.vi"("DATA"=u32 5, "ADDRESS"=u16 10) -> ()  [unwired: 1 out]
                                }
                                frame #1 {
                                n607 = stacked-sequence {
                                frame #0 {
                                n608 = call "wr_lbne.vi"("DATA"=u32 261, "ADDRESS"=u16 10) -> ()  [unwired: 1 out]
                                }
                                frame #1 {
                                n609 = Wait Until Next ms Multiple(millisecond multiple=u32 1) -> ()  [unwired: 1 out]
                                }
                                frame #2 {
                                n610 = call "wr_lbne.vi"("DATA"=u32 5, "ADDRESS"=u16 10) -> ()  [unwired: 1 out]
                                }
                                }
                                }
                                frame #2 {
                                n611 = call "rd_lbne.vi"("ADDRESS 2"=i16 12) -> ("DATA 2"=w965:u32)
                                "DATA 6" <- w965
                                }
                                }
                                }
                                frame #3 {
                                n612 = call "wr_lbne.vi"("DATA"=u32 2, "ADDRESS"=u16 10) -> ()  [unwired: 1 out]
                                }
                                }
                                n613 = Equal?(x=w952, y=u32 3) -> (x = y?=w953:bool)
                              }
                            }
                          }
                        }
                        frame #4 {
                          n614 = stacked-sequence {
                            tunnel: [_ _ _ _ w977] -> w969
                            frame #0 {
                              w970 = u32 3  # opcode
                              n615 = call "wr_lbne.vi"("DATA"=w970, "ADDRESS"=u16 10) -> ()  [unwired: 1 out]
                            }
                            frame #1 {
                              w972 = u32 259  # opcode
                              n616 = call "wr_lbne.vi"("DATA"=w972, "ADDRESS"=u16 10) -> ()  [unwired: 1 out]
                            }
                            frame #2 {
                              w974 = u32 0  # opcode
                              n617 = call "wr_lbne.vi"("DATA"=w974, "ADDRESS"=u16 10) -> ()  [unwired: 1 out]
                            }
                            frame #3 {
                              n618 = Wait Until Next ms Multiple(millisecond multiple=u32 10) -> ()  [unwired: 1 out]
                            }
                            frame #4 {
                              n619 = for {
                                N: 4 -> [_]
                                shift-right: [w982] -> w977
                                shift-left: u32[] [] ("DATA") -> [w983]
                                i -> [w985]
                                n620 = Multiply(x=16, y=w985) -> (x*y=w986:i32)
                                n621 = Add(x=u32 128, y=w986) -> (x+y=w980:u32)
                                n622 = call "rd_lbne_BLK.vi"("ADDRESS 2"=w980) -> ("Array"=w981:u32[])
                                n623 = Build Array (concatenate)(w983, w981) -> (w982:u32[])
                              }
                            }
                          }
                        }
                        frame #5 {
                          n624 = Equal?(x=w990, y=w991) -> (x = y?=w988:bool)
                          "x = y?" <- w988
                          n625 = case shown="True" w988 {
                            tunnel: [TRUE ("x = y? 3") w995] -> w989
                            frame False {
                              n626 = local read "NUM ATTEMP"() -> (w994:i32)
                              n627 = Increment(x=w994) -> (x+1=w992:i32)
                              n628 = local write "NUM ATTEMP"(w992) -> ()
                            }
                            frame True {
                              n629 = local read "NUM ATTEMP"() -> (w998:i32)
                              n630 = local read "ONE_MORE"() -> (w997:i32)
                              n631 = Equal?(x=w998, y=w997) -> (x = y?=w996:bool)
                              n632 = case shown="True" w996 {
                                tunnel: [TRUE ("x = y? 3") w1004] -> w995
                                frame False {
                                n633 = local read "NUM ATTEMP"() -> (w1000:i32)
                                n634 = local write "ONE_MORE"(w1000) -> ()
                                }
                                frame True {
                                n635 = local write "ONE_MORE"(-1 ("ONE_MORE")) -> ()
                                n636 = local read "PAGE 3"() -> (w1008:i32)
                                n637 = Increment(x=w1008) -> (x+1=w1006:i32)
                                "PAGE 3" <- w1006
                                n638 = local read "Numeric"() -> (w1001:i32)
                                n639 = Equal?(x=w1006, y=w1001) -> (x = y?=w1005:bool)
                                n640 = Select(t=FALSE ("x = y? 3"), s=w1005, f=TRUE ("x = y? 3")) -> (s? t:f=w1004:bool)
                                "NUM ATTEMP" <- 0 ("NUM ATTEMP")
                                }
                              }
                            }
                          }
                          "WRITE ARRAY" <- w991
                          "READ ARRAY 2" <- w990
                        }
                      }
                      n641 = Multiply(x=100.0, y=w916) -> (x*y=→"Meter":dbl)
                      n642 = Not(x="STOP WRITE") -> (.not. x?=w910:bool)
                      n643 = And(x=w911, y=w910) -> (x .and. y?=w906:bool)
                    }
                  }
                }
              }
            }
          }
          frame "ASIC SPI" {
            n644 = Wait Until Next ms Multiple(millisecond multiple=u32 10) -> ()  [unwired: 1 out]
            n645 = case shown="True" "OK Button 2" {
              frame False {
              }
              frame True {
                n646 = flat-sequence {
                  frame #0 {
                    n647 = call "wr_lbne.vi"("DATA"=u16 1 ("ADDRESS"), "ADDRESS"=u16 1) -> ()  [unwired: 1 out]
                  }
                  frame #1 {
                    n648 = call "wr_lbne.vi"("DATA"=u16 2 ("ADDRESS"), "ADDRESS"=u16 1) -> ()  [unwired: 1 out]
                  }
                }
              }
            }
            n649 = stacked-sequence {
              tunnel: 8 ("NUMBER OF ASICS") -> [w1051 w1118]
              frame #0 {
                n650 = for {
                  N: w1051 -> [_]
                  shift-right: [w1053] -> w1049
                  shift-left: bool[] [] -> [w1056]
                  i -> [w1054]
                  n651 = Index Array(array="CHANNEL 3", index (col)=w1054) -> (element=w1091:T15)  [unwired: 1 in]
                  n652 = Reverse 1D Array(array=w1091) -> (reversed array=w1095:T15)
                  n653 = for {
                    tunnel: w1095 -> [w1109] mode=indexing
                    shift-right: [w1105] -> w1090
                    shift-left: bool[] [] -> [w1099]
                    n654 = Unbundle By Name(w1109) -> ("tst"=w1097:bool, "slp"=w1098:bool, "PDSR"=w1104:bool, "PCSR"=w1103:bool, "D_offset"=w1102:u16)
                    n655 = Number To Boolean Array(number=w1102) -> (Boolean array=w1108:bool[])
                    n656 = Array Subset(array=w1108, index=0, length=4) -> (w1101:bool[])
                    n657 = Reverse 1D Array(array=w1101) -> (reversed array=w1100:bool[])
                    n658 = Build Array (concatenate)(w1099, w1097, w1098, w1104, w1103, w1100) -> (w1105:bool[])
                  }
                  n659 = Unbundle By Name("Global1") -> ("F4"=w1065:u16, "F5"=w1064:u16, "sLSB"=w1063:u16, "RES4-0(binary)"=w1071:u16)
                  n660 = Unbundle By Name("Global0") -> ("CLKG"=w1086:u16, "FRQC"=w1089:u16, "EN_GR"=w1085:u16, "F0"=w1088:u16, "F1"=w1084:u16, "F2"=w1083:u16, "F3"=w1082:u16)
                  n661 = Not Equal To 0?(x=w1065) -> (x != 0?=w1066:bool)
                  n662 = Not Equal To 0?(x=w1064) -> (x != 0?=w1062:bool)
                  n663 = Not Equal To 0?(x=w1063) -> (x != 0?=w1061:bool)
                  n664 = Not Equal To 0?(x=w1088) -> (x != 0?=w1077:bool)
                  n665 = Not Equal To 0?(x=w1084) -> (x != 0?=w1076:bool)
                  n666 = Not Equal To 0?(x=w1083) -> (x != 0?=w1075:bool)
                  n667 = Not Equal To 0?(x=w1082) -> (x != 0?=w1074:bool)
                  n668 = Number To Boolean Array(number=w1071) -> (Boolean array=w1068:bool[])
                  n669 = Number To Boolean Array(number=w1086) -> (Boolean array=w1092:bool[])
                  n670 = Not Equal To 0?(x=w1089) -> (x != 0?=w1079:bool)
                  n671 = Not Equal To 0?(x=w1085) -> (x != 0?=w1078:bool)
                  n672 = Array Subset(array=w1068, index=0, length=5) -> (w1060:bool[])
                  n673 = Index Array(array=w1092, index=0) -> (element=w1081:bool)
                  n674 = Index Array(array=w1092, index=1) -> (element=w1080:bool)
                  n675 = Build Array (concatenate)(w1066, w1062, w1061, w1060) -> (w1067:bool[])
                  n676 = Build Array(w1081, w1080, w1079, w1078, w1077, w1076, w1075, w1074) -> (w1073:bool[])
                  n677 = Reverse 1D Array(array=w1067) -> (reversed array=w1058:bool[])
                  n678 = Reverse 1D Array(array=w1073) -> (reversed array=w1059:bool[])
                  n679 = Build Array (concatenate)(w1090, w1058, w1059) -> (w1055:bool[])
                  n680 = Build Array (concatenate)(w1056, w1055) -> (w1053:bool[])
                }
                "ADC ARRAY" <- w1049
                n681 = Array Size(array=w1049) -> (size(s)=→"size(s)":i32)
              }
              frame #1 {
                n682 = Select(t=bool[] [], s="FE ASIC(DAC)", f=bool[] [FALSE, FALSE, FALSE, FALSE, FALSE, FALSE, FALSE, FALSE, FALSE, FALSE, FALSE, FALSE, FALSE, FALSE, FALSE, FALSE, FALSE, FALSE, FALSE, FALSE, FALSE, FALSE, FALSE, FALSE, FALSE, FALSE, FALSE, FALSE, FALSE, FALSE, FALSE, FALSE, FALSE, FALSE, FALSE, FALSE, FALSE, FALSE, FALSE, FALSE, FALSE, FALSE, FALSE, FALSE, FALSE, FALSE, FALSE, FALSE, FALSE, FALSE, FALSE, FALSE, FALSE, FALSE, FALSE, FALSE, FALSE, FALSE, FALSE, FALSE, FALSE, FALSE, FALSE, FALSE]) -> (s? t:f=w1113:bool[])
                n683 = for {
                  N: w1118 -> [_]
                  shift-right: [w1134] -> w1117
                  shift-left: w1113 -> [w1132]
                  tunnel: "FE ASIC(DAC)" -> [w1128]
                  tunnel: "DAC" -> [w1123] mode=indexing
                  tunnel: "SW" -> [w1122] mode=indexing
                  i -> [w1131]
                  w1129 = FALSE ("SLK 2")
                  n684 = Select(t="DAC  0x00-0x3f", s="DAC QUICK SET", f=w1123) -> (s? t:f=w1125:u16)
                  n685 = Index Array(array="Array 3", index (col)=w1131) -> (element=w1135:T16)  [unwired: 1 in]
                  n686 = Select(t="DAC SW", s="DAC QUICK SET", f=w1122) -> (s? t:f=w1119:u16)
                  n687 = for {
                    tunnel: w1135 -> [w1175] mode=indexing
                    shift-right: [w1171] -> w1142
                    shift-left: bool[] [] -> [w1172]
                    n688 = Unbundle By Name(w1175) -> ("sts"=w1174:bool, "snc"=w1173:bool, "SG"=w1164:u16, "ST"=w1163:u16, "SDC"=w1160:bool, "SDF"=w1159:bool)
                    n689 = Number To Boolean Array(number=w1164) -> (Boolean array=w1170:bool[])
                    n690 = Number To Boolean Array(number=w1163) -> (Boolean array=w1165:bool[])
                    n691 = Array Subset(array=w1170, index=0, length=2) -> (w1162:bool[])
                    n692 = Array Subset(array=w1165, index=0, length=2) -> (w1161:bool[])
                    n693 = Build Array (concatenate)(w1172, w1174, w1173, w1162, w1161, w1160, w1159) -> (w1171:bool[])
                  }
                  n694 = case shown="True" w1128 {
                    tunnel: [bool[] [] w1149] -> w1126
                    tunnel: w1125 -> [_ w1148]
                    tunnel: w1119 -> [_ w1147]
                    frame False {
                    }
                    frame True {
                      n695 = Number To Boolean Array(number=w1148) -> (Boolean array=w1158:bool[])
                      n696 = Number To Boolean Array(number=w1147) -> (Boolean array=w1154:bool[])
                      n697 = Array Subset(array=w1158, index=0, length=6) -> (w1155:bool[])
                      n698 = Reverse 1D Array(array=w1155) -> (reversed array=w1150:bool[])
                      n699 = Array Subset(array=w1154, index=0, length=2) -> (w1151:bool[])
                      n700 = Build Array (concatenate)(w1151, w1150) -> (w1149:bool[])
                      "DAC  0x00-0x3f" <- w1148
                    }
                  }
                  "array" <- w1126
                  n701 = Number To Boolean Array(number="STB") -> (Boolean array=w1138:bool[])
                  n702 = Array Subset(array=w1138, index=0, length=2) -> (w1144:bool[])
                  n703 = Reverse 1D Array(array=w1142) -> (reversed array=w1127:bool[])
                  n704 = Reverse 1D Array(array=w1144) -> (reversed array=w1145:bool[])
                  n705 = Build Array (concatenate)(w1127, "SLK", w1145, w1129, "SLK 2", w1129, w1129, w1129, w1126) -> (w1133:bool[])
                  n706 = Build Array (concatenate)(w1132, w1133) -> (w1134:bool[])
                }
                "FE ARRAY" <- w1117
                n707 = Array Size(array=w1117) -> (size(s)=→"size(s) 2":i32)
              }
            }
            n708 = event shown="[0] Timeout" {
              selector: _ -> [_ _ _]
              dyn-events: _ -> [_ _ _]
              timeout: 100 -> [_ _ _]
              event Timeout {
                n709 = event-data() -> ()  [unwired: 1 in, 3 out]
              }
              event "Slide": Value Change {
                n710 = event-data() -> ()  [unwired: 1 in, 4 out]
                n711 = Build Array("Slide") -> (w1177:u8[])
                n712 = Build Array(u8 0 ("element"), "Slide") -> (w1178:u8[])
                n713 = property on="Array 3" class="Arr"("Index Values"=w1178) -> ()  [unwired: 2 in, 2 out]
                n714 = property on="Array 4" class="Arr (strict)"("Index Values"=w1177) -> ()  [unwired: 2 in, 2 out]
                n715 = property on="CHANNEL 3" class="Arr (strict)"("Index Values"=w1178) -> ()  [unwired: 2 in, 2 out]
              }
              event "QUICK SET": Value Change {
                n716 = event-data() -> ()  [unwired: 1 in, 6 out]
                n717 = case shown="True" "ALL SET" {
                  tunnel: [1 8] -> w1181
                  frame False {
                  }
                  frame True {
                  }
                }
                n718 = for {
                  N: w1181 -> [_]
                  tunnel: "ALL SET" -> [w1201]
                  i -> [w1200]
                  n719 = case shown="False" w1201 {
                    tunnel: [w1219 w1220] -> w1193
                    tunnel: w1200 -> [_ w1220]
                    frame False {
                      n720 = local read "Slide"() -> (w1219:u8)
                    }
                    frame True {
                    }
                  }
                  n721 = local read "CHANNEL 3"() -> (w1206:T5)
                  n722 = local read "Array 3"() -> (w1203:T6)
                  n723 = Index Array(array=w1203, index (col)=w1193) -> (element=w1202:T16)  [unwired: 1 in]
                  n724 = Index Array(array=w1206, index (col)=w1193) -> (element=w1205:T15)  [unwired: 1 in]
                  n725 = for {
                    tunnel: w1205 -> [w1270] mode=indexing
                    tunnel: "CHANNEL 4" -> [w1272]
                    tunnel: [w1271] -> w1194 mode=indexing
                    tunnel: w1205 -> [w1269] mode=indexing
                    tunnel: "channel" -> [w1253]
                    tunnel: w1202 -> [w1252] mode=indexing
                    tunnel: w1202 -> [w1251] mode=indexing
                    tunnel: [w1226] -> w1195 mode=indexing
                    n726 = Unbundle By Name(w1272) -> ("D_offset"=w1262:u16, "PDSR"=w1261:bool, "PCSR"=w1259:bool, "slp"=w1258:bool, "tst"=w1222:bool)
                    n727 = Unbundle By Name(w1269) -> ("D_offset"=w1265:u16, "PDSR"=w1264:bool, "PCSR"=w1260:bool, "slp"=w1263:bool, "tst"=w1223:bool)
                    n728 = Unbundle By Name(w1253) -> ("sts"=w1238:bool, "snc"=w1237:bool, "SG"=w1236:u16, "ST"=w1235:u16, "SDC"=w1234:bool, "SDF"=w1233:bool)
                    n729 = Unbundle By Name(w1252) -> ("sts"=w1250:bool, "snc"=w1249:bool, "SG"=w1248:u16, "ST"=w1247:u16, "SDC"=w1246:bool, "SDF"=w1245:bool)
                    n730 = Select(t=w1238, s="s 5", f=w1250) -> (s? t:f=w1227:bool)
                    n731 = Select(t=w1237, s="s 6", f=w1249) -> (s? t:f=w1228:bool)
                    n732 = Select(t=w1236, s="s 7", f=w1248) -> (s? t:f=w1229:u16)
                    n733 = Select(t=w1235, s="s 8", f=w1247) -> (s? t:f=w1230:u16)
                    n734 = Select(t=w1234, s="s 9", f=w1246) -> (s? t:f=w1231:bool)
                    n735 = Select(t=w1233, s="s 10", f=w1245) -> (s? t:f=w1232:bool)
                    n736 = Select(t=w1262, s="s", f=w1265) -> (s? t:f=w1268:u16)
                    n737 = Select(t=w1261, s="s 2", f=w1264) -> (s? t:f=w1267:bool)
                    n738 = Select(t=w1259, s="s 3", f=w1260) -> (s? t:f=w1266:bool)
                    n739 = Select(t=w1258, s="s 4", f=w1263) -> (s? t:f=w1225:bool)
                    n740 = Select(t=w1222, s="s 11", f=w1223) -> (s? t:f=w1224:bool)
                    n741 = Bundle By Name(cluster=w1270, "D_offset"=w1268, "PDSR"=w1267, "PCSR"=w1266, "slp"=w1225, "tst"=w1224) -> (w1271:T4)
                    n742 = Bundle By Name(cluster=w1251, "sts"=w1227, "snc"=w1228, "SG"=w1229, "ST"=w1230, "SDC"=w1231, "SDF"=w1232) -> (w1226:T3)
                  }
                  n743 = Unbundle By Name("channel") -> ("SG"=w1190:u16, "ST"=w1187:u16)
                  n744 = case shown="2" w1190 {
                    tunnel: [u16 446 ("SG") u16 265 ("SG") u16 148 ("SG") u16 81 ("SG")] -> w1191
                    frame 0, Default {
                    }
                    frame 1 {
                    }
                    frame 2 {
                    }
                    frame 3 {
                    }
                  }
                  "gain electrons" <- w1191
                  n745 = case shown="3" w1190 {
                    tunnel: [u16 47 ("SG") u16 78 ("SG") u16 14 ("SG") u16 25 ("SG")] -> w1189
                    frame 0, Default {
                    }
                    frame 1 {
                    }
                    frame 2 {
                    }
                    frame 3 {
                    }
                  }
                  n746 = case shown="0, Default" w1187 {
                    tunnel: [u16 1 ("SG") u16 0 ("SG") u16 3 ("SG") u16 2 ("SG")] -> w1186
                    frame 0, Default {
                    }
                    frame 1 {
                    }
                    frame 2 {
                    }
                    frame 3 {
                    }
                  }
                  n747 = Multiply(x=w1189, y=u16 10) -> (x*y=w1185:u16)
                  n748 = local read "CHANNEL 3"() -> (w1196:T5)
                  n749 = local read "Array 3"() -> (w1198:T6)
                  n750 = Add(x=w1186, y=w1185) -> (x+y=→"setting":u16)
                  n751 = Replace Array Subset(array=w1198, new element=w1195, index (col)=w1193) -> (w1199:T6)  [unwired: 1 in]
                  n752 = Replace Array Subset(array=w1196, new element=w1194, index (col)=w1193) -> (w1197:T5)  [unwired: 1 in]
                  n753 = local write "Array 3"(w1199) -> ()
                  n754 = local write "CHANNEL 3"(w1197) -> ()
                }
              }
            }
            n755 = case shown="True" "write_string" {
              frame False {
              }
              frame True {
                n756 = stacked-sequence {
                  frame #0 {
                    n757 = local read "ADC write"() -> (w1277:bool)
                    n758 = case shown="True" w1277 {
                      frame False {
                      }
                      frame True {
                        # "ADC ASIC"
                        n759 = stacked-sequence {
                          frame #0 {
                            n760 = local read "ADC ARRAY"() -> (w1286:bool[])
                            n761 = Array Size(array=w1286) -> (size(s)=w1285:i32)
                            n762 = local read "ADC ARRAY"() -> (w1283:bool[])
                            n763 = Divide(x=w1285, y=2) -> (x/y=w1278:dbl)
                            n764 = Array Subset(array=w1283, index=w1278) -> (w1281:bool[])  [unwired: 1 in]
                            n765 = Array Subset(array=w1286, length=w1278) -> (w1282:bool[])  [unwired: 1 in]
                            n766 = for {
                              N: 36 -> [_]
                              tunnel: w1282 -> [w1301]
                              tunnel: w1281 -> [w1299]
                              tunnel: [w1288] -> w1279 mode=indexing
                              i -> [w1290]
                              (unwired) 64 ("y")
                              w1300 = 16 ("length")
                              n767 = Multiply(x=w1300, y=w1290) -> (x*y=w1297:i32)
                              n768 = Add(x=w1290, y=512) -> (x+y=w1287:i32)
                              n769 = Array Subset(array=w1301, index=w1297, length=w1300) -> (w1293:bool[])
                              n770 = Array Subset(array=w1299, index=w1297, length=16) -> (w1294:bool[])
                              n771 = Boolean Array To Number(Boolean array=w1293) -> (number=w1295:u32)
                              n772 = To Unsigned Word Integer(number=w1295) -> (unsigned 16bit integer=w1292:u16)
                              n773 = Boolean Array To Number(Boolean array=w1294) -> (number=w1296:u32)
                              n774 = To Unsigned Word Integer(number=w1296) -> (unsigned 16bit integer=w1291:u16)
                              n775 = Join Numbers(hi=w1291, lo=w1292) -> ((hi.lo)=w1288:u32)
                              n776 = call "wr_lbne.vi"("DATA"=w1288, "ADDRESS"=w1287) -> ()  [unwired: 1 out]
                            }
                            "Array" <- w1279
                            "ADC  Input" <- w1279
                          }
                          frame #1 {
                            n777 = flat-sequence {
                              frame #0 {
                                n778 = call "wr_lbne.vi"("DATA"=u32 1, "ADDRESS"=u16 2) -> ()  [unwired: 1 out]
                              }
                              frame #1 {
                                n779 = Wait Until Next ms Multiple(millisecond multiple=u32 10) -> ()  [unwired: 1 out]
                              }
                              frame #2 {
                                n780 = for {
                                N: 36 -> [_]
                                tunnel: [w1310] -> w1307 mode=indexing
                                i -> [w1312]
                                (unwired) 104 ("y")
                                n781 = Add(x=w1312, y=552) -> (x+y=w1311:i32)
                                n782 = call "rd_lbne.vi"("ADDRESS 2"=w1311) -> ("DATA 2"=w1310:u32)
                                n783 = Wait Until Next ms Multiple(millisecond multiple=u32 1) -> ()  [unwired: 1 out]
                                }
                                "ADC RB" <- w1307
                                n784 = local read "Array"() -> (w1306:u32[])
                                n785 = Equal?(x=w1307, y=w1306) -> (x = y?=→"ADC SPI OK":bool)
                              }
                            }
                          }
                        }
                      }
                    }
                  }
                  frame #1 {
                    # "FE ASIC"
                    n786 = stacked-sequence {
                      frame #0 {
                        n787 = local read "FE ARRAY"() -> (w1321:bool[])
                        n788 = Array Size(array=w1321) -> (size(s)=w1320:i32)
                        n789 = Divide(x=w1320, y=2) -> (x/y=w1318:dbl)
                        n790 = Array Subset(array=w1321, index=w1318) -> (w1315:bool[])  [unwired: 1 in]
                        n791 = Array Subset(array=w1321) -> (w1316:bool[])  [unwired: 2 in]
                        n792 = for {
                          N: 36 -> [_]
                          tunnel: w1316 -> [w1336]
                          tunnel: w1315 -> [w1334]
                          tunnel: [w1323] -> w1314 mode=indexing
                          i -> [w1324]
                          (unwired) 64 ("y")
                          w1335 = 16 ("length")
                          n793 = Multiply(x=w1335, y=w1324) -> (x*y=w1332:i32)
                          n794 = Array Subset(array=w1336, index=w1332, length=w1335) -> (w1328:bool[])
                          n795 = Array Subset(array=w1334, index=w1332, length=16) -> (w1329:bool[])
                          n796 = Boolean Array To Number(Boolean array=w1328) -> (number=w1330:u32)
                          n797 = Boolean Array To Number(Boolean array=w1329) -> (number=w1331:u32)
                          n798 = To Unsigned Word Integer(number=w1330) -> (unsigned 16bit integer=w1327:u16)
                          n799 = To Unsigned Word Integer(number=w1331) -> (unsigned 16bit integer=w1326:u16)
                          n800 = Add(x=w1324, y=592) -> (x+y=w1325:i32)
                          n801 = Join Numbers(hi=w1326, lo=w1327) -> ((hi.lo)=w1323:u32)
                          n802 = call "wr_lbne.vi"("DATA"=w1323, "ADDRESS"=w1325) -> ()  [unwired: 1 out]
                        }
                        "Array 2" <- w1314
                        "FE Input" <- w1314
                      }
                      frame #1 {
                        n803 = flat-sequence {
                          frame #0 {
                            n804 = call "wr_lbne.vi"("DATA"=u32 2, "ADDRESS"=u16 2) -> ()  [unwired: 1 out]
                          }
                          frame #1 {
                            n805 = Wait Until Next ms Multiple(millisecond multiple=u32 10) -> ()  [unwired: 1 out]
                          }
                          frame #2 {
                            n806 = for {
                              N: 36 -> [_]
                              tunnel: [w1346] -> w1341 mode=indexing
                              i -> [w1348]
                              (unwired) 104 ("y")
                              n807 = Add(x=w1348, y=632) -> (x+y=w1347:i32)
                              n808 = call "rd_lbne.vi"("ADDRESS 2"=w1347) -> ("DATA 2"=w1346:u32)
                              n809 = Wait Until Next ms Multiple(millisecond multiple=u32 1) -> ()  [unwired: 1 out]
                            }
                            "FE RB" <- w1341
                            n810 = local read "Array 2"() -> (w1340:u32[])
                            n811 = Equal?(x=w1341, y=w1340) -> (x = y?=→"FE SPI OK":bool)
                          }
                        }
                      }
                    }
                  }
                  frame #2 {
                    n812 = case shown="True" "ADC write" {
                      frame False {
                      }
                      frame True {
                        n813 = call "rd_lbne.vi"("ADDRESS 2"=i16 6) -> ("DATA 2"=w1354:u32)
                        n814 = Split Number(x=w1354) -> (hi(x)=→"ADC FIFO SYNC":u16)  [unwired: 1 out]
                      }
                    }
                    n815 = case shown="True" "Sync_cnt" {
                      frame False {
                      }
                      frame True {
                        n816 = call "wr_lbne.vi"("DATA"=u32 1, "ADDRESS"=u16 18) -> ()  [unwired: 1 out]
                      }
                    }
                  }
                }
              }
            }
          }
        }
      }
    }
    frame #2 {
      n817 = flat-sequence {
        frame #0 {
          n818 = global read "LBNE_Global .vi" "LBNE_REF"() -> (w1358:refnum<k24>)
          n819 = invoke class="LBNE_COMM" method="UDP_CLEANUP"(reference=w1358) -> ("UDP_CLEANUP"=→"UDP_CLEANUP":string)  [unwired: 2 in, 2 out]
        }
        frame #1 {
          n820 = Wait Until Next ms Multiple(millisecond multiple=u32 1200) -> ()  [unwired: 1 out]
        }
        frame #2 {
        }
        frame #3 {
        }
      }
      n821 = Request Deallocation(TRUE ("flag")) -> ()
    }
  }
